vi "Auto_New.vi"() -> ()   [LabVIEW 2017]
uses:
  Control/Saurabh/prosucer_consumer_enum1.ctl
  <vilib>/Utility/error.llb/DialogType.ctl
  <vilib>/addons/database/Connection.llb/DB Tools Open Connec (String).vi
  Global/Global 1.vi
  Global/DATA LOG.vi
  <vilib>/addons/database/NI_Database_API.lvlib
panel:
  out "OP30 BARCODE STRING EMPRTY 2":bool
  out "SHIFT":string
  in  "BARCODE RECIPE":string(combo)
  out "PLC COM.":bool
  out "SHIFT_DATA":string[](array[string])
  out "OP30 BARCODE STRING EMPRTY":bool
  out "stop":bool
  out "error out 2":errorcluster
  out "Shift 4":i32
  out "Time Stamp Out":timestamp[](array[timestamp]) format="%<%X>T"
  out "Time Stamp Out 4":timestamp[](array[timestamp]) format="%<%X>T"
  out "Shift_change":bool
  out "appended array":string[][](array[string])
  out "SHIFT_DATA 2":string[](array[string])
  in  "error in (no error)":errorcluster
  in  "Tab Control":enum32{"Screen 1", "Screen 2"}(tab)
  out "OP 50":bool
  out "OP 40":bool
  out "OP 30":bool
  out "OP - 50":T1
  out "OP - 40":T2
  out "OP - 30":T3
  in  "stop 2":bool
  out "OP - 10":T4
  in  "SIMULATE INPUT":bool[](array[boolean])=[FALSE, FALSE, FALSE, FALSE]
  out "OP - 20":T5
  out "OP 10 & 20":bool
  out "OP - 110":cluster{"BARCODE":string}
  out "OP - 80":T6
  out "OP - 70":T7
  out "OP - 90":T8
  out "OP - 100":T9
  out "OP - 60":T10
  out "OP 60":bool
  out "OP 70 & 80":bool
  out "OP 90 -100 - 110":bool
  # "SENSOR MIN VLTG"
  # "Op10 20\nOp30\nOp 40\nOp50\nOp60\nOp70-80\nOp 90-100-110"
  # "OP - 50"
  # "OP - 40"
  # "OP - 30"
  # "OP - 10"
  # "OP - 20"
  # "Op10 20\nOp30\nOp 40\nOp50\nOp60\nOp70-80\nOp 90-100-110"
  # "OP - 110"
  # "OP - 80"
  # "OP - 70"
  # "OP - 90"
  # "OP - 100"
  # "OP - 60"
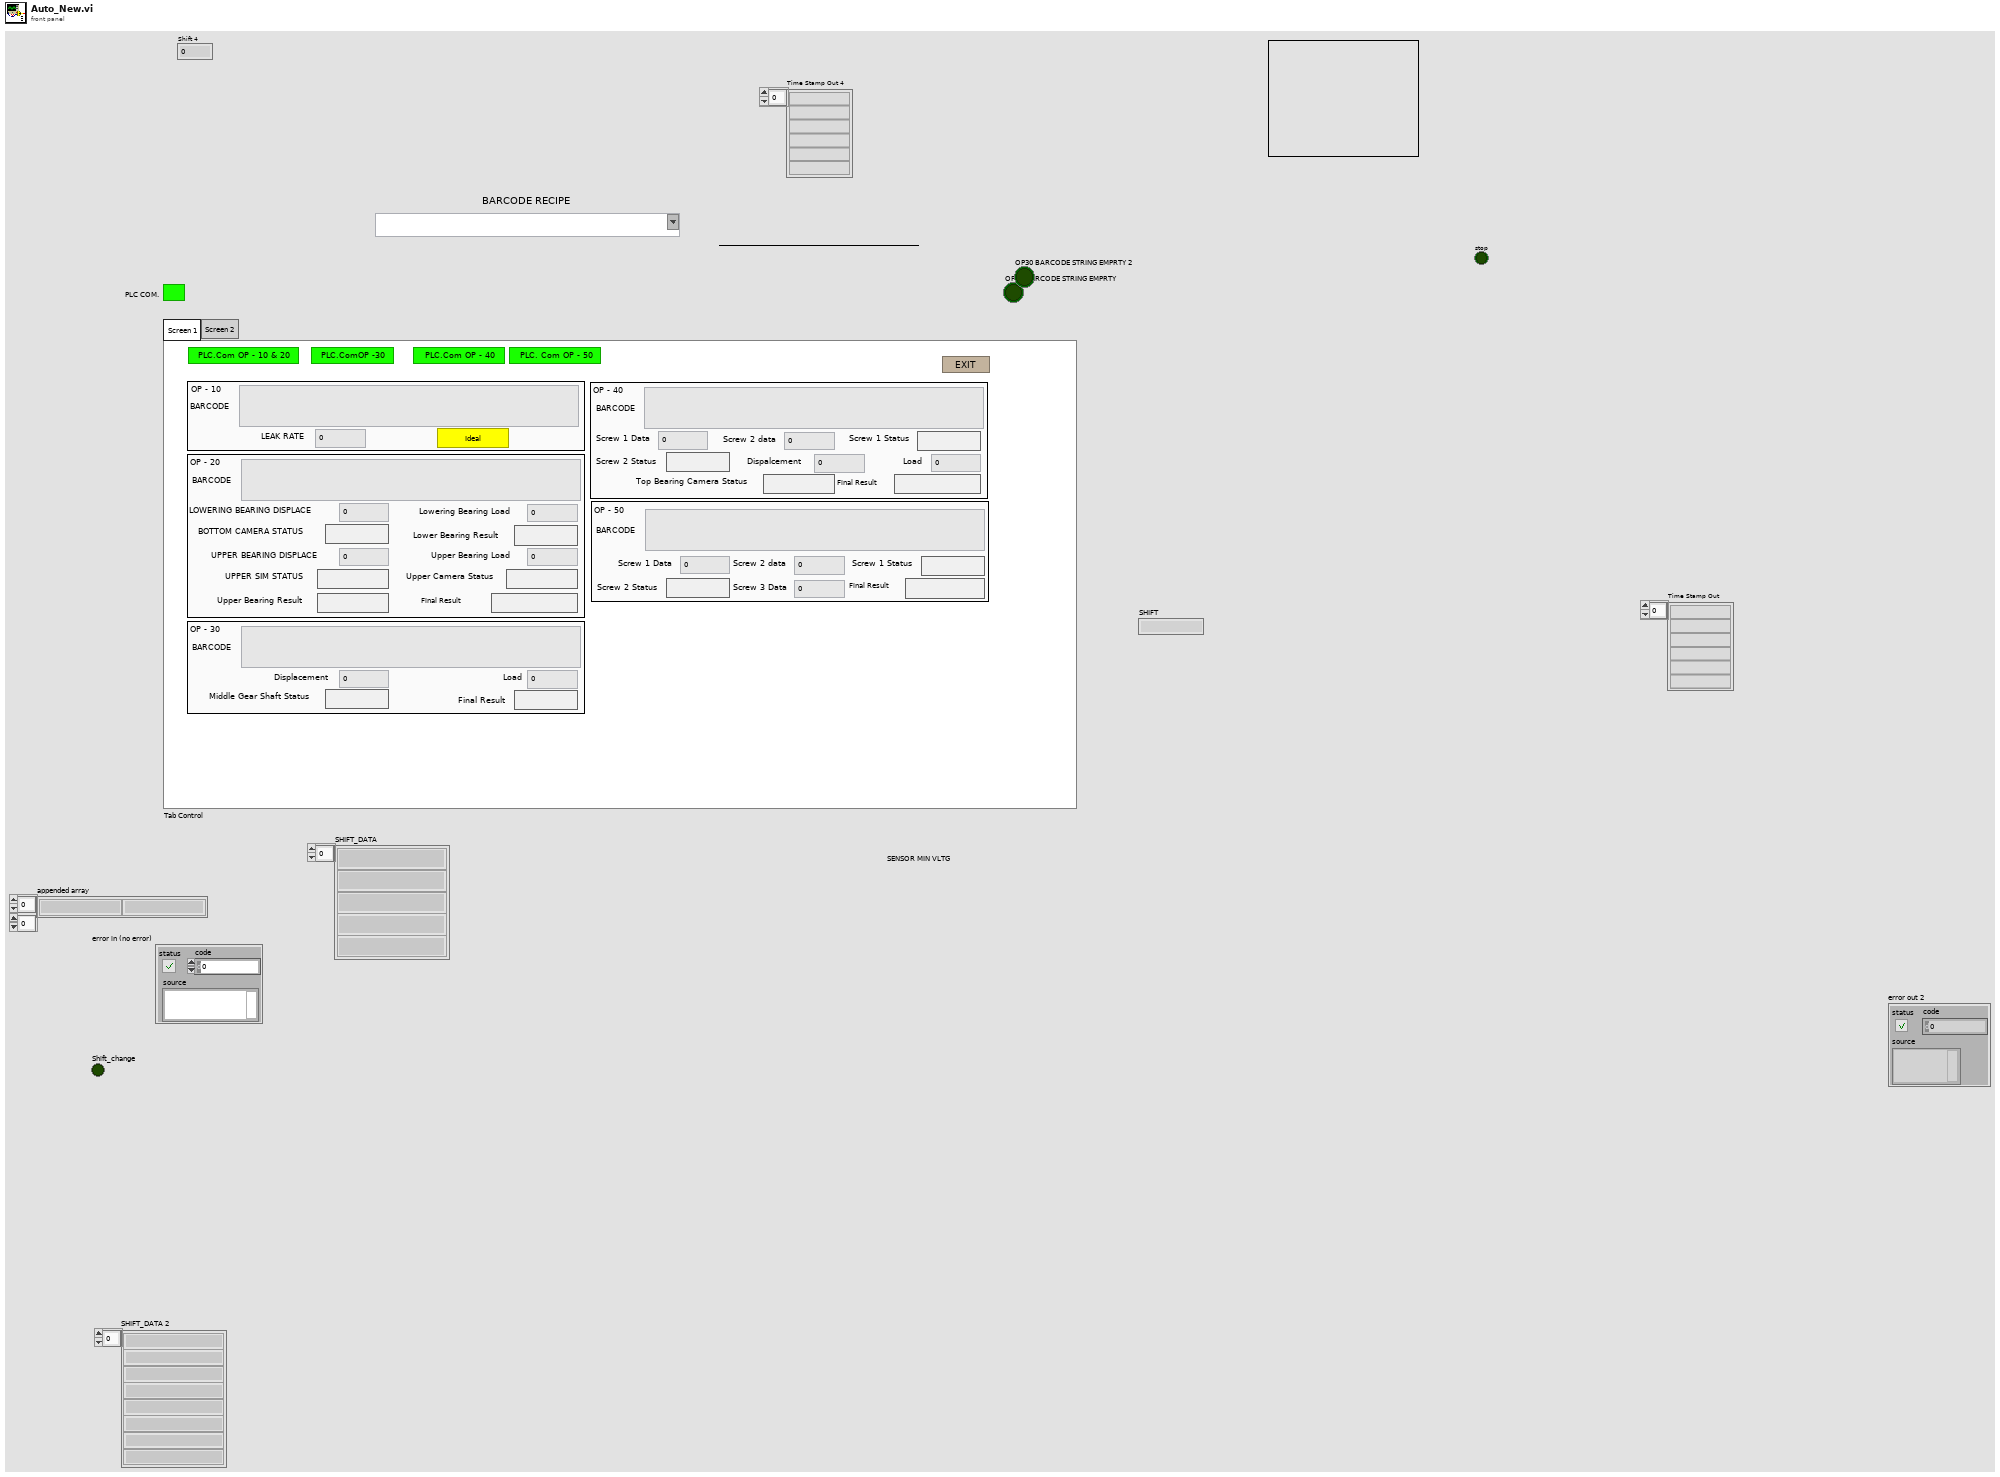
[diagram p1: front panel]
types:
  T1 = cluster{"BARCODE":string, "Screw 1 Data":dbl, "Screw 2 data":dbl, "Screw 1 Status":bool, "Screw 2 Status":bool, "Screw 3 Data":dbl, "Final Result":bool}
  T2 = cluster{"BARCODE":string, "Screw 1 Data":dbl, "Screw 2 data":dbl, "Screw 1 Status":bool, "Screw 2 Status":bool, "Dispalcement ":dbl, "Load ":dbl, "Top Bearing Camera Status":bool, "Final Result":bool}
  T3 = cluster{"BARCODE":string, "Displacement":dbl, "Load":dbl, "Middle Gear Shaft Status":bool, "Final Result":bool}
  T4 = cluster{"BARCODE":string, "LEAK RATE":dbl, "RESULT":bool}
  T5 = cluster{"BARCODE":string, "LOWERING BEARING DISPLACE":dbl, "Lowering Bearing Load":dbl, "BOTTOM CAMERA STATUS":bool, "Lower Bearing Result":bool, "UPPER BEARING DISPLACE":dbl, "Upper Bearing Load ":dbl, "UPPER SIM STATUS":bool, "Upper Camera Status":bool, "Upper Bearing Result":bool, "Final Result":bool}
  T6 = cluster{"BARCODE":string, "Load":dbl, "Final Result":bool, "Dispensing":bool}
  T7 = cluster{"BARCODE":string, "Sensor MIN Vltg":dbl, "Sensor MAX Vltg":dbl, "Final Result":bool}
  T8 = cluster{"BARCODE":string, "Seat LT Data":dbl, "Seat Status":bool, "Steam LT Data":dbl, "Final Result":bool}
  T9 = cluster{"BARCODE":string, "Sensor O/P Open V":dbl, "Start Of Close Sensor V":dbl, "Final Result":bool, "Sensor O/P Full Close V":dbl, "Response Time FWD (mSec)":dbl, "Response Time REV (mSec)":dbl, "Motor V Start Of Close A":dbl, "Motor V Full Close B R":dbl, "Motor V Start Back C":dbl, "Motor V Full Open D":dbl, "Motor RMS Current A":dbl}
  T10 = cluster{"BARCODE":string, "Screw 1 Data":dbl, "Screw 2 data":dbl, "Screw 1 Status":bool, "Screw 2 Status":bool, "Screw3 Data":dbl, "Final Result":bool, "Screw3 Status":bool, "Screw4 Data":dbl, "Screw5 Data":dbl, "Screw4 Status":bool, "Screw5 Status":bool, "Screw6 Data":dbl, "Screw6 Status":bool}
  T11 = cluster{"OP - 10":cluster{"BARCODE":string, "LEAK RATE":dbl, "RESULT":bool}, "OP - 20":cluster{"BARCODE":string, "LOWERING BEARING DISPLACE":dbl, "LOWERING BEARING LOAD":dbl, "BOTTOM CAMERA STATUS":bool, "LOWER BEARING RESULT":bool, "UPPER BEARING DISPLACE":dbl, "UPPER BEARING LOAD ":dbl, "UPPER SIM STATUS":bool, "UPPER CAMERA STATUS":bool, "UPPER BEARING RESULT":bool, "FINAL RESULT":bool}, "OP - 30":cluster{"BARCODE":string, "Displacement":dbl, "Load":dbl, "Middle Gear Shaft Status":bool, "Final Result":bool}, "OP - 40":cluster{"BARCODE":string, "Screw 1 Data":dbl, "Screw 2 data":dbl, "Screw 1 Status":bool, "Screw 2 Status":bool, "Dispalcement ":dbl, "Load ":dbl, "Top Bearing Camera Status":bool, "Final Result":bool}, "OP - 50":cluster{"BARCODE":string, "Screw 1 Data":dbl, "Screw 2 data":dbl, "Screw 1 Status":bool, "Screw 2 Status":bool, "Screw 3 Data":dbl, "Final Result":bool}, "OP - 60":cluster{"BARCODE":string, "Screw 1 Data":dbl, "Screw 2 data":dbl, "Screw 1 Status":bool, "Screw 2 Status":bool, "Screw3 Data":dbl, "Final Result":bool, "Screw3 Status":bool, "Screw4 Data":dbl, "Screw5 Data":dbl, "Screw4 Status":bool, "Screw5 Status":bool, "Screw6 Data":dbl, "Screw6 Status":bool}, "OP - 70":cluster{"BARCODE":string, "Sensor MIN Vltg":dbl, "Sensor MAX Vltg":dbl, "Final Result":bool}, "OP - 80":cluster{"BARCODE":string, "Load":dbl, "Final Result":bool, "Dispensing":bool}, "OP - 90":cluster{"BARCODE":string, "Seat LT Data":dbl, "Seat Status":bool, "Steam LT Data":dbl, "Final Result":bool}, "OP - 100":cluster{"BARCODE":string, "Sensor O/P Open V":dbl, "Start Of Close Sensor V":dbl, "Final Result":bool, "Sensor O/P Full Close V":dbl, "Response Time FWD (mSec)":dbl, "Response Time REV (mSec)":dbl, "Motor V Start Of Close A":dbl, "Motor V Full Close B R":dbl, "Motor V Start Back C":dbl, "Motor V Full Open D":dbl, "Motor RMS Current A":dbl}, "OP - 110":cluster{"BARCODE":string}}
  T12 = typedef "prosucer_consumer_enum1.ctl" = enum16{"SCAN1", "SCAN2", "SCAN3", "SCAN4", "SCAN5", "SCAN6", "SCAN7", "SCAN8", "SCAN9", "SCAN10", "SCAN11", "STOP", "DATALOG1", "DATALOG2", "DATALOG3", "DATALOG4", "DATALOG5", "DATALOG6", "DATALOG7", "DATALOG8", "DATALOG9", "DATALOG10", "DATALOG11", "-1", "CYCLE_START1", "CYCLE_START2", "CYCLE_START3", "CYCLE_START4", "BARCODE RECIPE", "EMERGENCY STOP"}
  T13 = typedef "NI_Database_API.lvlib/Conn ObjectReference.ctl" = refnum<k1>
  T14 = typedef "DialogType.ctl" = u16
  T15 = cluster{"trimmed string":string, "SHIFT":string, "date/time string":string, string, "Input 2":string}
  T16 = cluster{"SHIFT":string, "date/time string":string, "Input 2":string, string}
  T17 = cluster{"Input 2":string, "Input 2":string, "Input 2":string, "Input 2":string, "Input 2":string, "Input 2":string, "Input 2":string, "Input 2":string, "Input 2":string, "Input 2":string}
  T18 = cluster{"date/time string":string, "SHIFT":string, "Input 2":string, "Input 2":string, "Input 2":string, "Input 2":string, "Input 2":string, "Input 2":string, "Input 2":string, "Input 2":string, "Input 2":string, "Input 2":string}
  T19 = cluster{"Input 2":string, "Input 2":string, "Input 2":string, "Input 2":string}
  T20 = cluster{"date/time string":string, "SHIFT":string, "Input 2":string, "Input 2":string, "Input 2":string, "Input 2":string}
  T21 = cluster{"Input 2":string, "Input 2":string, "Input 2":string, "Input 2":string, "Input 2":string, "Input 2":string, "Input 2":string, "Input 2":string}
  T22 = cluster{"date/time string":string, "SHIFT":string, "Input 2":string, "Input 2":string, "Input 2":string, "Input 2":string, "Input 2":string, "Input 2":string, "Input 2":string, "Input 2":string}
  T23 = cluster{"Input 2":string, "Input 2":string, "Input 2":string, "Input 2":string, "Input 2":string, "Input 2":string}
  T24 = cluster{"date/time string":string, "SHIFT":string, "Input 2":string, "Input 2":string, "Input 2":string, "Input 2":string, "Input 2":string, "Input 2":string}
  T25 = cluster{"Input 2":string, "Input 2":string, "Input 2":string, "Input 2":string, "Input 2":string, "Input 2":string, "Input 2":string, "Input 2":string, "Input 2":string, "Input 2":string, "Input 2":string, "Input 2":string}
  T26 = cluster{"date/time string":string, "SHIFT":string, "Input 2":string, "Input 2":string, "Input 2":string, "Input 2":string, "Input 2":string, "Input 2":string, "Input 2":string, "Input 2":string, "Input 2":string, "Input 2":string, "Input 2":string, "Input 2":string}
  T27 = cluster{"Input 2":string, "Input 2":string, "Input 2":string}
  T28 = cluster{"date/time string":string, "SHIFT":string, "Input 2":string, "Input 2":string, "Input 2":string}
  T29 = cluster{"Input 2":string, "Input 2":string, "Input 2":string, "time string":string, "time string":string, "Input 2":string, "Input 2":string, "Input 2":string, "Input 2":string, "Input 2":string, "Input 2":string, "Input 2":string}
  T30 = cluster{"date/time string":string, "SHIFT":string, "Input 2":string, "Input 2":string, "Input 2":string, "time string":string, "time string":string, "Input 2":string, "Input 2":string, "Input 2":string, "Input 2":string, "Input 2":string, "Input 2":string, "Input 2":string}
  T31 = cluster{"BARCODE":string, "LOWERING BEARING DISPLACE":dbl, "LOWERING BEARING LOAD":dbl, "BOTTOM CAMERA STATUS":bool, "LOWER BEARING RESULT":bool, "UPPER BEARING DISPLACE":dbl, "UPPER BEARING LOAD ":dbl, "UPPER SIM STATUS":bool, "UPPER CAMERA STATUS":bool, "UPPER BEARING RESULT":bool, "FINAL RESULT":bool}
  T32 = enum32{"invalid app kind", "Development System", "Run Time System", "Student Edition", "Embedded LabVIEW", "Evaluation", "Custom"}
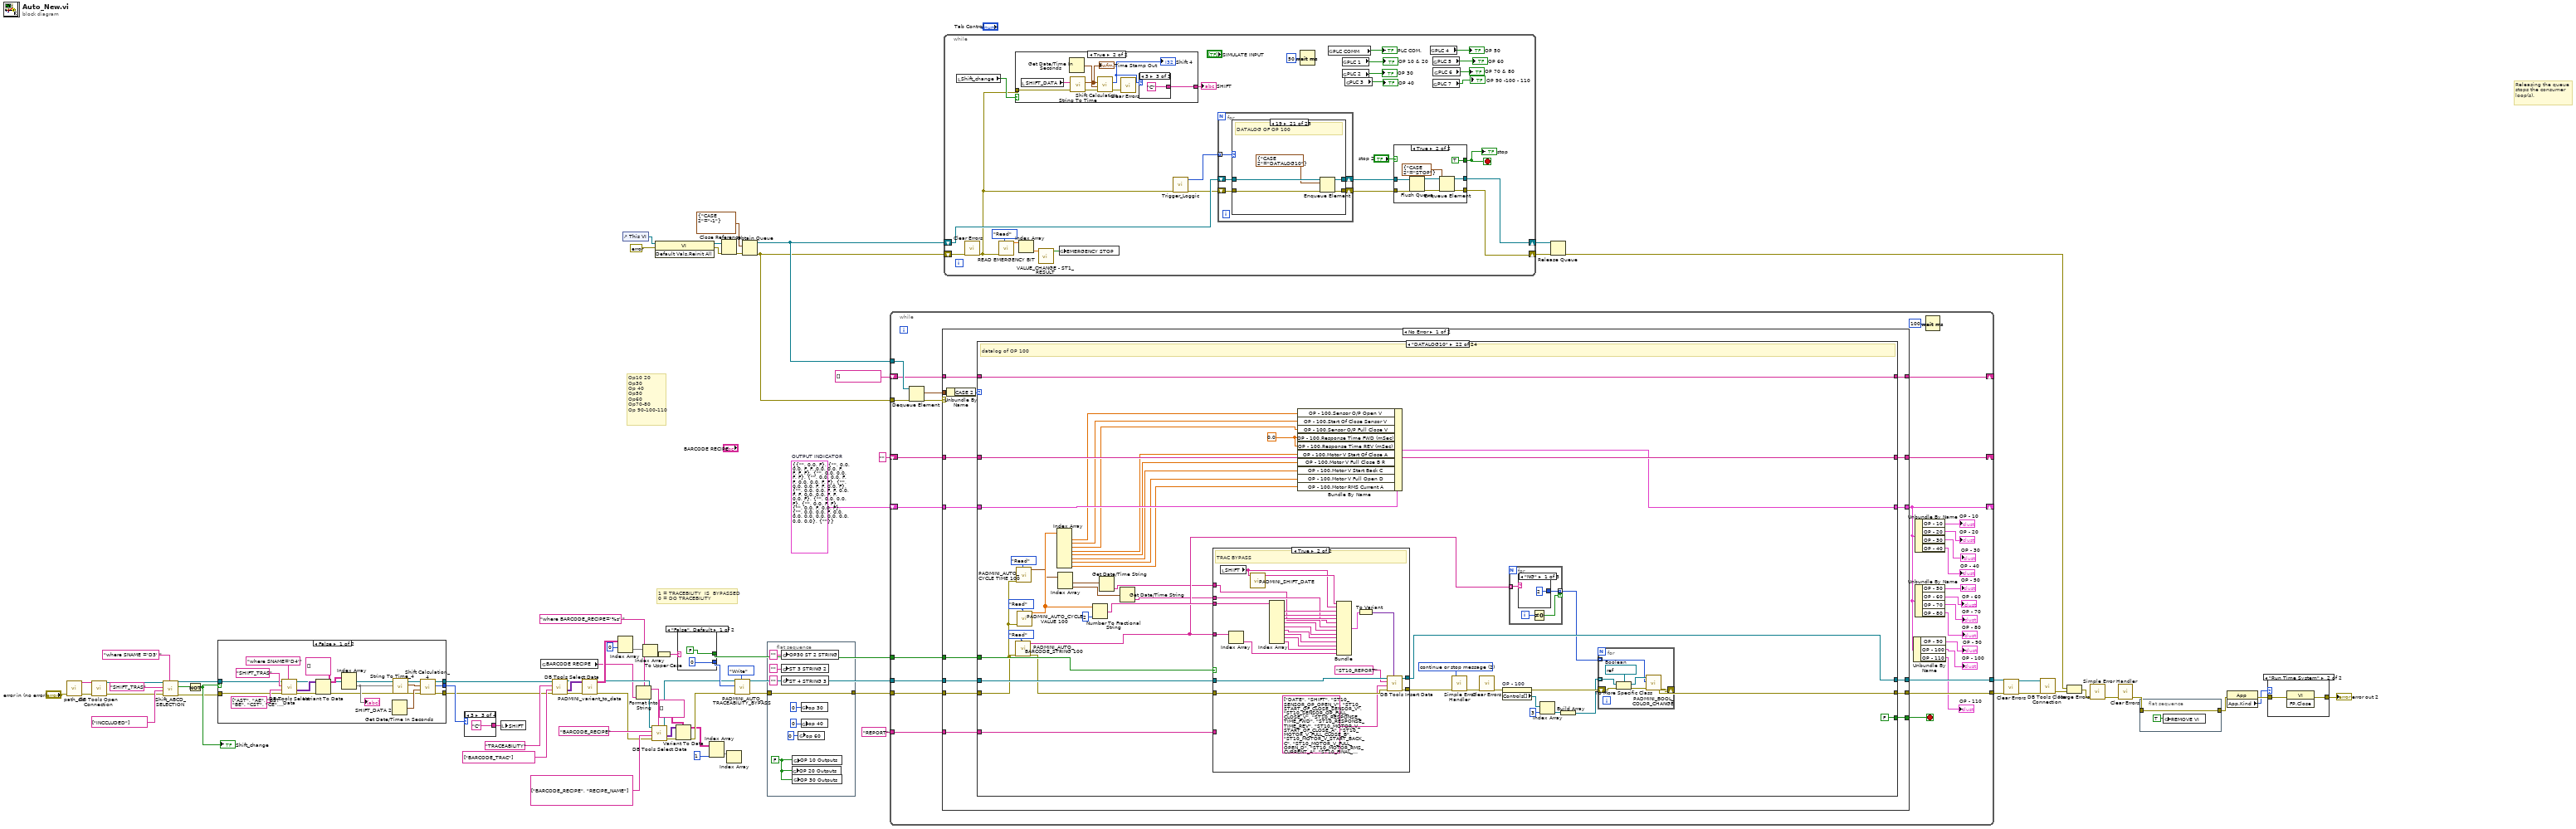
[diagram p0: block diagram]
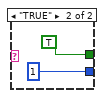
[diagram p2: hidden frame]
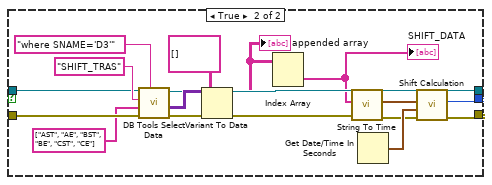
[diagram p3: hidden frame]
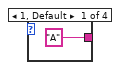
[diagram p4: hidden frame]
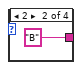
[diagram p5: hidden frame]
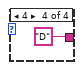
[diagram p6: hidden frame]
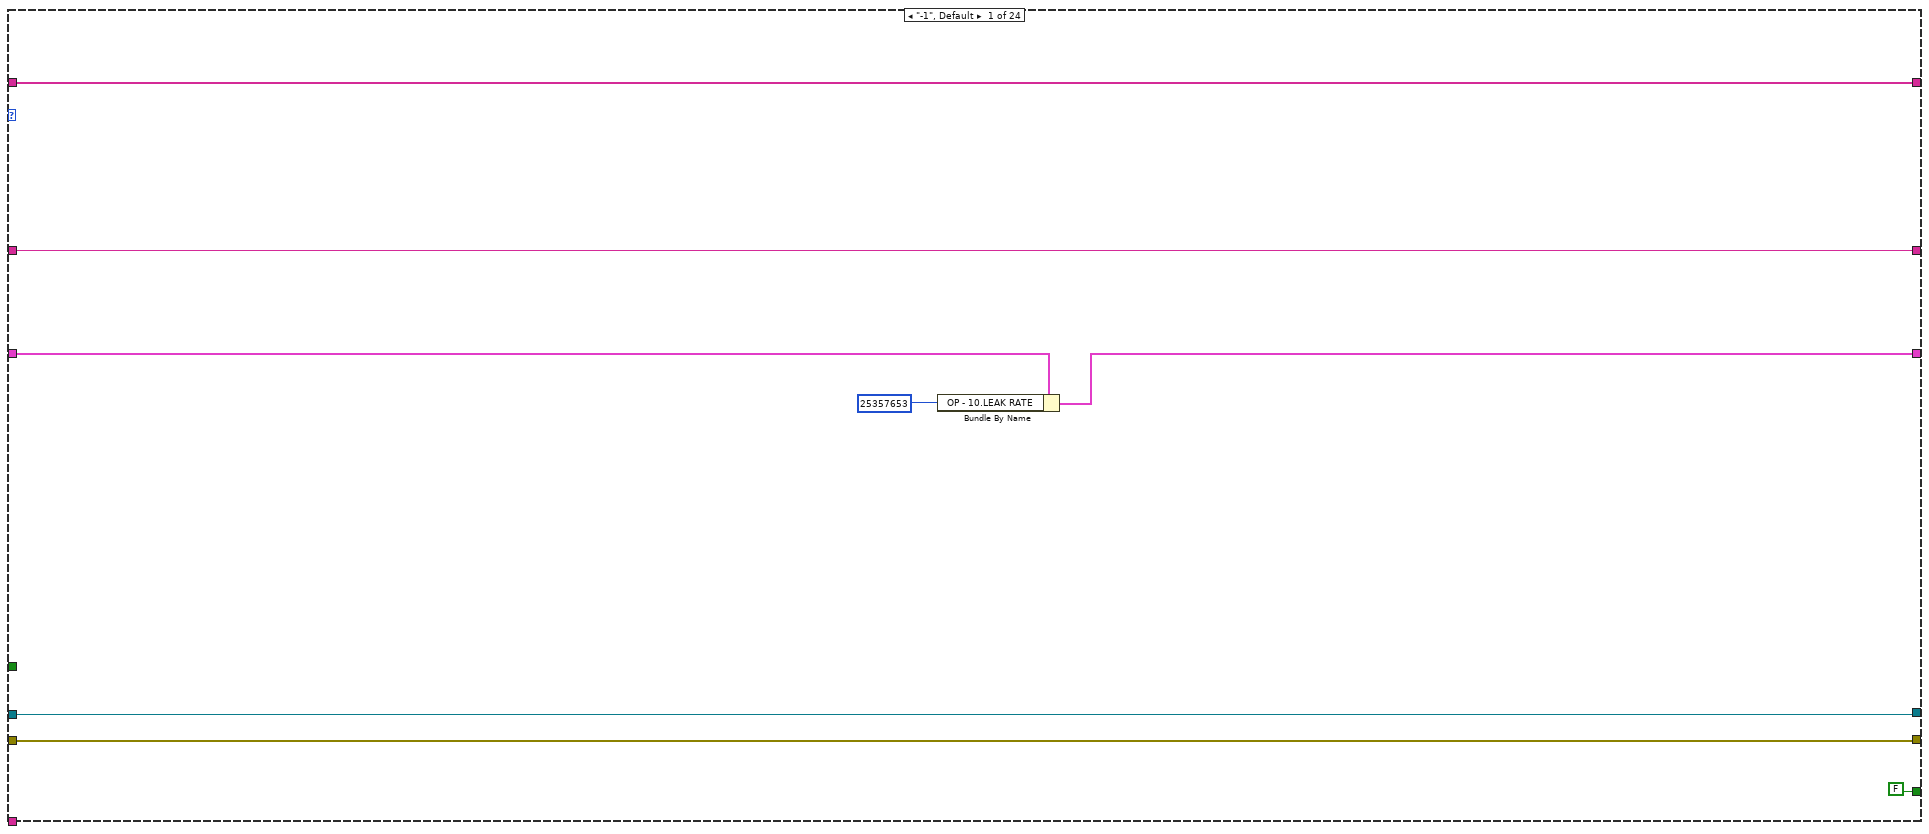
[diagram p7: hidden frame]
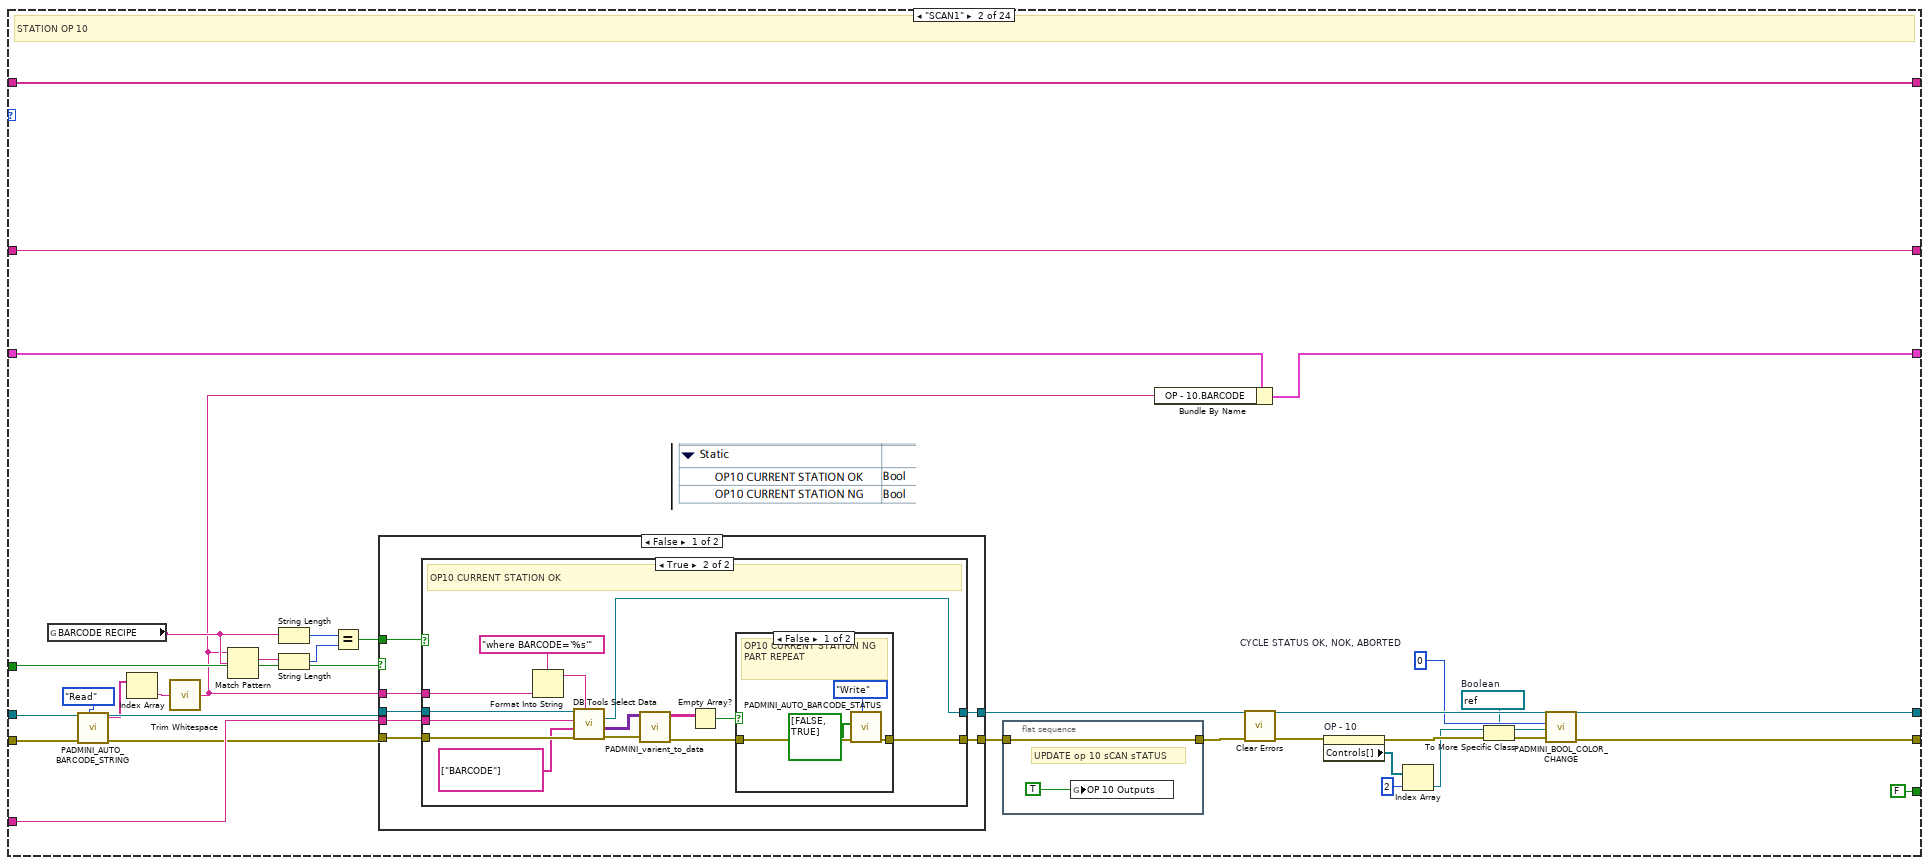
[diagram p8: hidden frame]
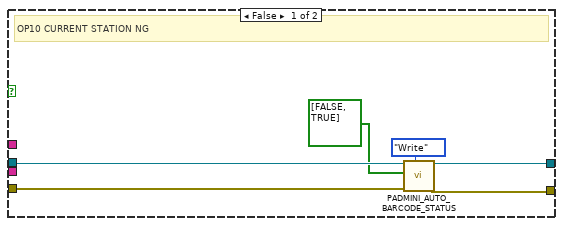
[diagram p9: hidden frame]
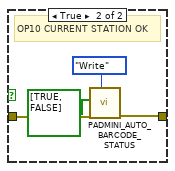
[diagram p10: hidden frame]
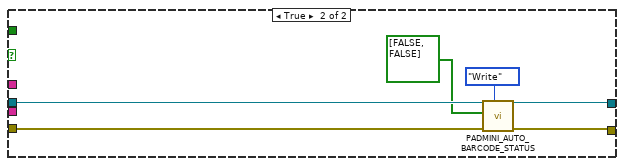
[diagram p11: hidden frame]
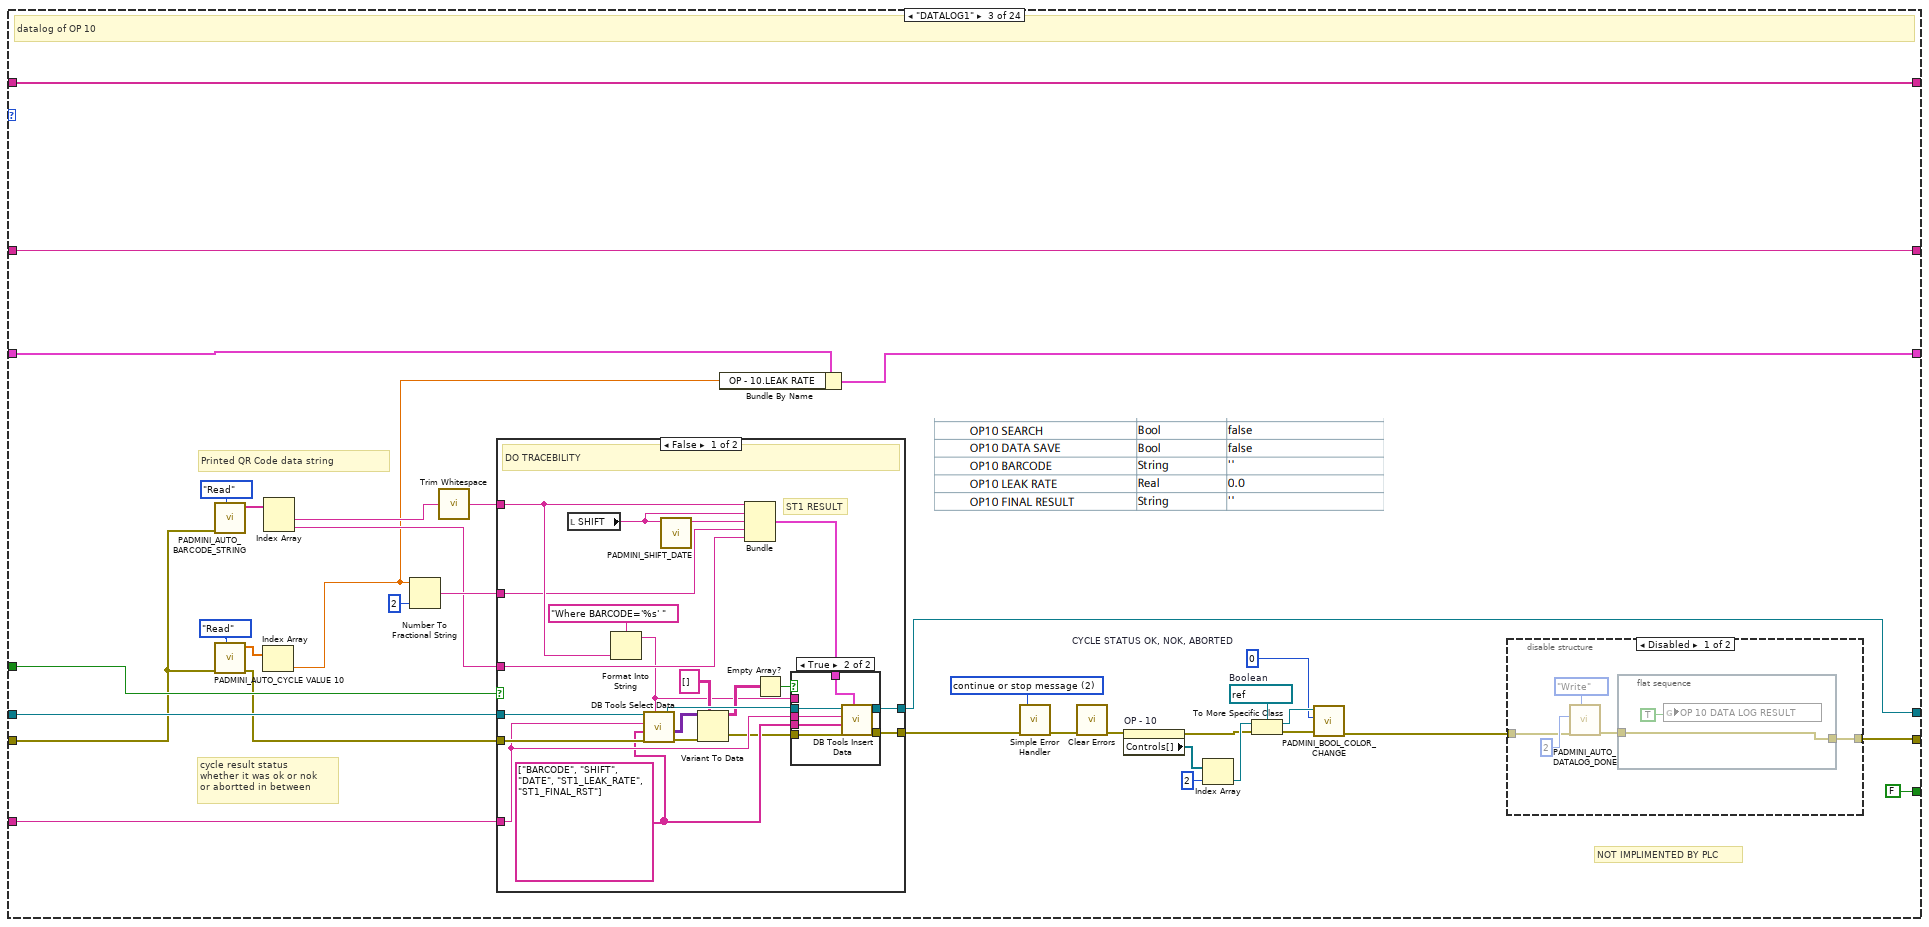
[diagram p12: hidden frame]
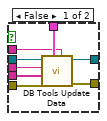
[diagram p14: hidden frame]
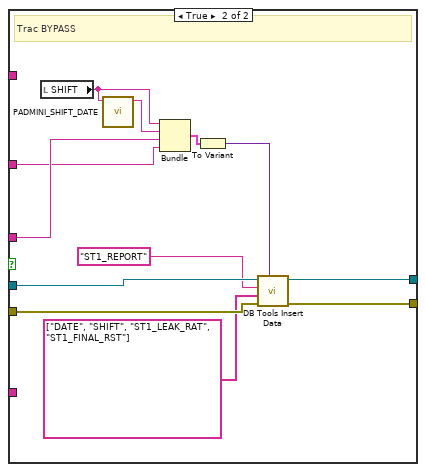
[diagram p15: hidden frame]
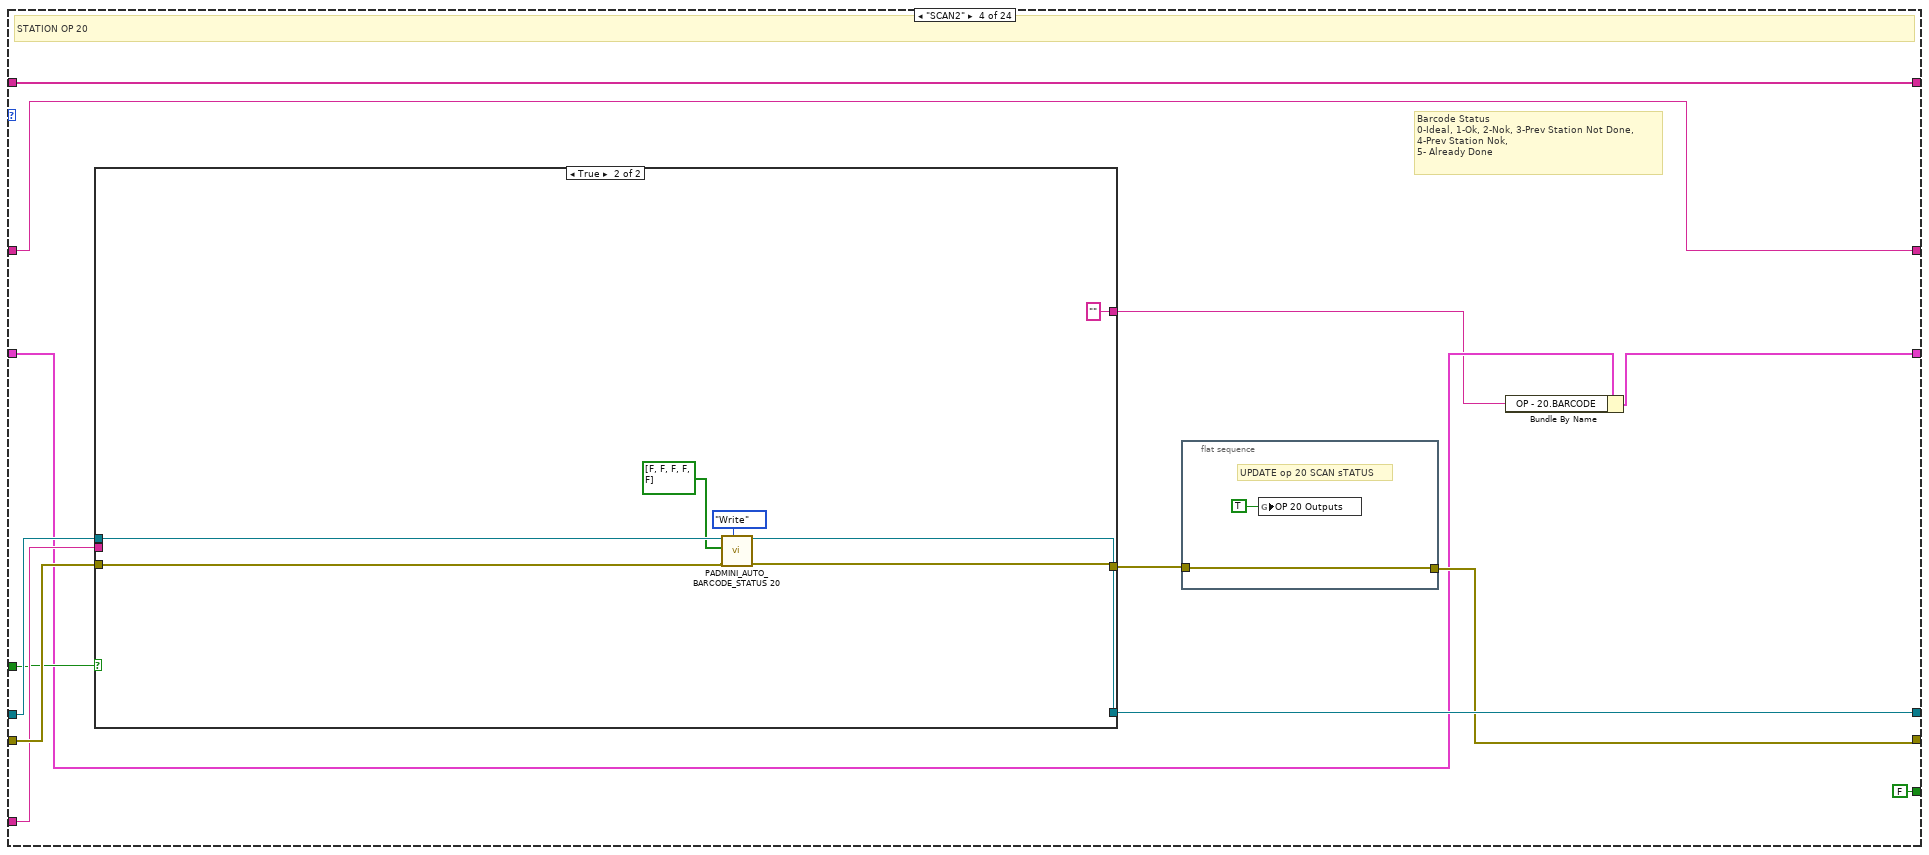
[diagram p16: hidden frame]
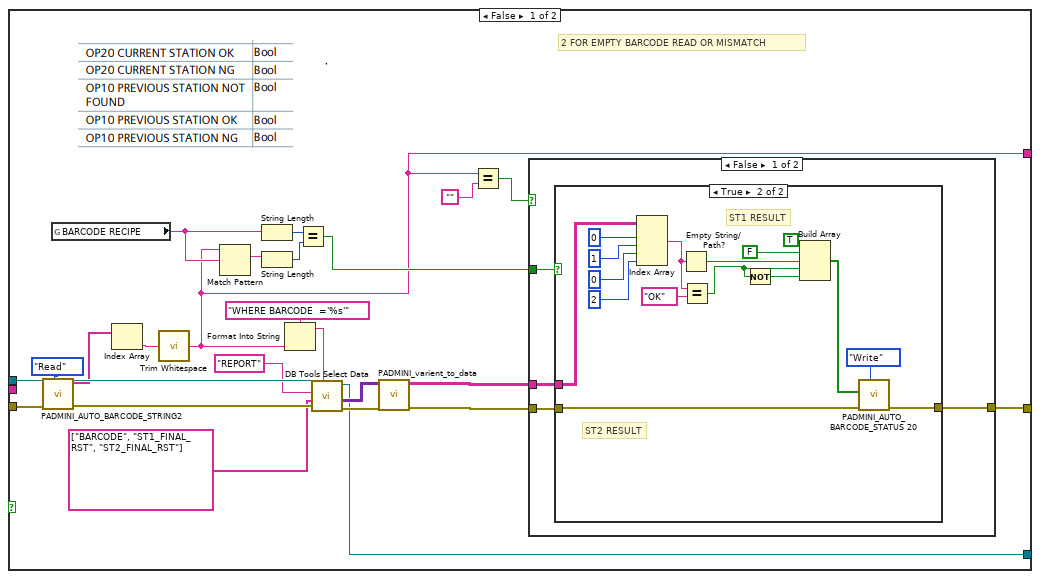
[diagram p17: hidden frame]
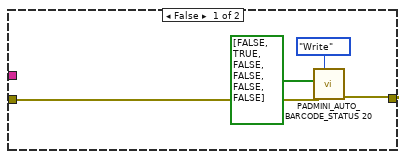
[diagram p18: hidden frame]
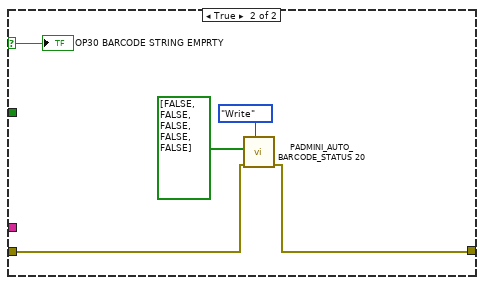
[diagram p19: hidden frame]
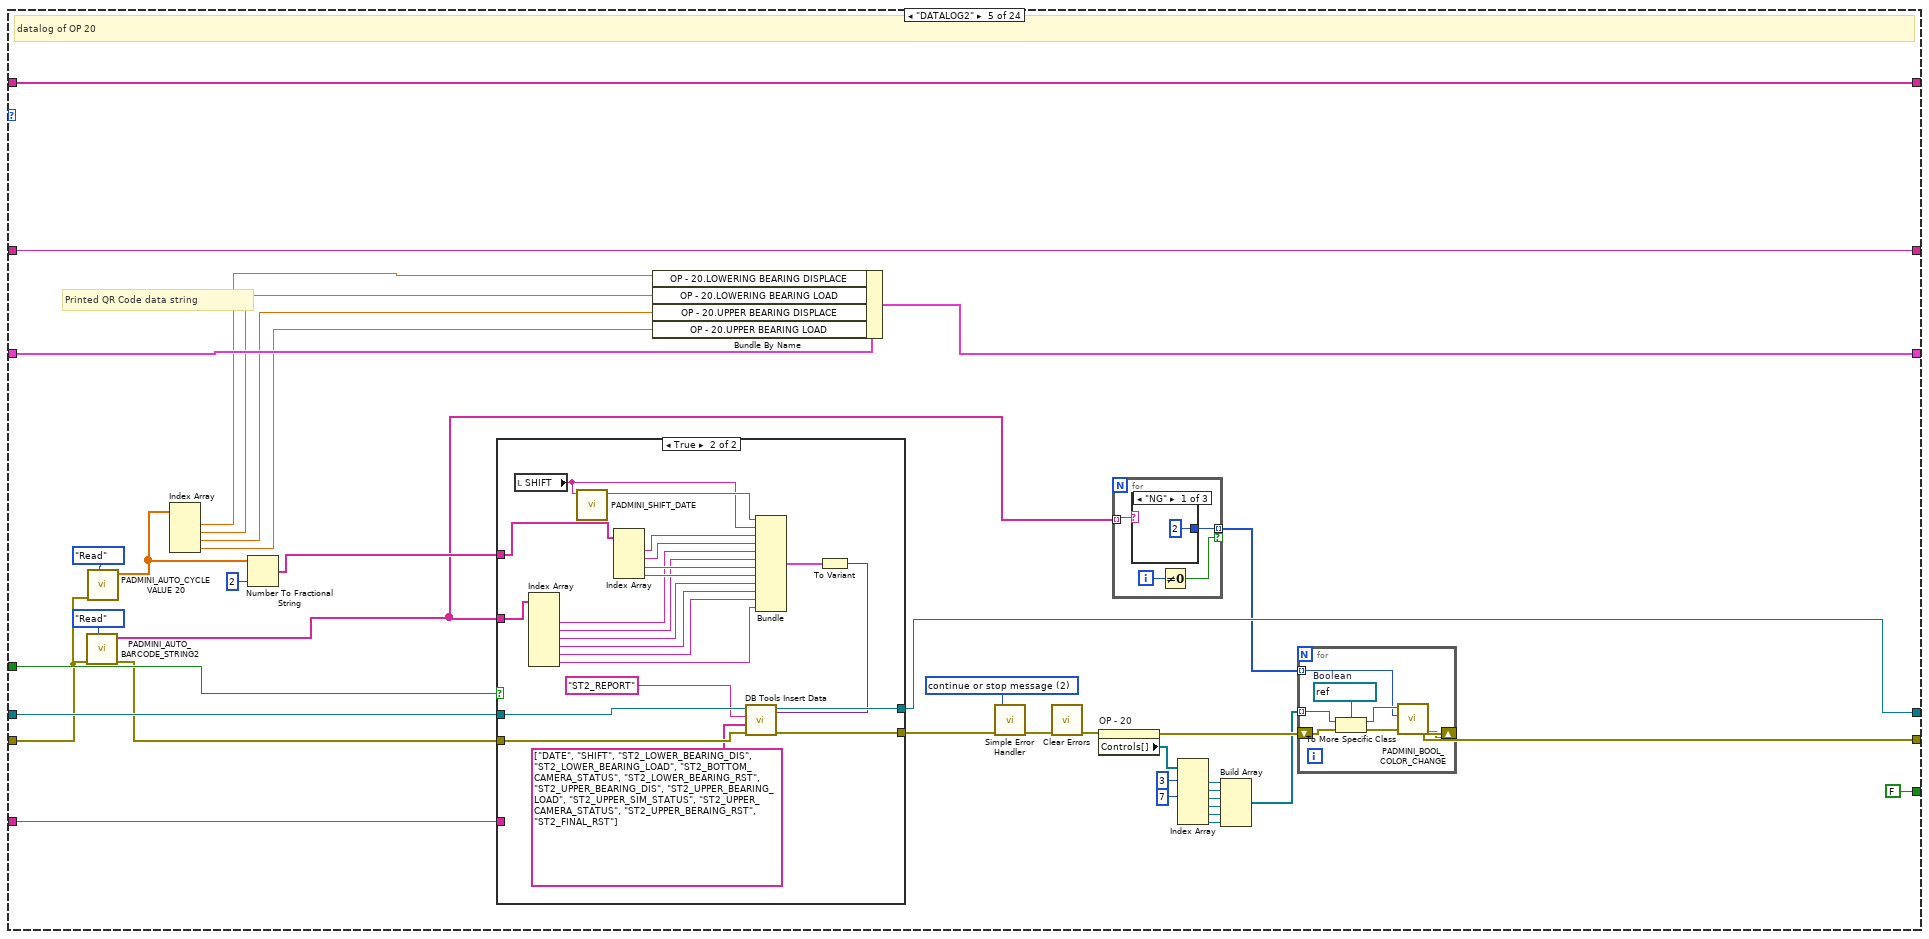
[diagram p20: hidden frame]
diagram:
  w2 = T11 {"OP - 10"={"BARCODE"="", "LEAK RATE"=0.0, "RESULT"=FALSE}, "OP - 20"={"BARCODE"="", "LOWERING BEARING DISPLACE"=0.0, "LOWERING BEARING LOAD"=0.0, "BOTTOM CAMERA STATUS"=FALSE, "LOWER BEARING RESULT"=FALSE, "UPPER BEARING DISPLACE"=0.0, "UPPER BEARING LOAD "=0.0, "UPPER SIM STATUS"=FALSE, "UPPER CAMERA STATUS"=FALSE, "UPPER BEARING RESULT"=FALSE, "FINAL RESULT"=FALSE}, "OP - 30"={"BARCODE"="", "Displacement"=0.0, "Load"=0.0, "Middle Gear Shaft Status"=FALSE, "Final Result"=FALSE}, "OP - 40"={"BARCODE"="", "Screw 1 Data"=0.0, "Screw 2 data"=0.0, "Screw 1 Status"=FALSE, "Screw 2 Status"=FALSE, "Dispalcement "=0.0, "Load "=0.0, "Top Bearing Camera Status"=FALSE, "Final Result"=FALSE}, "OP - 50"={"BARCODE"="", "Screw 1 Data"=0.0, "Screw 2 data"=0.0, "Screw 1 Status"=FALSE, "Screw 2 Status"=FALSE, "Screw 3 Data"=0.0, "Final Result"=FALSE}, "OP - 60"={"BARCODE"="", "Screw 1 Data"=0.0, "Screw 2 data"=0.0, "Screw 1 Status"=FALSE, "Screw 2 Status"=FALSE, "Screw3 Data"=0.0, "Final Result"=FALSE, "Screw3 Status"=FALSE, "Screw4 Data"=0.0, "Screw5 Data"=0.0, "Screw4 Status"=FALSE, "Screw5 Status"=FALSE, "Screw6 Data"=0.0, "Screw6 Status"=FALSE}, "OP - 70"={"BARCODE"="", "Sensor MIN Vltg"=0.0, "Sensor MAX Vltg"=0.0, "Final Result"=FALSE}, "OP - 80"={"BARCODE"="", "Load"=0.0, "Final Result"=FALSE, "Dispensing"=FALSE}, "OP - 90"={"BARCODE"="", "Seat LT Data"=0.0, "Seat Status"=FALSE, "Steam LT Data"=0.0, "Final Result"=FALSE}, "OP - 100"={"BARCODE"="", "Sensor O/P Open V"=0.0, "Start Of Close Sensor V"=0.0, "Final Result"=FALSE, "Sensor O/P Full Close V"=0.0, "Response Time FWD (mSec)"=0.0, "Response Time REV (mSec)"=0.0, "Motor V Start Of Close A"=0.0, "Motor V Full Close B R"=0.0, "Motor V Start Back C"=0.0, "Motor V Full Open D"=0.0, "Motor RMS Current A"=0.0}, "OP - 110"={"BARCODE"=""}}  # OUTPUT INDICATOR
  # "Op10 20\nOp30\nOp 40\nOp50\nOp60\nOp70-80\nOp 90-100-110"
  # "1 = TRACEBILITY  IS  BYPASSED\n0 = DO TRACEBILITY"
  # "Releasing the queue stops the consumer loop(s)."
  n1 = call "path_db.vi"("error in"="error in (no error)") -> ("error out"=w47:errorcluster, "resulting string"=w68:string)  [unwired: 9 in]
  n2 = call-poly <vilib>:"DB Tools Open Connection.vi"("error in (no error)"=w47, "connection information"=w68) -> ("error out"=w46:errorcluster, "connection reference"=w39:T13)  [unwired: 6 in]
  n3 = call "Shift_ABCD_SELECTION.vi"("Where"="where SNAME ='D3' ", "error in (no error)"=w46, "Array"=string[] ["INCCLUDED"], "table"="SHIFT_TRAS", "Refnum in"=w39) -> ("error out"=w1:errorcluster, "Boolean"=w59:bool, "Refnum out"=w60:T13)  [unwired: 4 in]
  n4 = Not(x=w59) -> (.not. x?=w58:bool)
  "Shift_change" <- w58
  n5 = case shown="False" w58 {
    tunnel: [w73 w97] -> w64
    tunnel: w60 -> [w76 w95]
    tunnel: w1 -> [w75 w94]
    tunnel: [w74 w93] -> w28
    tunnel: [w72 w87] -> w27
    frame False {
      n6 = call <vilib>:"DB Tools Select Data.vi"("condition"="where SNAME='D4'", "error in (no error)"=w75, "columns"=string[] ["AST", "AE", "BST", "BE", "CST", "CE", "DST", "DE"], "table"="SHIFT_TRAS", "connection reference"=w76) -> ("error out"=w82:errorcluster, "data"=w86:variant[][], "connection reference out"=w74:T13)  [unwired: 1 in]
      n7 = Variant To Data(error in=w82, type=string[][] [], Variant=w86) -> (data=w79:string[][], error out=w72:errorcluster)
      n8 = Index Array(array=w79) -> (element=w78:string[])  [unwired: 2 in]
      "SHIFT_DATA 2" <- w78
      n9 = Get Date/Time In Seconds() -> (seconds since 1Jan1904=w81:timestamp)
      n10 = call "String To Time_4.vi"("String Array In"=w78) -> ("Time Stamp Out"=w77:timestamp[])  [unwired: 9 in, 1 out]
      n11 = call "Shift Calculation_4.vi"("Current Time"=w81, "Time Stamp Out"=w77) -> ("Shift"=w73:i32)  [unwired: 8 in, 1 out]
    }
    frame True {
      n12 = call <vilib>:"DB Tools Select Data.vi"("condition"="where SNAME='D3'", "error in (no error)"=w94, "columns"=string[] ["AST", "AE", "BST", "BE", "CST", "CE"], "table"="SHIFT_TRAS", "connection reference"=w95) -> ("error out"=w99:errorcluster, "data"=w103:variant[][], "connection reference out"=w93:T13)  [unwired: 1 in]
      n13 = Variant To Data(error in=w99, type=string[][] [], Variant=w103) -> (data=w91:string[][], error out=w89:errorcluster)
      "appended array" <- w91
      n14 = Index Array(array=w91) -> (element=w90:string[])  [unwired: 2 in]
      "SHIFT_DATA" <- w90
      n15 = call "String To Time.vi"("error in (no error)"=w89, "String Array In"=w90) -> ("error out"=w88:errorcluster, "Time Stamp Out"=w96:timestamp[])  [unwired: 8 in]
      n16 = Get Date/Time In Seconds() -> (seconds since 1Jan1904=w98:timestamp)
      n17 = call "Shift Calculation.vi"("error in (no error)"=w88, "Current Time"=w98, "Time Stamp Out"=w96) -> ("error out"=w87:errorcluster, "Shift"=w97:i32)  [unwired: 7 in]
    }
  }
  n18 = case shown="3" w64 {
    tunnel: ["A" "B" "C" "D"] -> w57
    frame 1, Default {
    }
    frame 2 {
    }
    frame 3 {
    }
    frame 4 {
    }
  }
  n19 = local write "SHIFT"(w57) -> ()
  n20 = global read "Global 1.vi" "BARCODE RECIPE"() -> (w8:string)
  n21 = call <vilib>:"DB Tools Select Data.vi"("error in (no error)"=w27, "columns"=string[] ["BARCODE_TRAC"], "table"="TRACEABILITY", "connection reference"=w28) -> ("error out"=w37:errorcluster, "data"=w36:variant[][], "connection reference out"=w14:T13)  [unwired: 2 in]
  n22 = call "PADMINI_varient_to_data.vi"("error in (no error)"=w37, "data"=w36) -> ("error out"=w12:errorcluster, "Array"=w35:string[][])  [unwired: 8 in]
  n23 = Index Array(array=w35, index (row)=0 ("disabled index (col)")) -> (element=w34:string[])  [unwired: 1 in]
  n24 = control-ref of="This VI"() -> (w44:refnum<vi>)
  n25 = Format Into String(format string="where BARCODE_RECIPE='%s' ", w8) -> (resulting string=w6:string)  [unwired: 2 in, 1 out]
  n26 = Index Array(array=w34) -> (element=w30:string)  [unwired: 1 in]
  n27 = call <vilib>:"DB Tools Select Data.vi"("condition"=w6, "error in (no error)"=w12, "columns"=string[] ["BARCODE_RECIPE", "RECIPE_NAME"], "table"="BARCODE_RECIPE", "connection reference"=w14) -> ("error out"=w16:errorcluster, "data"=w15:variant[][], "connection reference out"=w13:T13)  [unwired: 1 in]
  n28 = invoke class="VI" method="Default Vals.Reinit All"(reference=w44, error in=errorcluster {"status"=FALSE, "code"=0, "source"=""} ("error in (no error)")) -> (reference out=w42:refnum<vi>, error out=w43:errorcluster)  [unwired: 1 in, 1 out]
  n29 = To Upper Case(1:w30) -> (0:w29:string)
  n30 = Variant To Data(error in=w16, type=string[][] [], Variant=w15) -> (data=w9:string[][], error out=w11:errorcluster)
  n31 = case shown="\"False\", Default" w29 {
    tunnel: [FALSE ("BARCODE TRACEABILITY") TRUE ("BARCODE TRACEABILITY")] -> w19
    tunnel: [0 1] -> w25
    frame "False", Default {
    }
    frame "TRUE" {
    }
  }
  n32 = Index Array(array=w9, index (col)=1 ("disabled index (col)")) -> (element=w4:string[])  [unwired: 1 in]
  n33 = Close Reference(reference=w42, error in (no error)=w43) -> (error out=w40:errorcluster)
  n34 = Index Array(array=w4) -> ()  [unwired: 1 in, 1 out]
  n35 = call "PADMINI_AUTO_TRACEABILITY_BYPASS.vi"("Enum"=enum16{"Read", "Write"}."Write", "error in (no error)"=w11, "I/P"=w25) -> ("error out"=w23:errorcluster)  [unwired: 7 in, 1 out]
  n36 = Obtain Queue(element data type=cluster{"CASE 2":T12} {"CASE 2"=enum."-1"}, error in (no error)=w40) -> (queue out=w69:refnum<queue>, error out=w20:errorcluster)  [unwired: 3 in, 1 out]
  n37 = flat-sequence {
    tunnel: w23 -> [w116]
    tunnel: [w116] -> w22
    frame #0 {
      w112 = FALSE
      n38 = global write "DATA LOG.vi" "OP30 ST 2 STRING"("" ("OP30 ST 2 STRING")) -> ()
      n39 = global write "DATA LOG.vi" "ST 3 STRING 2"("" ("ST 3 STRING 2")) -> ()
      n40 = global write "DATA LOG.vi" "ST 4 STRING 3"("" ("ST 4 STRING 3")) -> ()
      n41 = global write "DATA LOG.vi" "OP 20 Outputs"(w112) -> ()
      n42 = global write "DATA LOG.vi" "OP 10 Outputs"(w112) -> ()
      n43 = global write "DATA LOG.vi" "OP 30 Outputs"(w112) -> ()
      n44 = global write "DATA LOG.vi" "op 60"(0 ("op 30")) -> ()
      n45 = global write "DATA LOG.vi" "op 30"(0 ("op 30")) -> ()
      n46 = global write "DATA LOG.vi" "op 40"(0 ("op 30")) -> ()
    }
  }
  n47 = while {
    tunnel: w69 -> [w148]
    tunnel: w20 -> [w144]
    tunnel: w22 -> [w143]
    tunnel: w13 -> [w142]
    tunnel: [w141] -> w67
    tunnel: [w140] -> w66
    tunnel: w19 -> [w139]
    tunnel: "REPORT" -> [w138]
    shift-right: [w136] -> _
    shift-left: string[] [] -> [w137]
    shift-right: [w135] -> _
    shift-left: "" ("trimmed string") -> [w134]
    shift-right: [w123] -> _
    shift-left: w2 -> [w132]
    stop <- w145 stop-if-true
    n48 = Dequeue Element(queue=w148, error in (no error)=w144) -> (element=w146:cluster{"CASE 2":T12}, error out=w147:errorcluster)  [unwired: 1 in, 2 out]
    n49 = case shown="No Error" w147 {
      tunnel: w146 -> [w163 _]
      tunnel: [w159 TRUE] -> w145
      tunnel: w143 -> [w160 w1892]
      tunnel: w142 -> [w161 w1891]
      tunnel: [w157 w1892] -> w141
      tunnel: [w158 w1891] -> w140
      tunnel: w139 -> [w156 _]
      tunnel: w138 -> [w155 _]
      tunnel: w137 -> [w154 w1890]
      tunnel: [w153 w1890] -> w136
      tunnel: [w152 w1889] -> w135
      tunnel: w134 -> [w151 w1889]
      tunnel: w132 -> [w150 w1888]
      tunnel: [w149 w1888] -> w123
      frame No Error {
        n50 = Unbundle By Name(w163) -> ("CASE 2"=w162:T12)
        n51 = case shown="\"DATALOG10\"" w162 {
          tunnel: w161 -> [w170 w202 w278 w348 w446 w520 w613 w675 w772 w842 w936 w1002 w1107 w1185 w1274 w1333 w1423 w1482 w1573 w1634 w1705 w1806 w1875 w1883]
          tunnel: w160 -> [w169 w198 w245 w347 w427 w519 w594 w674 w753 w841 w917 w1001 w1088 w1184 w1255 w1332 w1404 w1481 w1554 w1633 w1704 w1771 w1874 w1885]
          tunnel: [FALSE FALSE FALSE FALSE FALSE FALSE FALSE FALSE FALSE FALSE FALSE FALSE FALSE FALSE FALSE FALSE FALSE FALSE FALSE FALSE FALSE FALSE FALSE TRUE] -> w159
          tunnel: [w170 w200 w275 w345 w443 w517 w610 w672 w769 w839 w933 w999 w1104 w1182 w1271 w1330 w1420 w1479 w1570 w1631 w1702 w1803 w1875 w1882] -> w158
          tunnel: [w169 w177 w274 w342 w433 w514 w600 w669 w759 w836 w923 w996 w1094 w1179 w1261 w1327 w1410 w1476 w1560 w1628 w1699 w1793 w1874 w1884] -> w157
          tunnel: w156 -> [_ w195 w277 w344 w445 w516 w612 w671 w771 w838 w935 w998 w1106 w1181 w1273 w1329 w1422 w1478 w1572 w1630 w1701 w1805 _ _]
          tunnel: w155 -> [_ w201 w276 w346 w444 w518 w611 w673 w770 w840 w934 w1000 w1105 w1183 w1272 w1331 w1421 w1480 w1571 w1632 w1703 w1804 _ _]
          tunnel: w154 -> [w168 w199 w271 w339 w442 w512 w609 w667 w768 w834 w932 w994 w1103 w1177 w1270 w1325 w1419 w1474 w1569 w1626 w1697 w1802 w1872 w1886]
          tunnel: [w168 w199 w271 w339 w442 w512 w609 w667 w768 w834 w932 w994 w1103 w1177 w1270 w1325 w1419 w1474 w1569 w1626 w1697 w1802 w1872 w1886] -> w153
          tunnel: [w167 w194 w267 w340 w438 w511 w605 w666 w764 w833 w928 w993 w1099 w1176 w1266 w1324 w1415 w1473 w1565 w1625 w1696 w1798 w1871 w1877] -> w152
          tunnel: w151 -> [w167 w194 w267 w340 w438 w511 w605 w666 w764 w833 w928 w993 w1099 w1176 w1266 w1324 w1415 w1473 w1565 w1625 w1696 w1798 w1871 w1877]
          tunnel: w150 -> [w166 w188 w256 w338 w432 w510 w599 w665 w758 w832 w922 w992 w1093 w1175 w1260 w1323 w1409 w1472 w1559 w1624 w1695 w1792 w1870 w1876]
          tunnel: [w165 w187 w255 w337 w431 w509 w598 w664 w757 w831 w921 w991 w1092 w1174 w1259 w1322 w1408 w1471 w1558 w1623 w1695 w1791 w1870 w1876] -> w149
          frame "-1", Default {
            n52 = Bundle By Name(cluster=w166, "OP - 10.LEAK RATE"=25357653) -> (w165:T11)
          }
          frame "SCAN1" {
            w180 = u16 0  # CYCLE STATUS OK, NOK, ABORTED
            w179 = refnum<vi> refnum  # Boolean
            # "STATION OP 10"
            n53 = global read "Global 1.vi" "BARCODE RECIPE"() -> (w189:string)
            n54 = call "PADMINI_AUTO_BARCODE_STRING.vi"("Enum"=enum16{"Read", "Write"}."Read", "error in (no error)"=w198) -> ("error out"=w197:errorcluster, "Input 2"=w174:string[])  [unwired: 8 in]
            n55 = Index Array(array=w174) -> (element=w173:string)  [unwired: 1 in]
            n56 = call <vilib>:"Trim Whitespace.vi"("string"=w173) -> ("trimmed string"=w172:string)  [unwired: 1 in]
            n57 = Match Pattern(string=w172, regular expression=w189) -> (match substring=w192:string)  [unwired: 1 in, 3 out]
            n58 = String Length(string=w189) -> (length=w191:i32)
            n59 = String Length(string=w192) -> (length=w190:i32)
            n60 = Equal?(x=w191, y=w190) -> (x = y?=w196:bool)
            n61 = case shown="False" w195 {
              tunnel: w202 -> [w212 w244]
              tunnel: w197 -> [w211 w242]
              tunnel: w201 -> [w210 _]
              tunnel: [w209 w241] -> w176
              tunnel: [w208 w244] -> w200
              tunnel: w196 -> [w207 _]
              tunnel: w172 -> [w206 _]
              frame False {
                n62 = case shown="True" w207 {
                  tunnel: w212 -> [w214 w231]
                  tunnel: w211 -> [w216 w230]
                  tunnel: w210 -> [_ w229]
                  tunnel: [w215 w220] -> w209
                  tunnel: [w214 w219] -> w208
                  tunnel: w206 -> [_ w218]
                  frame False {
                    # "OP10 CURRENT STATION NG"
                    n63 = call "PADMINI_AUTO_BARCODE_STATUS.vi"("Enum"=enum16{"Read", "Write"}."Write", "error in (no error)"=w216, "I/P"=bool[] [FALSE, TRUE]) -> ("error out"=w215:errorcluster)  [unwired: 7 in, 1 out]
                  }
                  frame True {
                    # "OP10 CURRENT STATION OK"
                    n64 = Format Into String(format string="where BARCODE='%s'", w218) -> (resulting string=w226:string)  [unwired: 2 in, 1 out]
                    n65 = call <vilib>:"DB Tools Select Data.vi"("condition"=w226, "error in (no error)"=w230, "columns"=string[] ["BARCODE"], "table"=w229, "connection reference"=w231) -> ("error out"=w225:errorcluster, "data"=w224:variant[][], "connection reference out"=w219:T13)  [unwired: 1 in]
                    n66 = call "PADMINI_varient_to_data.vi"("error in (no error)"=w225, "data"=w224) -> ("error out"=w221:errorcluster, "Array"=w223:string[][])  [unwired: 8 in]
                    n67 = Empty Array?(array=w223) -> (empty?=w222:bool)
                    n68 = case shown="False" w222 {
                      tunnel: w221 -> [w235 w239]
                      tunnel: [w234 w237] -> w220
                      frame False {
                        # "OP10 CURRENT STATION NG\nPART REPEAT"
                        n69 = call "PADMINI_AUTO_BARCODE_STATUS.vi"("Enum"=enum16{"Read", "Write"}."Write", "error in (no error)"=w235, "I/P"=bool[] [FALSE, TRUE]) -> ("error out"=w234:errorcluster)  [unwired: 7 in, 1 out]
                      }
                      frame True {
                        # "OP10 CURRENT STATION OK"
                        n70 = call "PADMINI_AUTO_BARCODE_STATUS.vi"("Enum"=enum16{"Read", "Write"}."Write", "error in (no error)"=w239, "I/P"=bool[] [TRUE, FALSE]) -> ("error out"=w237:errorcluster)  [unwired: 7 in, 1 out]
                      }
                    }
                  }
                }
              }
              frame True {
                n71 = call "PADMINI_AUTO_BARCODE_STATUS.vi"("Enum"=enum16{"Read", "Write"}."Write", "error in (no error)"=w242, "I/P"=bool[] [FALSE, FALSE]) -> ("error out"=w241:errorcluster)  [unwired: 7 in, 1 out]
              }
            }
            n72 = flat-sequence {
              tunnel: [w205] -> w175
              tunnel: w176 -> [w205]
              frame #0 {
                # "UPDATE op 10 sCAN sTATUS"
                n73 = global write "DATA LOG.vi" "OP 10 Outputs"(TRUE) -> ()
              }
            }
            n74 = Bundle By Name(cluster=w188, "OP - 10.BARCODE"=w172) -> (w187:T11)
            n75 = call <vilib>:"Clear Errors.vi"("error in (no error)"=w175) -> ("error out"=w181:errorcluster)  [unwired: 5 in, 1 out]
            n76 = property on="OP - 10" class="Clust"(error in=w181) -> (error out=w185:errorcluster, "Controls[]"=w183:refnum<vi>[])  [unwired: 1 in, 1 out]
            n77 = Index Array(array=w183, index=2) -> (element=w184:refnum<vi>)
            n78 = To More Specific Class(target class=w179, reference=w184, error in=w185) -> (specific class reference=w182:refnum<vi>, error out=w186:errorcluster)
            n79 = call "PADMINI_BOOL_COLOR_CHANGE.vi"("error in (no error)"=w186, "Numeric"=w180, "Boolean in"=w182) -> ("error out"=w177:errorcluster)  [unwired: 8 in]
          }
          frame "DATALOG1" {
            w257 = u16 0  # CYCLE STATUS OK, NOK, ABORTED
            w261 = refnum<vi> refnum  # Boolean
            w269 = T14 2 items=["no dialog", "OK message", "continue or stop message", "OK message + warnings", "continue/stop + warnings"] ("type of dialog (OK msg:1)")
            # "NOT IMPLIMENTED BY PLC"
            # "cycle result status\nwhether it was ok or nok\nor abortted in between"
            # "Printed QR Code data string"
            # "datalog of OP 10"
            n80 = call "PADMINI_AUTO_BARCODE_STRING.vi"("Enum"=enum16{"Read", "Write"}."Read", "error in (no error)"=w245) -> ("Input 2"=w252:string[])  [unwired: 8 in, 1 out]
            n81 = call "PADMINI_AUTO_CYCLE VALUE 10.vi"("Enum"=enum16{"Read", "Write"}."Read", "error in (no error)"=w245) -> ("error out"=w248:errorcluster, "Input 2"=w247:dbl[])  [unwired: 8 in]
            n82 = Index Array(array=w247) -> (element=w246:dbl)  [unwired: 1 in]
            n83 = Index Array(array=w252) -> (element #1=w251:string, element #2=w250:string)  [unwired: 2 in]
            n84 = Number To Fractional String(number=w246, precision (6)=i16 2) -> (F-format string=w253:string)  [unwired: 2 in]
            n85 = call <vilib>:"Trim Whitespace.vi"("string"=w251) -> ("trimmed string"=w272:string)  [unwired: 1 in]
            n86 = case shown="False" w277 {
              tunnel: w278 -> [w300 w335]
              tunnel: w248 -> [w302 w334]
              tunnel: [w308 w333] -> w275
              tunnel: [w307 w332] -> w270
              tunnel: w276 -> [w297 _]
              tunnel: w272 -> [w294 _]
              tunnel: w250 -> [w304 w325]
              tunnel: w253 -> [w288 w324]
              frame False {
                w296 = string[] ["BARCODE", "SHIFT", "DATE", "ST1_LEAK_RATE", "ST1_FINAL_RST"]
                # "ST1 RESULT"
                # "DO TRACEBILITY"
                n87 = local read "SHIFT"() -> (w306:string)
                n88 = Format Into String(format string="Where BARCODE='%s' ", w294) -> (resulting string=w289:string)  [unwired: 2 in, 1 out]
                n89 = call <vilib>:"DB Tools Select Data.vi"("condition"=w289, "error in (no error)"=w302, "columns"=w296, "table"=w297, "connection reference"=w300) -> ("error out"=w298:errorcluster, "data"=w301:variant[][], "connection reference out"=w299:T13)  [unwired: 1 in]
                n90 = call "PADMINI_SHIFT_DATE.vi"("SHIFT"=w306) -> ("date/time string"=w305:string)  [unwired: 10 in]
                n91 = Variant To Data(error in=w298, type=string[][] [], Variant=w301) -> (data=w292:string[][], error out=w290:errorcluster)
                n92 = Bundle("trimmed string"=w294, "SHIFT"=w306, "date/time string"=w305, w288, "Input 2"=w304) -> (w303:T15)  [unwired: 1 in]
                n93 = Empty Array?(array=w292) -> (empty?=w291:bool)
                n94 = case shown="True" w291 {
                  tunnel: w299 -> [w313 w323]
                  tunnel: w290 -> [w312 w322]
                  tunnel: [w316 w321] -> w308
                  tunnel: [w315 w320] -> w307
                  tunnel: w296 -> [w310 w319]
                  tunnel: w297 -> [w311 w318]
                  tunnel: w303 -> [w314 w317]
                  tunnel: w289 -> [w309 _]
                  frame False {
                    n95 = call <vilib>:"DB Tools Update Data.vi"("condition"=w309, "data"=w314, "error in (no error)"=w312, "columns"=w310, "table"=w311, "connection reference"=w313) -> ("error out"=w315:errorcluster, "connection reference out"=w316:T13)  [unwired: 4 in]
                  }
                  frame True {
                    n96 = call <vilib>:"DB Tools Insert Data.vi"("data"=w317, "error in (no error)"=w322, "columns"=w319, "table"=w318, "connection reference"=w323) -> ("error out"=w320:errorcluster, "connection reference out"=w321:T13)  [unwired: 5 in]
                  }
                }
              }
              frame True {
                # "Trac BYPASS"
                n97 = local read "SHIFT"() -> (w330:string)
                n98 = call "PADMINI_SHIFT_DATE.vi"("SHIFT"=w330) -> ("date/time string"=w329:string)  [unwired: 10 in]
                n99 = Bundle("SHIFT"=w330, "date/time string"=w329, "Input 2"=w325, w324) -> (w328:T16)  [unwired: 1 in]
                n100 = To Variant(anything=w328) -> (Variant=w327:variant)
                n101 = call <vilib>:"DB Tools Insert Data.vi"("data"=w327, "error in (no error)"=w334, "columns"=string[] ["DATE", "SHIFT", "ST1_LEAK_RAT", "ST1_FINAL_RST"], "table"="ST1_REPORT", "connection reference"=w335) -> ("error out"=w332:errorcluster, "connection reference out"=w333:T13)  [unwired: 5 in]
              }
            }
            n102 = Bundle By Name(cluster=w256, "OP - 10.LEAK RATE"=w246) -> (w255:T11)
            n103 = call <vilib>:"Simple Error Handler.vi"("type of dialog (OK msg:1)"=w269, "error in (no error)"=w270) -> ("error out"=w268:errorcluster)  [unwired: 3 in, 4 out]
            n104 = call <vilib>:"Clear Errors.vi"("error in (no error)"=w268) -> ("error out"=w266:errorcluster)  [unwired: 5 in, 1 out]
            n105 = property on="OP - 10" class="Clust"(error in=w266) -> (error out=w260:errorcluster, "Controls[]"=w264:refnum<vi>[])  [unwired: 1 in, 1 out]
            n106 = Index Array(array=w264, index=2) -> (element=w262:refnum<vi>)
            n107 = To More Specific Class(target class=w261, reference=w262, error in=w260) -> (specific class reference=w265:refnum<vi>, error out=w259:errorcluster)
            n108 = call "PADMINI_BOOL_COLOR_CHANGE.vi"("error in (no error)"=w259, "Numeric"=w257, "Boolean in"=w265) -> ("error out"=w258:errorcluster)  [unwired: 8 in]
            n109 = disable-structure shown="Disabled" {
              disable-tunnel: [w281 w287] -> w274
              disable-tunnel: w258 -> [w280 w287]
              frame Disabled {
                n110 = call "PADMINI_AUTO_DATALOG_DONE.vi"("Enum"=enum16{"Read", "Write"}."Write", "error in (no error)"=w280, "I/P"=u16 2) -> ("error out"=w282:errorcluster)  [unwired: 7 in, 1 out]
                n111 = flat-sequence {
                  tunnel: [w285] -> w281
                  tunnel: w282 -> [w285]
                  frame #0 {
                    n112 = global write "DATA LOG.vi" "OP 10 DATA LOG RESULT"(TRUE ("DATA LOG RESET")) -> ()
                  }
                }
              }
              frame Enabled {
              }
            }
          }
          frame "SCAN2" {
            # "Barcode Status\n0-Ideal, 1-Ok, 2-Nok, 3-Prev Station Not Done,\n4-Prev Station Nok,\n5- Already Done"
            # "STATION OP 20"
            n113 = case shown="True" w344 {
              tunnel: w348 -> [w372 w407]
              tunnel: w347 -> [w364 w405]
              tunnel: w346 -> [_ _]
              tunnel: [w367 w404] -> w343
              tunnel: [w365 w407] -> w345
              tunnel: [w349 "" ("trimmed string")] -> w336
              frame False {
                # "2 FOR EMPTY BARCODE READ OR MISMATCH"
                n114 = call "PADMINI_AUTO_BARCODE_STRING2.vi"("Enum"=enum16{"Read", "Write"}."Read", "error in (no error)"=w364) -> ("error out"=w363:errorcluster, "Input 2"=w351:string[])  [unwired: 8 in]
                n115 = global read "Global 1.vi" "BARCODE RECIPE"() -> (w352:string)
                n116 = Index Array(array=w351) -> (element=w350:string)  [unwired: 1 in]
                n117 = call <vilib>:"Trim Whitespace.vi"("string"=w350) -> ("trimmed string"=w349:string)  [unwired: 1 in]
                n118 = Match Pattern(string=w349, regular expression=w352) -> (match substring=w353:string)  [unwired: 1 in, 3 out]
                n119 = String Length(string=w352) -> (length=w355:i32)
                n120 = String Length(string=w353) -> (length=w354:i32)
                n121 = Format Into String(format string="WHERE BARCODE  ='%s'", w349) -> (resulting string=w359:string)  [unwired: 2 in, 1 out]
                n122 = Equal?(x=w355, y=w354) -> (x = y?=w356:bool)
                n123 = call <vilib>:"DB Tools Select Data.vi"("condition"=w359, "error in (no error)"=w363, "columns"=string[] ["BARCODE", "ST1_FINAL_RST", "ST2_FINAL_RST"], "table"="REPORT", "connection reference"=w372) -> ("error out"=w370:errorcluster, "data"=w369:variant[][], "connection reference out"=w365:T13)  [unwired: 1 in]
                n124 = call "PADMINI_varient_to_data.vi"("error in (no error)"=w370, "data"=w369) -> ("error out"=w368:errorcluster, "Array"=w366:string[][])  [unwired: 8 in]
                n125 = Equal?(x=w349, y="") -> (x = y?=w357:bool)
                n126 = case shown="False" w357 {
                  selector: w357 -> [_ w401]
                  tunnel: w368 -> [w376 w400]
                  tunnel: [w375 w399] -> w367
                  tunnel: w366 -> [w374 _]
                  tunnel: w356 -> [w373 _]
                  frame False {
                    n127 = case shown="True" w373 {
                      tunnel: w376 -> [w379 w389]
                      tunnel: [w378 w396] -> w375
                      tunnel: w374 -> [_ w395]
                      frame False {
                        n128 = call "PADMINI_AUTO_BARCODE_STATUS 20.vi"("Enum"=enum16{"Read", "Write"}."Write", "error in (no error)"=w379, "I/P"=bool[] [FALSE, TRUE, FALSE, FALSE, FALSE, FALSE]) -> ("error out"=w378:errorcluster)  [unwired: 7 in, 1 out]
                      }
                      frame True {
                        # "ST2 RESULT"
                        # "ST1 RESULT"
                        n129 = Index Array(array=w395, index (row) #1=0 ("index (row)"), index (col) #1=1 ("disabled index (col)"), index (row) #2=0 ("index (row)"), index (col) #2=2 ("disabled index (col)")) -> (element #1=w388:string)  [unwired: 1 out]
                        n130 = Empty String/Path?(string/path=w388) -> (empty?=w386:bool)
                        n131 = Equal?(x=w388, y="OK") -> (x = y?=w382:bool)
                        n132 = Not(x=w382) -> (.not. x?=w381:bool)
                        n133 = Build Array(TRUE ("element"), FALSE ("element"), w386, w382, w381) -> (w385:bool[])
                        n134 = call "PADMINI_AUTO_BARCODE_STATUS 20.vi"("Enum"=enum16{"Read", "Write"}."Write", "error in (no error)"=w389, "I/P"=w385) -> ("error out"=w396:errorcluster)  [unwired: 7 in, 1 out]
                      }
                    }
                  }
                  frame True {
                    n135 = call "PADMINI_AUTO_BARCODE_STATUS 20.vi"("Enum"=enum16{"Read", "Write"}."Write", "error in (no error)"=w400, "I/P"=bool[] [FALSE, FALSE, FALSE, FALSE, FALSE]) -> ("error out"=w399:errorcluster)  [unwired: 7 in, 1 out]
                    "OP30 BARCODE STRING EMPRTY" <- w401
                  }
                }
              }
              frame True {
                n136 = call "PADMINI_AUTO_BARCODE_STATUS 20.vi"("Enum"=enum16{"Read", "Write"}."Write", "error in (no error)"=w405, "I/P"=bool[] [FALSE, FALSE, FALSE, FALSE, FALSE]) -> ("error out"=w404:errorcluster)  [unwired: 7 in, 1 out]
              }
            }
            n137 = flat-sequence {
              tunnel: [w409] -> w342
              tunnel: w343 -> [w409]
              frame #0 {
                # "UPDATE op 20 SCAN sTATUS"
                n138 = global write "DATA LOG.vi" "OP 20 Outputs"(TRUE) -> ()
              }
            }
            n139 = Bundle By Name(cluster=w338, "OP - 20.BARCODE"=w336) -> (w337:T11)
          }
          frame "DATALOG2" {
            w440 = T14 2 items=["no dialog", "OK message", "continue or stop message", "OK message + warnings", "continue/stop + warnings"] ("type of dialog (OK msg:1)")
            # "Printed QR Code data string"
            # "datalog of OP 20"
            n140 = call "PADMINI_AUTO_BARCODE_STRING2.vi"("Enum"=enum16{"Read", "Write"}."Read", "error in (no error)"=w427) -> ("error out"=w429:errorcluster, "Input 2"=w411:string[])  [unwired: 8 in]
            n141 = call "PADMINI_AUTO_CYCLE VALUE 20.vi"("Enum"=enum16{"Read", "Write"}."Read", "error in (no error)"=w427) -> ("Input 2"=w421:dbl[])  [unwired: 8 in, 1 out]
            n142 = Index Array(array=w421) -> (element #1=w426:dbl, element #2=w425:dbl, element #3=w424:dbl, element #4=w423:dbl)  [unwired: 4 in]
            n143 = Number To Fractional String(number=w421, precision (6)=i16 2) -> (F-format string=w420:string[])  [unwired: 2 in]
            n144 = case shown="True" w445 {
              tunnel: w446 -> [w481 w507]
              tunnel: w429 -> [w482 w506]
              tunnel: [w485 w505] -> w443
              tunnel: [w484 w504] -> w441
              tunnel: w444 -> [w480 _]
              tunnel: w420 -> [w476 w489]
              tunnel: w411 -> [w468 w490]
              frame False {
                # "ST2 RESULT"
                # "DO TRACEBILITY"
                n145 = Index Array(array=w468) -> (element #1=w469:string, element #2=w467:string, element #3=w466:string, element #4=w465:string, element #5=w464:string, element #6=w463:string, element #7=w462:string)  [unwired: 7 in]
                n146 = local read "SHIFT"() -> (w483:string)
                n147 = Index Array(array=w476) -> (element #1=w475:string, element #2=w474:string, element #3=w473:string, element #4=w472:string)  [unwired: 4 in]
                n148 = call <vilib>:"Trim Whitespace.vi"("string"=w469) -> ("trimmed string"=w470:string)  [unwired: 1 in]
                n149 = call "PADMINI_SHIFT_DATE.vi"("SHIFT"=w483) -> ()  [unwired: 10 in, 1 out]
                n150 = Format Into String(format string="Where BARCODE='%s' ", w470) -> (resulting string=w478:string)  [unwired: 2 in, 1 out]
                n151 = Bundle("Input 2"=w475, "Input 2"=w474, "Input 2"=w467, "Input 2"=w466, "Input 2"=w473, "Input 2"=w472, "Input 2"=w465, "Input 2"=w464, "Input 2"=w463, "Input 2"=w462) -> (w471:T17)  [unwired: 1 in]
                n152 = call <vilib>:"DB Tools Update Data.vi"("condition"=w478, "data"=w471, "error in (no error)"=w482, "columns"=string[] ["ST2_LOWER_BEARING_DIS", "ST2_LOWER_BEARING_LOAD", "ST2_BOTTOM_CAMERA_STATUS", "ST2_LOWER_BEARING_RST", "ST2_UPPER_BEARING_DIS", "ST2_UPPER_BEARING_LOAD", "ST2_UPPER_SIM_STATUS", "ST2_UPPER_CAMERA_STATUS", "ST2_UPPER_BERAING_RST", "ST2_FINAL_RST"], "table"=w480, "connection reference"=w481) -> ("error out"=w484:errorcluster, "connection reference out"=w485:T13)  [unwired: 4 in]
              }
              frame True {
                n153 = local read "SHIFT"() -> (w487:string)
                n154 = Index Array(array=w490) -> (element #2=w496:string, element #3=w495:string, element #4=w494:string, element #5=w493:string, element #6=w492:string, element #7=w486:string)  [unwired: 7 in, 1 out]
                n155 = call "PADMINI_SHIFT_DATE.vi"("SHIFT"=w487) -> ("date/time string"=w488:string)  [unwired: 10 in]
                n156 = Index Array(array=w489) -> (element #1=w500:string, element #2=w499:string, element #3=w498:string, element #4=w497:string)  [unwired: 4 in]
                n157 = Bundle("date/time string"=w488, "SHIFT"=w487, "Input 2"=w500, "Input 2"=w499, "Input 2"=w496, "Input 2"=w495, "Input 2"=w498, "Input 2"=w497, "Input 2"=w494, "Input 2"=w493, "Input 2"=w492, "Input 2"=w486) -> (w491:T18)  [unwired: 1 in]
                n158 = To Variant(anything=w491) -> (Variant=w502:variant)
                n159 = call <vilib>:"DB Tools Insert Data.vi"("data"=w502, "error in (no error)"=w506, "columns"=string[] ["DATE", "SHIFT", "ST2_LOWER_BEARING_DIS", "ST2_LOWER_BEARING_LOAD", "ST2_BOTTOM_CAMERA_STATUS", "ST2_LOWER_BEARING_RST", "ST2_UPPER_BEARING_DIS", "ST2_UPPER_BEARING_LOAD", "ST2_UPPER_SIM_STATUS", "ST2_UPPER_CAMERA_STATUS", "ST2_UPPER_BERAING_RST", "ST2_FINAL_RST"], "table"="ST2_REPORT", "connection reference"=w507) -> ("error out"=w504:errorcluster, "connection reference out"=w505:T13)  [unwired: 5 in]
              }
            }
            n160 = Bundle By Name(cluster=w432, "OP - 20.LOWERING BEARING DISPLACE"=w426, "OP - 20.LOWERING BEARING LOAD"=w425, "OP - 20.UPPER BEARING DISPLACE"=w424, "OP - 20.UPPER BEARING LOAD"=w423) -> (w431:T11)
            n161 = call <vilib>:"Simple Error Handler.vi"("type of dialog (OK msg:1)"=w440, "error in (no error)"=w441) -> ("error out"=w439:errorcluster)  [unwired: 3 in, 4 out]
            n162 = call <vilib>:"Clear Errors.vi"("error in (no error)"=w439) -> ("error out"=w437:errorcluster)  [unwired: 5 in, 1 out]
            n163 = property on="OP - 20" class="Clust"(error in=w437) -> (error out=w434:errorcluster, "Controls[]"=w436:refnum<vi>[])  [unwired: 1 in, 1 out]
            n164 = for {
              tunnel: w411 -> [w451] mode=indexing
              tunnel: [w450] -> w410 mode=indexing if=w448
              i -> [w449]
              n165 = case shown="\"NG\"" w451 {
                tunnel: [2 ("CYCLE STATUS OK, NOK, ABORTED") 1 ("CYCLE STATUS OK, NOK, ABORTED") 0 ("CYCLE STATUS OK, NOK, ABORTED")] -> w450
                frame "NG" {
                }
                frame "OK" {
                }
                frame "-1", Default {
                }
              }
              n166 = Not Equal To 0?(x=w449) -> (x != 0?=w448:bool)
            }
            n167 = Index Array(array=w436, index #1=3 ("index"), index #3=7 ("index")) -> (element #1=w418:refnum<vi>, element #2=w417:refnum<vi>, element #3=w416:refnum<vi>, element #4=w415:refnum<vi>, element #5=w414:refnum<vi>, element #6=w413:refnum<vi>)  [unwired: 4 in]
            n168 = Build Array(w418, w417, w416, w415, w414, w413) -> (w412:refnum<vi>[])
            n169 = for {
              tunnel: w412 -> [w460] mode=indexing
              shift-right: [w456] -> w433
              shift-left: w434 -> [w458]
              tunnel: w410 -> [w455] mode=indexing
              w459 = refnum<vi> refnum  # Boolean
              n170 = To More Specific Class(target class=w459, reference=w460, error in=w458) -> (specific class reference=w461:refnum<vi>, error out=w457:errorcluster)
              n171 = call "PADMINI_BOOL_COLOR_CHANGE.vi"("error in (no error)"=w457, "Numeric"=w455, "Boolean in"=w461) -> ("error out"=w456:errorcluster)  [unwired: 8 in]
            }
          }
          frame "SCAN3" {
            # "STATION OP 30"
            n172 = case shown="False" w516 {
              tunnel: w520 -> [w544 w579]
              tunnel: w519 -> [w536 w577]
              tunnel: w518 -> [_ _]
              tunnel: [w539 w576] -> w515
              tunnel: [w537 w579] -> w517
              tunnel: [w521 "" ("trimmed string")] -> w508
              frame False {
                n173 = call "PADMINI_AUTO_BARCODE_STRING 30.vi"("Enum"=enum16{"Read", "Write"}."Read", "error in (no error)"=w536) -> ("error out"=w535:errorcluster, "Input 2"=w523:string[])  [unwired: 8 in]
                n174 = global read "Global 1.vi" "BARCODE RECIPE"() -> (w524:string)
                n175 = Index Array(array=w523) -> (element=w522:string)  [unwired: 1 in]
                n176 = call <vilib>:"Trim Whitespace.vi"("string"=w522) -> ("trimmed string"=w521:string)  [unwired: 1 in]
                n177 = Match Pattern(string=w521, regular expression=w524) -> (match substring=w525:string)  [unwired: 1 in, 3 out]
                n178 = String Length(string=w524) -> (length=w527:i32)
                n179 = String Length(string=w525) -> (length=w526:i32)
                n180 = Format Into String(format string="WHERE BARCODE  ='%s'", w521) -> (resulting string=w531:string)  [unwired: 2 in, 1 out]
                n181 = Equal?(x=w527, y=w526) -> (x = y?=w528:bool)
                n182 = call <vilib>:"DB Tools Select Data.vi"("condition"=w531, "error in (no error)"=w535, "columns"=string[] ["BARCODE", "ST2_FINAL_RST", "ST3_FINAL_RST"], "table"="REPORT", "connection reference"=w544) -> ("error out"=w542:errorcluster, "data"=w541:variant[][], "connection reference out"=w537:T13)  [unwired: 1 in]
                n183 = call "PADMINI_varient_to_data.vi"("error in (no error)"=w542, "data"=w541) -> ("error out"=w540:errorcluster, "Array"=w538:string[][])  [unwired: 8 in]
                n184 = Equal?(x=w521, y="") -> (x = y?=w529:bool)
                n185 = case shown="False" w529 {
                  selector: w529 -> [_ w573]
                  tunnel: w540 -> [w548 w572]
                  tunnel: [w547 w571] -> w539
                  tunnel: w538 -> [w546 _]
                  tunnel: w528 -> [w545 _]
                  frame False {
                    n186 = case shown="True" w545 {
                      tunnel: w548 -> [w551 w561]
                      tunnel: [w550 w568] -> w547
                      tunnel: w546 -> [_ w567]
                      frame False {
                        n187 = call "PADMINI_AUTO_BARCODE_STATUS 30.vi"("Enum"=enum16{"Read", "Write"}."Write", "error in (no error)"=w551, "I/P"=bool[] [FALSE, TRUE, FALSE, FALSE, FALSE, FALSE]) -> ("error out"=w550:errorcluster)  [unwired: 7 in, 1 out]
                      }
                      frame True {
                        n188 = Index Array(array=w567, index (row) #1=0 ("index (row)"), index (col) #1=1 ("disabled index (col)"), index (row) #2=0 ("index (row)"), index (col) #2=2 ("disabled index (col)")) -> (element #1=w560:string)  [unwired: 1 out]
                        n189 = Empty String/Path?(string/path=w560) -> (empty?=w558:bool)
                        n190 = Equal?(x=w560, y="OK") -> (x = y?=w554:bool)
                        n191 = Not(x=w554) -> (.not. x?=w553:bool)
                        n192 = Build Array(TRUE ("element"), FALSE ("element"), w558, w554, w553) -> (w557:bool[])
                        n193 = call "PADMINI_AUTO_BARCODE_STATUS 30.vi"("Enum"=enum16{"Read", "Write"}."Write", "error in (no error)"=w561, "I/P"=w557) -> ("error out"=w568:errorcluster)  [unwired: 7 in, 1 out]
                      }
                    }
                  }
                  frame True {
                    n194 = call "PADMINI_AUTO_BARCODE_STATUS 30.vi"("Enum"=enum16{"Read", "Write"}."Write", "error in (no error)"=w572, "I/P"=bool[] [FALSE, FALSE, FALSE, FALSE, FALSE]) -> ("error out"=w571:errorcluster)  [unwired: 7 in, 1 out]
                    "OP30 BARCODE STRING EMPRTY 2" <- w573
                  }
                }
              }
              frame True {
                n195 = call "PADMINI_AUTO_BARCODE_STATUS 30.vi"("Enum"=enum16{"Read", "Write"}."Write", "error in (no error)"=w577, "I/P"=bool[] [FALSE, FALSE, FALSE, FALSE, FALSE]) -> ("error out"=w576:errorcluster)  [unwired: 7 in, 1 out]
              }
            }
            n196 = flat-sequence {
              tunnel: [w582] -> w514
              tunnel: w515 -> [w582]
              frame #0 {
                # "UPDATE op 30 SCAN sTATUS"
                n197 = local write "OP30 BARCODE STRING EMPRTY 2"(FALSE ("Boolean 5")) -> ()
                n198 = global write "DATA LOG.vi" "OP 30 Outputs"(TRUE) -> ()
              }
            }
            n199 = Bundle By Name(cluster=w510, "OP - 30.BARCODE"=w508) -> (w509:T11)
          }
          frame "DATALOG3" {
            w607 = T14 2 items=["no dialog", "OK message", "continue or stop message", "OK message + warnings", "continue/stop + warnings"] ("type of dialog (OK msg:1)")
            # "Printed QR Code data string"
            # "datalog of OP 30"
            n200 = call "PADMINI_AUTO_BARCODE_STRING 30.vi"("Enum"=enum16{"Read", "Write"}."Read", "error in (no error)"=w594) -> ("error out"=w596:errorcluster, "Input 2"=w585:string[])  [unwired: 8 in]
            n201 = call "PADMINI_AUTO_CYCLE VALUE 30.vi"("Enum"=enum16{"Read", "Write"}."Read", "error in (no error)"=w594) -> ("Input 2"=w590:dbl[])  [unwired: 8 in, 1 out]
            n202 = Index Array(array=w590) -> (element #1=w593:dbl, element #2=w592:dbl)  [unwired: 2 in]
            n203 = Number To Fractional String(number=w590, precision (6)=i16 2) -> (F-format string=w589:string[])  [unwired: 2 in]
            n204 = case shown="True" w612 {
              tunnel: w613 -> [w642 w662]
              tunnel: w596 -> [w643 w661]
              tunnel: [w646 w660] -> w610
              tunnel: [w645 w659] -> w608
              tunnel: w611 -> [w641 _]
              tunnel: w589 -> [w637 w647]
              tunnel: w585 -> [w631 w648]
              frame False {
                # "DO TRACEBILITY"
                n205 = Index Array(array=w631) -> (element #1=w632:string, element #2=w630:string, element #3=w629:string)  [unwired: 3 in]
                n206 = local read "SHIFT"() -> (w644:string)
                n207 = Index Array(array=w637) -> (element #1=w636:string, element #2=w635:string)  [unwired: 2 in]
                n208 = call <vilib>:"Trim Whitespace.vi"("string"=w632) -> ("trimmed string"=w633:string)  [unwired: 1 in]
                n209 = call "PADMINI_SHIFT_DATE.vi"("SHIFT"=w644) -> ()  [unwired: 10 in, 1 out]
                n210 = Format Into String(format string="Where BARCODE='%s' ", w633) -> (resulting string=w639:string)  [unwired: 2 in, 1 out]
                n211 = Bundle("Input 2"=w636, "Input 2"=w635, "Input 2"=w630, "Input 2"=w629) -> (w634:T19)  [unwired: 1 in]
                n212 = call <vilib>:"DB Tools Update Data.vi"("condition"=w639, "data"=w634, "error in (no error)"=w643, "columns"=string[] ["ST3_DISPLACEMENT", "ST3_LOAD", "ST3_MIDDLE_GEAR_SHAFT_STATUS", "ST3_FINAL_RST"], "table"=w641, "connection reference"=w642) -> ("error out"=w645:errorcluster, "connection reference out"=w646:T13)  [unwired: 4 in]
              }
              frame True {
                # "TRAC BYPASS"
                n213 = local read "SHIFT"() -> (w649:string)
                n214 = call "PADMINI_SHIFT_DATE.vi"("SHIFT"=w649) -> ("date/time string"=w650:string)  [unwired: 10 in]
                n215 = Index Array(array=w648) -> (element #2=w654:string, element #3=w653:string)  [unwired: 3 in, 1 out]
                n216 = Index Array(array=w647) -> (element #1=w656:string, element #2=w655:string)  [unwired: 2 in]
                n217 = Bundle("date/time string"=w650, "SHIFT"=w649, "Input 2"=w656, "Input 2"=w655, "Input 2"=w654, "Input 2"=w653) -> (w651:T20)  [unwired: 1 in]
                n218 = To Variant(anything=w651) -> (Variant=w652:variant)
                n219 = call <vilib>:"DB Tools Insert Data.vi"("data"=w652, "error in (no error)"=w661, "columns"=string[] ["DATE", "SHIFT", "ST3_DISPLACEMENT", "ST3_LOAD", "ST3_MIDDLE_GEAR_SHAFT_STATUS", "ST3_FINAL_RST"], "table"="ST3_REPORT", "connection reference"=w662) -> ("error out"=w659:errorcluster, "connection reference out"=w660:T13)  [unwired: 5 in]
              }
            }
            n220 = Bundle By Name(cluster=w599, "OP - 30.Displacement"=w593, "OP - 30.Load"=w592) -> (w598:T11)
            n221 = call <vilib>:"Simple Error Handler.vi"("type of dialog (OK msg:1)"=w607, "error in (no error)"=w608) -> ("error out"=w606:errorcluster)  [unwired: 3 in, 4 out]
            n222 = call <vilib>:"Clear Errors.vi"("error in (no error)"=w606) -> ("error out"=w604:errorcluster)  [unwired: 5 in, 1 out]
            n223 = property on="OP - 30" class="Clust"(error in=w604) -> (error out=w601:errorcluster, "Controls[]"=w603:refnum<vi>[])  [unwired: 1 in, 1 out]
            n224 = for {
              tunnel: w585 -> [w618] mode=indexing
              tunnel: [w617] -> w584 mode=indexing if=w615
              i -> [w616]
              n225 = case shown="\"NG\"" w618 {
                tunnel: [2 ("CYCLE STATUS OK, NOK, ABORTED") 1 ("CYCLE STATUS OK, NOK, ABORTED") 0 ("CYCLE STATUS OK, NOK, ABORTED")] -> w617
                frame "NG" {
                }
                frame "OK" {
                }
                frame "-1", Default {
                }
              }
              n226 = Not Equal To 0?(x=w616) -> (x != 0?=w615:bool)
            }
            n227 = Index Array(array=w603, index #1=3 ("index"), index #2=4 ("index")) -> (element #1=w588:refnum<vi>, element #2=w587:refnum<vi>)
            n228 = Build Array(w588, w587) -> (w586:refnum<vi>[])
            n229 = for {
              tunnel: w586 -> [w627] mode=indexing
              shift-right: [w623] -> w600
              shift-left: w601 -> [w625]
              tunnel: w584 -> [w622] mode=indexing
              w626 = refnum<vi> refnum  # Boolean
              n230 = To More Specific Class(target class=w626, reference=w627, error in=w625) -> (specific class reference=w628:refnum<vi>, error out=w624:errorcluster)
              n231 = call "PADMINI_BOOL_COLOR_CHANGE.vi"("error in (no error)"=w624, "Numeric"=w622, "Boolean in"=w628) -> ("error out"=w623:errorcluster)  [unwired: 8 in]
            }
          }
          frame "SCAN4" {
            # "STATION OP 40"
            n232 = case shown="True" w671 {
              tunnel: w675 -> [w699 w733]
              tunnel: w674 -> [w691 w732]
              tunnel: w673 -> [_ _]
              tunnel: [w694 w731] -> w670
              tunnel: [w692 w733] -> w672
              tunnel: [w676 "" ("trimmed string")] -> w663
              frame False {
                n233 = call "PADMINI_AUTO_BARCODE_STRING 40.vi"("Enum"=enum16{"Read", "Write"}."Read", "error in (no error)"=w691) -> ("error out"=w690:errorcluster, "Input 2"=w678:string[])  [unwired: 8 in]
                n234 = global read "Global 1.vi" "BARCODE RECIPE"() -> (w679:string)
                n235 = Index Array(array=w678) -> (element=w677:string)  [unwired: 1 in]
                n236 = call <vilib>:"Trim Whitespace.vi"("string"=w677) -> ("trimmed string"=w676:string)  [unwired: 1 in]
                n237 = Match Pattern(string=w676, regular expression=w679) -> (match substring=w680:string)  [unwired: 1 in, 3 out]
                n238 = String Length(string=w679) -> (length=w682:i32)
                n239 = String Length(string=w680) -> (length=w681:i32)
                n240 = Format Into String(format string="WHERE BARCODE  ='%s'", w676) -> (resulting string=w686:string)  [unwired: 2 in, 1 out]
                n241 = Equal?(x=w682, y=w681) -> (x = y?=w683:bool)
                n242 = call <vilib>:"DB Tools Select Data.vi"("condition"=w686, "error in (no error)"=w690, "columns"=string[] ["BARCODE", "ST3_FINAL_RST", "ST4_FINAL_RST"], "table"="REPORT", "connection reference"=w699) -> ("error out"=w697:errorcluster, "data"=w696:variant[][], "connection reference out"=w692:T13)  [unwired: 1 in]
                n243 = call "PADMINI_varient_to_data.vi"("error in (no error)"=w697, "data"=w696) -> ("error out"=w695:errorcluster, "Array"=w693:string[][])  [unwired: 8 in]
                n244 = Equal?(x=w676, y="") -> (x = y?=w684:bool)
                n245 = case shown="True" w684 {
                  tunnel: w695 -> [w703 w727]
                  tunnel: [w702 w726] -> w694
                  tunnel: w693 -> [w701 _]
                  tunnel: w683 -> [w700 _]
                  frame False {
                    n246 = case shown="False" w700 {
                      tunnel: w703 -> [w707 w710]
                      tunnel: [w706 w709] -> w702
                      tunnel: w701 -> [_ w723]
                      frame False {
                        n247 = call "PADMINI_AUTO_BARCODE_STATUS 40.vi"("Enum"=enum16{"Read", "Write"}."Write", "error in (no error)"=w707, "I/P"=bool[] [FALSE, TRUE, FALSE, FALSE, FALSE]) -> ("error out"=w706:errorcluster)  [unwired: 7 in, 1 out]
                      }
                      frame True {
                        n248 = Index Array(array=w723, index (row) #1=0 ("index (row)"), index (col) #1=1 ("disabled index (col)"), index (row) #2=0 ("index (row)"), index (col) #2=2 ("disabled index (col)")) -> (element #1=w717:string)  [unwired: 1 out]
                        n249 = Empty String/Path?(string/path=w717) -> (empty?=w715:bool)
                        n250 = Equal?(x=w717, y="OK") -> (x = y?=w713:bool)
                        n251 = Not(x=w713) -> (.not. x?=w712:bool)
                        n252 = Build Array(TRUE ("element"), FALSE ("element"), w715, w713, w712) -> (w711:bool[])
                        n253 = call "PADMINI_AUTO_BARCODE_STATUS 40.vi"("Enum"=enum16{"Read", "Write"}."Write", "error in (no error)"=w710, "I/P"=w711) -> ("error out"=w709:errorcluster)  [unwired: 7 in, 1 out]
                      }
                    }
                  }
                  frame True {
                    n254 = call "PADMINI_AUTO_BARCODE_STATUS 40.vi"("Enum"=enum16{"Read", "Write"}."Write", "error in (no error)"=w727, "I/P"=bool[] [FALSE, FALSE, FALSE, FALSE, FALSE]) -> ("error out"=w726:errorcluster)  [unwired: 7 in, 1 out]
                  }
                }
              }
              frame True {
                n255 = call "PADMINI_AUTO_BARCODE_STATUS 40.vi"("Enum"=enum16{"Read", "Write"}."Write", "error in (no error)"=w732, "I/P"=bool[] [FALSE, FALSE, FALSE, FALSE, FALSE]) -> ("error out"=w731:errorcluster)  [unwired: 7 in, 1 out]
              }
            }
            n256 = flat-sequence {
              tunnel: [w735] -> w669
              tunnel: w670 -> [w735]
              frame #0 {
                # "UPDATE op 40 SCAN sTATUS"
                n257 = global write "DATA LOG.vi" "OP 40 Outputs"(TRUE) -> ()
              }
            }
            n258 = Bundle By Name(cluster=w665, "OP - 40.BARCODE"=w663) -> (w664:T11)
          }
          frame "DATALOG4" {
            w766 = T14 2 items=["no dialog", "OK message", "continue or stop message", "OK message + warnings", "continue/stop + warnings"] ("type of dialog (OK msg:1)")
            # "datalog of OP 40"
            n259 = call "PADMINI_AUTO_BARCODE_STRING 40.vi"("Enum"=enum16{"Read", "Write"}."Read", "error in (no error)"=w753) -> ("error out"=w755:errorcluster, "Input 2"=w744:string[])  [unwired: 8 in]
            n260 = call "PADMINI_AUTO_CYCLE VALUE 40.vi"("Enum"=enum16{"Read", "Write"}."Read", "error in (no error)"=w753) -> ("Input 2"=w749:dbl[])  [unwired: 8 in, 1 out]
            n261 = Index Array(array=w749) -> (element #1=w752:dbl, element #2=w751:dbl, element #3=w741:dbl, element #4=w740:dbl)  [unwired: 4 in]
            n262 = Number To Fractional String(number=w749, precision (6)=i16 2) -> (F-format string=w748:string[])  [unwired: 2 in]
            n263 = case shown="True" w771 {
              tunnel: w772 -> [w805 w829]
              tunnel: w755 -> [w806 w828]
              tunnel: [w809 w827] -> w769
              tunnel: [w808 w826] -> w767
              tunnel: w770 -> [w804 _]
              tunnel: w748 -> [w800 w811]
              tunnel: w744 -> [w795 w810]
              frame False {
                # "DO TRACEBILITY"
                n264 = Index Array(array=w795) -> (element #1=w796:string, element #2=w791:string, element #3=w790:string, element #4=w789:string, element #5=w788:string)  [unwired: 5 in]
                n265 = local read "SHIFT"() -> (w807:string)
                n266 = Index Array(array=w800) -> (element #1=w799:string, element #2=w794:string, element #3=w793:string, element #4=w792:string)  [unwired: 4 in]
                n267 = call <vilib>:"Trim Whitespace.vi"("string"=w796) -> ("trimmed string"=w797:string)  [unwired: 1 in]
                n268 = call "PADMINI_SHIFT_DATE.vi"("SHIFT"=w807) -> ()  [unwired: 10 in, 1 out]
                n269 = Format Into String(format string="Where BARCODE='%s' ", w797) -> (resulting string=w802:string)  [unwired: 2 in, 1 out]
                n270 = Bundle("Input 2"=w799, "Input 2"=w791, "Input 2"=w794, "Input 2"=w790, "Input 2"=w793, "Input 2"=w792, "Input 2"=w788, "Input 2"=w789) -> (w798:T21)  [unwired: 1 in]
                n271 = call <vilib>:"DB Tools Update Data.vi"("condition"=w802, "data"=w798, "error in (no error)"=w806, "columns"=string[] ["ST4_SCREW1_DATA", "ST4_SCREW1_STATUS", "ST4_SCREW2_DATA", "ST4_SCREW2_STATUS", "ST4_DISPLACEMENT", "ST4_LOAD", "ST4_TOP_BEARING_CAMERA_STAUS", "ST4_FINAL_RST"], "table"=w804, "connection reference"=w805) -> ("error out"=w808:errorcluster, "connection reference out"=w809:T13)  [unwired: 4 in]
              }
              frame True {
                # "TRAC BYPASS"
                n272 = local read "SHIFT"() -> (w812:string)
                n273 = Index Array(array=w810) -> (element #2=w820:string, element #3=w819:string, element #4=w818:string, element #5=w817:string)  [unwired: 5 in, 1 out]
                n274 = call "PADMINI_SHIFT_DATE.vi"("SHIFT"=w812) -> ("date/time string"=w813:string)  [unwired: 10 in]
                n275 = Index Array(array=w811) -> (element #1=w814:string, element #2=w823:string, element #3=w822:string, element #4=w821:string)  [unwired: 4 in]
                n276 = Bundle("date/time string"=w813, "SHIFT"=w812, "Input 2"=w814, "Input 2"=w820, "Input 2"=w823, "Input 2"=w819, "Input 2"=w822, "Input 2"=w821, "Input 2"=w817, "Input 2"=w818) -> (w816:T22)  [unwired: 1 in]
                n277 = To Variant(anything=w816) -> (Variant=w815:variant)
                n278 = call <vilib>:"DB Tools Insert Data.vi"("data"=w815, "error in (no error)"=w828, "columns"=string[] ["DATE", "SHIFT", "ST4_SCREW1_DATA", "ST4_SCREW1_STATUS", "ST4_SCREW2_DATA", "ST4_SCREW2_STATUS", "ST4_DISPLACEMENT", "ST4_LOAD", "ST4_TOP_BEARING_CAMERA_STAUS", "ST4_FINAL_RST"], "table"="ST4_REPORT", "connection reference"=w829) -> ("error out"=w826:errorcluster, "connection reference out"=w827:T13)  [unwired: 5 in]
              }
            }
            n279 = Bundle By Name(cluster=w758, "OP - 40.Screw 1 Data"=w752, "OP - 40.Screw 2 data"=w751, "OP - 40.Dispalcement"=w741, "OP - 40.Load"=w740) -> (w757:T11)
            n280 = call <vilib>:"Simple Error Handler.vi"("type of dialog (OK msg:1)"=w766, "error in (no error)"=w767) -> ("error out"=w765:errorcluster)  [unwired: 3 in, 4 out]
            n281 = call <vilib>:"Clear Errors.vi"("error in (no error)"=w765) -> ("error out"=w763:errorcluster)  [unwired: 5 in, 1 out]
            n282 = property on="OP - 40" class="Clust"(error in=w763) -> (error out=w760:errorcluster, "Controls[]"=w762:refnum<vi>[])  [unwired: 1 in, 1 out]
            n283 = for {
              tunnel: w744 -> [w777] mode=indexing
              tunnel: [w776] -> w743 mode=indexing if=w774
              i -> [w775]
              n284 = case shown="\"NG\"" w777 {
                tunnel: [2 ("CYCLE STATUS OK, NOK, ABORTED") 1 ("CYCLE STATUS OK, NOK, ABORTED") 0 ("CYCLE STATUS OK, NOK, ABORTED")] -> w776
                frame "NG" {
                }
                frame "OK" {
                }
                frame "-1", Default {
                }
              }
              n285 = Not Equal To 0?(x=w775) -> (x != 0?=w774:bool)
            }
            n286 = Index Array(array=w762, index #1=3 ("index"), index #2=4 ("index"), index #3=8 ("index"), index #4=7 ("index")) -> (element #1=w747:refnum<vi>, element #2=w746:refnum<vi>, element #3=w737:refnum<vi>, element #4=w736:refnum<vi>)
            n287 = Build Array(w747, w746, w737, w736) -> (w745:refnum<vi>[])
            n288 = for {
              tunnel: w745 -> [w786] mode=indexing
              shift-right: [w782] -> w759
              shift-left: w760 -> [w784]
              tunnel: w743 -> [w781] mode=indexing
              w785 = refnum<vi> refnum  # Boolean
              n289 = To More Specific Class(target class=w785, reference=w786, error in=w784) -> (specific class reference=w787:refnum<vi>, error out=w783:errorcluster)
              n290 = call "PADMINI_BOOL_COLOR_CHANGE.vi"("error in (no error)"=w783, "Numeric"=w781, "Boolean in"=w787) -> ("error out"=w782:errorcluster)  [unwired: 8 in]
            }
          }
          frame "SCAN5" {
            # "STATION OP 50"
            n291 = case shown="False" w838 {
              tunnel: w842 -> [w866 w900]
              tunnel: w841 -> [w858 w899]
              tunnel: w840 -> [_ _]
              tunnel: [w861 w898] -> w837
              tunnel: [w859 w900] -> w839
              tunnel: [w843 "" ("trimmed string")] -> w830
              frame False {
                n292 = call "PADMINI_AUTO_BARCODE_STRING 50.vi"("Enum"=enum16{"Read", "Write"}."Read", "error in (no error)"=w858) -> ("error out"=w857:errorcluster, "Input 2"=w845:string[])  [unwired: 8 in]
                n293 = global read "Global 1.vi" "BARCODE RECIPE"() -> (w846:string)
                n294 = Index Array(array=w845) -> (element=w844:string)  [unwired: 1 in]
                n295 = call <vilib>:"Trim Whitespace.vi"("string"=w844) -> ("trimmed string"=w843:string)  [unwired: 1 in]
                n296 = Match Pattern(string=w843, regular expression=w846) -> (match substring=w847:string)  [unwired: 1 in, 3 out]
                n297 = String Length(string=w846) -> (length=w849:i32)
                n298 = String Length(string=w847) -> (length=w848:i32)
                n299 = Format Into String(format string="WHERE BARCODE  ='%s'", w843) -> (resulting string=w853:string)  [unwired: 2 in, 1 out]
                n300 = Equal?(x=w849, y=w848) -> (x = y?=w850:bool)
                n301 = call <vilib>:"DB Tools Select Data.vi"("condition"=w853, "error in (no error)"=w857, "columns"=string[] ["BARCODE", "ST4_FINAL_RST", "ST5_FINAL_RST"], "table"="REPORT", "connection reference"=w866) -> ("error out"=w864:errorcluster, "data"=w863:variant[][], "connection reference out"=w859:T13)  [unwired: 1 in]
                n302 = call "PADMINI_varient_to_data.vi"("error in (no error)"=w864, "data"=w863) -> ("error out"=w862:errorcluster, "Array"=w860:string[][])  [unwired: 8 in]
                n303 = Equal?(x=w843, y="") -> (x = y?=w851:bool)
                n304 = case shown="True" w851 {
                  tunnel: w862 -> [w870 w894]
                  tunnel: [w869 w893] -> w861
                  tunnel: w860 -> [w868 _]
                  tunnel: w850 -> [w867 _]
                  frame False {
                    n305 = case shown="True" w867 {
                      tunnel: w870 -> [w874 w878]
                      tunnel: [w873 w877] -> w869
                      tunnel: w868 -> [_ w890]
                      frame False {
                        n306 = call "PADMINI_AUTO_BARCODE_STATUS 50.vi"("Enum"=enum16{"Read", "Write"}."Write", "error in (no error)"=w874, "I/P"=bool[] [FALSE, TRUE, FALSE, FALSE, FALSE]) -> ("error out"=w873:errorcluster)  [unwired: 7 in, 1 out]
                      }
                      frame True {
                        n307 = Index Array(array=w890, index (row) #1=0 ("index (row)"), index (col) #1=1 ("disabled index (col)"), index (row) #2=0 ("index (row)"), index (col) #2=2 ("disabled index (col)")) -> (element #1=w884:string)  [unwired: 1 out]
                        n308 = Empty String/Path?(string/path=w884) -> (empty?=w882:bool)
                        n309 = Equal?(x=w884, y="OK") -> (x = y?=w880:bool)
                        n310 = Not(x=w880) -> (.not. x?=w879:bool)
                        n311 = Build Array(TRUE ("element"), FALSE ("element"), w882, w880, w879) -> (w876:bool[])
                        n312 = call "PADMINI_AUTO_BARCODE_STATUS 50.vi"("Enum"=enum16{"Read", "Write"}."Write", "error in (no error)"=w878, "I/P"=w876) -> ("error out"=w877:errorcluster)  [unwired: 7 in, 1 out]
                      }
                    }
                  }
                  frame True {
                    n313 = call "PADMINI_AUTO_BARCODE_STATUS 50.vi"("Enum"=enum16{"Read", "Write"}."Write", "error in (no error)"=w894, "I/P"=bool[] [FALSE, FALSE, FALSE, FALSE, FALSE]) -> ("error out"=w893:errorcluster)  [unwired: 7 in, 1 out]
                  }
                }
              }
              frame True {
                n314 = call "PADMINI_AUTO_BARCODE_STATUS 50.vi"("Enum"=enum16{"Read", "Write"}."Write", "error in (no error)"=w899, "I/P"=bool[] [FALSE, FALSE, FALSE, FALSE, FALSE]) -> ("error out"=w898:errorcluster)  [unwired: 7 in, 1 out]
              }
            }
            n315 = flat-sequence {
              tunnel: [w902] -> w836
              tunnel: w837 -> [w902]
              frame #0 {
                # "UPDATE op 50 SCAN sTATUS"
                n316 = global write "DATA LOG.vi" "OP 50 Outputs"(TRUE) -> ()
              }
            }
            n317 = Bundle By Name(cluster=w832, "OP - 50.BARCODE"=w830) -> (w831:T11)
          }
          frame "DATALOG5" {
            w930 = T14 2 items=["no dialog", "OK message", "continue or stop message", "OK message + warnings", "continue/stop + warnings"] ("type of dialog (OK msg:1)")
            # "datalog of OP 50"
            n318 = call "PADMINI_AUTO_BARCODE_STRING 50.vi"("Enum"=enum16{"Read", "Write"}."Read", "error in (no error)"=w917) -> ("error out"=w919:errorcluster, "Input 2"=w908:string[])  [unwired: 8 in]
            n319 = call "PADMINI_AUTO_CYCLE VALUE 50.vi"("Enum"=enum16{"Read", "Write"}."Read", "error in (no error)"=w917) -> ("Input 2"=w913:dbl[])  [unwired: 8 in, 1 out]
            n320 = Index Array(array=w913) -> (element #1=w916:dbl, element #2=w915:dbl, element #3=w905:dbl)  [unwired: 3 in]
            n321 = Number To Fractional String(number=w913, precision (6)=i16 2) -> (F-format string=w912:string[])  [unwired: 2 in]
            n322 = case shown="True" w935 {
              tunnel: w936 -> [w967 w989]
              tunnel: w919 -> [w968 w988]
              tunnel: [w971 w987] -> w933
              tunnel: [w970 w986] -> w931
              tunnel: w934 -> [w966 _]
              tunnel: w912 -> [w962 w973]
              tunnel: w908 -> [w957 w972]
              frame False {
                # "DO TRACEBILITY"
                n323 = Index Array(array=w957) -> (element #1=w958:string, element #2=w954:string, element #3=w953:string, element #4=w952:string)  [unwired: 4 in]
                n324 = local read "SHIFT"() -> (w969:string)
                n325 = Index Array(array=w962) -> (element #1=w961:string, element #2=w956:string, element #3=w955:string)  [unwired: 3 in]
                n326 = call <vilib>:"Trim Whitespace.vi"("string"=w958) -> ("trimmed string"=w959:string)  [unwired: 1 in]
                n327 = call "PADMINI_SHIFT_DATE.vi"("SHIFT"=w969) -> ()  [unwired: 10 in, 1 out]
                n328 = Format Into String(format string="Where BARCODE='%s' ", w959) -> (resulting string=w964:string)  [unwired: 2 in, 1 out]
                n329 = Bundle("Input 2"=w961, "Input 2"=w954, "Input 2"=w956, "Input 2"=w953, "Input 2"=w955, "Input 2"=w952) -> (w960:T23)  [unwired: 1 in]
                n330 = call <vilib>:"DB Tools Update Data.vi"("condition"=w964, "data"=w960, "error in (no error)"=w968, "columns"=string[] ["ST5_SCREW1_DATA", "ST5_SCREW1_STATUS", "ST5_SCREW2_DATA", "ST5_SCREW2_STATUS", "ST5_SCREW3_DATA", "ST5_FINAL_RST"], "table"=w966, "connection reference"=w967) -> ("error out"=w970:errorcluster, "connection reference out"=w971:T13)  [unwired: 4 in]
              }
              frame True {
                # "TRAC BYPASS"
                n331 = local read "SHIFT"() -> (w974:string)
                n332 = Index Array(array=w972) -> (element #2=w978:string, element #3=w977:string, element #4=w982:string)  [unwired: 4 in, 1 out]
                n333 = Index Array(array=w973) -> (element #1=w981:string, element #2=w980:string, element #3=w979:string)  [unwired: 3 in]
                n334 = call "PADMINI_SHIFT_DATE.vi"("SHIFT"=w974) -> ("date/time string"=w975:string)  [unwired: 10 in]
                n335 = Bundle("date/time string"=w975, "SHIFT"=w974, "Input 2"=w981, "Input 2"=w978, "Input 2"=w980, "Input 2"=w977, "Input 2"=w979, "Input 2"=w982) -> (w976:T24)  [unwired: 1 in]
                n336 = To Variant(anything=w976) -> (Variant=w985:variant)
                n337 = call <vilib>:"DB Tools Insert Data.vi"("data"=w985, "error in (no error)"=w988, "columns"=string[] ["DATE", "SHIFT", "ST5_SCREW1_DATA", "ST5_SCREW1_STATUS", "ST5_SCREW2_DATA", "ST5_SCREW2_STATUS", "ST5_SCREW3_DATA", "ST5_FINAL_RST"], "table"="ST5_REPORT", "connection reference"=w989) -> ("error out"=w986:errorcluster, "connection reference out"=w987:T13)  [unwired: 5 in]
              }
            }
            n338 = Bundle By Name(cluster=w922, "OP - 50.Screw 1 Data"=w916, "OP - 50.Screw 2 data"=w915, "OP - 50.Screw 3 Data"=w905) -> (w921:T11)
            n339 = call <vilib>:"Simple Error Handler.vi"("type of dialog (OK msg:1)"=w930, "error in (no error)"=w931) -> ("error out"=w929:errorcluster)  [unwired: 3 in, 4 out]
            n340 = call <vilib>:"Clear Errors.vi"("error in (no error)"=w929) -> ("error out"=w927:errorcluster)  [unwired: 5 in, 1 out]
            n341 = property on="OP - 50" class="Clust"(error in=w927) -> (error out=w924:errorcluster, "Controls[]"=w926:refnum<vi>[])  [unwired: 1 in, 1 out]
            n342 = for {
              tunnel: w908 -> [w941] mode=indexing
              tunnel: [w940] -> w907 mode=indexing if=w938
              i -> [w939]
              n343 = case shown="\"NG\"" w941 {
                tunnel: [2 ("CYCLE STATUS OK, NOK, ABORTED") 1 ("CYCLE STATUS OK, NOK, ABORTED") 0 ("CYCLE STATUS OK, NOK, ABORTED")] -> w940
                frame "NG" {
                }
                frame "OK" {
                }
                frame "-1", Default {
                }
              }
              n344 = Not Equal To 0?(x=w939) -> (x != 0?=w938:bool)
            }
            n345 = Index Array(array=w926, index #1=3 ("index"), index #2=4 ("index"), index #3=6 ("index")) -> (element #1=w911:refnum<vi>, element #2=w910:refnum<vi>, element #3=w903:refnum<vi>)
            n346 = Build Array(w911, w910, w903) -> (w909:refnum<vi>[])
            n347 = for {
              tunnel: w909 -> [w950] mode=indexing
              shift-right: [w946] -> w923
              shift-left: w924 -> [w948]
              tunnel: w907 -> [w945] mode=indexing
              w949 = refnum<vi> refnum  # Boolean
              n348 = To More Specific Class(target class=w949, reference=w950, error in=w948) -> (specific class reference=w951:refnum<vi>, error out=w947:errorcluster)
              n349 = call "PADMINI_BOOL_COLOR_CHANGE.vi"("error in (no error)"=w947, "Numeric"=w945, "Boolean in"=w951) -> ("error out"=w946:errorcluster)  [unwired: 8 in]
            }
          }
          frame "SCAN6" {
            # "STATION OP 60"
            n350 = case shown="True" w998 {
              tunnel: w1002 -> [w1026 w1060]
              tunnel: w1001 -> [w1018 w1059]
              tunnel: w1000 -> [_ _]
              tunnel: [w1021 w1058] -> w997
              tunnel: [w1019 w1060] -> w999
              tunnel: [w1003 "" ("trimmed string")] -> w990
              frame False {
                n351 = call "PADMINI_AUTO_BARCODE_STRING 60.vi"("Enum"=enum16{"Read", "Write"}."Read", "error in (no error)"=w1018) -> ("error out"=w1017:errorcluster, "Input 2"=w1005:string[])  [unwired: 8 in]
                n352 = global read "Global 1.vi" "BARCODE RECIPE"() -> (w1006:string)
                n353 = Index Array(array=w1005) -> (element=w1004:string)  [unwired: 1 in]
                n354 = call <vilib>:"Trim Whitespace.vi"("string"=w1004) -> ("trimmed string"=w1003:string)  [unwired: 1 in]
                n355 = Match Pattern(string=w1003, regular expression=w1006) -> (match substring=w1007:string)  [unwired: 1 in, 3 out]
                n356 = String Length(string=w1006) -> (length=w1009:i32)
                n357 = String Length(string=w1007) -> (length=w1008:i32)
                n358 = Format Into String(format string="WHERE BARCODE  ='%s'", w1003) -> (resulting string=w1013:string)  [unwired: 2 in, 1 out]
                n359 = Equal?(x=w1009, y=w1008) -> (x = y?=w1010:bool)
                n360 = call <vilib>:"DB Tools Select Data.vi"("condition"=w1013, "error in (no error)"=w1017, "columns"=string[] ["BARCODE", "ST5_FINAL_RST", "ST6_FINAL_RST"], "table"="REPORT", "connection reference"=w1026) -> ("error out"=w1024:errorcluster, "data"=w1023:variant[][], "connection reference out"=w1019:T13)  [unwired: 1 in]
                n361 = call "PADMINI_varient_to_data.vi"("error in (no error)"=w1024, "data"=w1023) -> ("error out"=w1022:errorcluster, "Array"=w1020:string[][])  [unwired: 8 in]
                n362 = Equal?(x=w1003, y="") -> (x = y?=w1011:bool)
                n363 = case shown="False" w1011 {
                  tunnel: w1022 -> [w1030 w1054]
                  tunnel: [w1029 w1053] -> w1021
                  tunnel: w1020 -> [w1028 _]
                  tunnel: w1010 -> [w1027 _]
                  frame False {
                    n364 = case shown="True" w1027 {
                      tunnel: w1030 -> [w1034 w1038]
                      tunnel: [w1033 w1037] -> w1029
                      tunnel: w1028 -> [_ w1050]
                      frame False {
                        n365 = call "PADMINI_AUTO_BARCODE_STATUS 60.vi"("Enum"=enum16{"Read", "Write"}."Write", "error in (no error)"=w1034, "I/P"=bool[] [FALSE, TRUE, FALSE, FALSE, FALSE]) -> ("error out"=w1033:errorcluster)  [unwired: 7 in, 1 out]
                      }
                      frame True {
                        n366 = Index Array(array=w1050, index (row) #1=0 ("index (row)"), index (col) #1=1 ("disabled index (col)"), index (row) #2=0 ("index (row)"), index (col) #2=2 ("disabled index (col)")) -> (element #1=w1044:string)  [unwired: 1 out]
                        n367 = Empty String/Path?(string/path=w1044) -> (empty?=w1042:bool)
                        n368 = Equal?(x=w1044, y="OK") -> (x = y?=w1040:bool)
                        n369 = Not(x=w1040) -> (.not. x?=w1039:bool)
                        n370 = Build Array(TRUE ("element"), FALSE ("element"), w1042, w1040, w1039) -> (w1036:bool[])
                        n371 = call "PADMINI_AUTO_BARCODE_STATUS 60.vi"("Enum"=enum16{"Read", "Write"}."Write", "error in (no error)"=w1038, "I/P"=w1036) -> ("error out"=w1037:errorcluster)  [unwired: 7 in, 1 out]
                      }
                    }
                  }
                  frame True {
                    n372 = call "PADMINI_AUTO_BARCODE_STATUS 60.vi"("Enum"=enum16{"Read", "Write"}."Write", "error in (no error)"=w1054, "I/P"=bool[] [FALSE, FALSE, FALSE, FALSE, FALSE]) -> ("error out"=w1053:errorcluster)  [unwired: 7 in, 1 out]
                  }
                }
              }
              frame True {
                n373 = call "PADMINI_AUTO_BARCODE_STATUS 60.vi"("Enum"=enum16{"Read", "Write"}."Write", "error in (no error)"=w1059, "I/P"=bool[] [FALSE, FALSE, FALSE, FALSE, FALSE]) -> ("error out"=w1058:errorcluster)  [unwired: 7 in, 1 out]
              }
            }
            n374 = flat-sequence {
              tunnel: [w1062] -> w996
              tunnel: w997 -> [w1062]
              frame #0 {
                # "UPDATE op 60 SCAN sTATUS"
                n375 = global write "DATA LOG.vi" "OP 60 Outputs"(TRUE) -> ()
              }
            }
            n376 = Bundle By Name(cluster=w992, "OP - 60.BARCODE"=w990) -> (w991:T11)
          }
          frame "DATALOG6" {
            w1101 = T14 2 items=["no dialog", "OK message", "continue or stop message", "OK message + warnings", "continue/stop + warnings"] ("type of dialog (OK msg:1)")
            # "datalog of OP 60"
            n377 = call "PADMINI_AUTO_BARCODE_STRING 60.vi"("Enum"=enum16{"Read", "Write"}."Read", "error in (no error)"=w1088) -> ("error out"=w1090:errorcluster, "Input 2"=w1079:string[])  [unwired: 8 in]
            n378 = call "PADMINI_AUTO_CYCLE VALUE 60.vi"("Enum"=enum16{"Read", "Write"}."Read", "error in (no error)"=w1088) -> ("Input 2"=w1084:dbl[])  [unwired: 8 in, 1 out]
            n379 = Index Array(array=w1084) -> (element #1=w1087:dbl, element #2=w1086:dbl, element #3=w1076:dbl, element #4=w1073:dbl, element #5=w1072:dbl, element #6=w1071:dbl)  [unwired: 6 in]
            n380 = Number To Fractional String(number=w1084, precision (6)=i16 2) -> (F-format string=w1083:string[])  [unwired: 2 in]
            n381 = case shown="True" w1106 {
              tunnel: w1107 -> [w1144 w1172]
              tunnel: w1090 -> [w1145 w1171]
              tunnel: [w1148 w1170] -> w1104
              tunnel: [w1147 w1169] -> w1102
              tunnel: w1105 -> [w1143 _]
              tunnel: w1083 -> [w1139 w1152]
              tunnel: w1079 -> [w1134 w1151]
              frame False {
                # "DO TRACEBILITY"
                n382 = Index Array(array=w1134) -> (element #1=w1135:string, element #2=w1131:string, element #3=w1130:string, element #4=w1129:string, element #5=w1127:string, element #6=w1124:string, element #7=w1123:string)  [unwired: 7 in]
                n383 = local read "SHIFT"() -> (w1146:string)
                n384 = Index Array(array=w1139) -> (element #1=w1138:string, element #2=w1133:string, element #3=w1132:string, element #4=w1128:string, element #5=w1126:string, element #6=w1125:string)  [unwired: 6 in]
                n385 = call <vilib>:"Trim Whitespace.vi"("string"=w1135) -> ("trimmed string"=w1136:string)  [unwired: 1 in]
                n386 = call "PADMINI_SHIFT_DATE.vi"("SHIFT"=w1146) -> ()  [unwired: 10 in, 1 out]
                n387 = Format Into String(format string="Where BARCODE='%s' ", w1136) -> (resulting string=w1141:string)  [unwired: 2 in, 1 out]
                n388 = Bundle("Input 2"=w1138, "Input 2"=w1131, "Input 2"=w1133, "Input 2"=w1130, "Input 2"=w1132, "Input 2"=w1129, "Input 2"=w1128, "Input 2"=w1127, "Input 2"=w1126, "Input 2"=w1125, "Input 2"=w1124, "Input 2"=w1123) -> (w1137:T25)  [unwired: 1 in]
                n389 = call <vilib>:"DB Tools Update Data.vi"("condition"=w1141, "data"=w1137, "error in (no error)"=w1145, "columns"=string[] ["ST6_SCREW1_DATA", "ST6_SCREW1_STATUS", "ST6_SCREW2_DATA", "ST6_SCREW2_STATUS", "ST6_SCREW3_DATA", "ST6_SCREW3_STATUS", "ST6_SCREW4_DATA", "ST6_SCREW4_STATUS", "ST6_SCREW5_DATA", "ST6_SCREW5_STATUS", "ST6_SCREW6_DATA", "ST6_SCREW6_STATUS", "ST6_FINAL_RST"], "table"=w1143, "connection reference"=w1144) -> ("error out"=w1147:errorcluster, "connection reference out"=w1148:T13)  [unwired: 4 in]
              }
              frame True {
                # "TRAC BYPASS"
                n390 = local read "SHIFT"() -> (w1149:string)
                n391 = call "PADMINI_SHIFT_DATE.vi"("SHIFT"=w1149) -> ("date/time string"=w1150:string)  [unwired: 10 in]
                n392 = Index Array(array=w1151) -> (element #2=w1160:string, element #3=w1159:string, element #4=w1158:string, element #5=w1156:string, element #6=w1164:string, element #7=w1165:string)  [unwired: 7 in, 1 out]
                n393 = Index Array(array=w1152) -> (element #1=w1163:string, element #2=w1162:string, element #3=w1161:string, element #4=w1157:string, element #5=w1155:string, element #6=w1154:string)  [unwired: 6 in]
                n394 = Bundle("date/time string"=w1150, "SHIFT"=w1149, "Input 2"=w1163, "Input 2"=w1160, "Input 2"=w1162, "Input 2"=w1159, "Input 2"=w1161, "Input 2"=w1158, "Input 2"=w1157, "Input 2"=w1156, "Input 2"=w1155, "Input 2"=w1154, "Input 2"=w1164, "Input 2"=w1165) -> (w1153:T26)  [unwired: 1 in]
                n395 = To Variant(anything=w1153) -> (Variant=w1168:variant)
                n396 = call <vilib>:"DB Tools Insert Data.vi"("data"=w1168, "error in (no error)"=w1171, "columns"=string[] ["DATE", "SHIFT", "ST6_SCREW1_DATA", "ST6_SCREW1_STATUS", "ST6_SCREW2_DATA", "ST6_SCREW2_STATUS", "ST6_SCREW3_DATA", "ST6_SCREW3_STATUS", "ST6_SCREW4_DATA", "ST6_SCREW4_STATUS", "ST6_SCREW5_DATA", "ST6_SCREW5_STATUS", "ST6_SCREW6_DATA", "ST6_SCREW6_STATUS", "ST6_FINAL_RST"], "table"="ST6_REPORT", "connection reference"=w1172) -> ("error out"=w1169:errorcluster, "connection reference out"=w1170:T13)  [unwired: 5 in]
              }
            }
            n397 = Bundle By Name(cluster=w1093, "OP - 60.Screw 1 Data"=w1087, "OP - 60.Screw 2 data"=w1086, "OP - 60.Screw3 Data"=w1076, "OP - 60.Screw4 Data"=w1073, "OP - 60.Screw5 Data"=w1072, "OP - 60.Screw6 Data"=w1071) -> (w1092:T11)
            n398 = call <vilib>:"Simple Error Handler.vi"("type of dialog (OK msg:1)"=w1101, "error in (no error)"=w1102) -> ("error out"=w1100:errorcluster)  [unwired: 3 in, 4 out]
            n399 = call <vilib>:"Clear Errors.vi"("error in (no error)"=w1100) -> ("error out"=w1098:errorcluster)  [unwired: 5 in, 1 out]
            n400 = property on="OP - 60" class="Clust"(error in=w1098) -> (error out=w1095:errorcluster, "Controls[]"=w1097:refnum<vi>[])  [unwired: 1 in, 1 out]
            n401 = for {
              tunnel: w1079 -> [w1112] mode=indexing
              tunnel: [w1111] -> w1078 mode=indexing if=w1109
              i -> [w1110]
              n402 = case shown="\"NG\"" w1112 {
                tunnel: [2 ("CYCLE STATUS OK, NOK, ABORTED") 1 ("CYCLE STATUS OK, NOK, ABORTED") 0 ("CYCLE STATUS OK, NOK, ABORTED")] -> w1111
                frame "NG" {
                }
                frame "OK" {
                }
                frame "-1", Default {
                }
              }
              n403 = Not Equal To 0?(x=w1110) -> (x != 0?=w1109:bool)
            }
            n404 = Index Array(array=w1097, index #1=3 ("index"), index #2=4 ("index"), index #3=7 ("index"), index #4=10 ("index"), index #5=11 ("index"), index #6=13 ("index"), index #7=6 ("index")) -> (element #1=w1082:refnum<vi>, element #2=w1081:refnum<vi>, element #3=w1074:refnum<vi>, element #4=w1067:refnum<vi>, element #5=w1066:refnum<vi>, element #6=w1065:refnum<vi>, element #7=w1063:refnum<vi>)
            n405 = Build Array(w1082, w1081, w1074, w1067, w1066, w1065, w1063) -> (w1080:refnum<vi>[])
            n406 = for {
              tunnel: w1080 -> [w1121] mode=indexing
              shift-right: [w1117] -> w1094
              shift-left: w1095 -> [w1119]
              tunnel: w1078 -> [w1116] mode=indexing
              w1120 = refnum<vi> refnum  # Boolean
              n407 = To More Specific Class(target class=w1120, reference=w1121, error in=w1119) -> (specific class reference=w1122:refnum<vi>, error out=w1118:errorcluster)
              n408 = call "PADMINI_BOOL_COLOR_CHANGE.vi"("error in (no error)"=w1118, "Numeric"=w1116, "Boolean in"=w1122) -> ("error out"=w1117:errorcluster)  [unwired: 8 in]
            }
          }
          frame "SCAN7" {
            # "STATION OP 70"
            n409 = case shown="True" w1181 {
              tunnel: w1185 -> [w1209 w1243]
              tunnel: w1184 -> [w1201 w1242]
              tunnel: w1183 -> [_ _]
              tunnel: [w1204 w1241] -> w1180
              tunnel: [w1202 w1243] -> w1182
              tunnel: [w1186 "" ("trimmed string")] -> w1173
              frame False {
                n410 = call "PADMINI_AUTO_BARCODE_STRING 70.vi"("Enum"=enum16{"Read", "Write"}."Read", "error in (no error)"=w1201) -> ("error out"=w1200:errorcluster, "Input 2"=w1188:string[])  [unwired: 8 in]
                n411 = global read "Global 1.vi" "BARCODE RECIPE"() -> (w1189:string)
                n412 = Index Array(array=w1188) -> (element=w1187:string)  [unwired: 1 in]
                n413 = call <vilib>:"Trim Whitespace.vi"("string"=w1187) -> ("trimmed string"=w1186:string)  [unwired: 1 in]
                n414 = Match Pattern(string=w1186, regular expression=w1189) -> (match substring=w1190:string)  [unwired: 1 in, 3 out]
                n415 = String Length(string=w1189) -> (length=w1192:i32)
                n416 = String Length(string=w1190) -> (length=w1191:i32)
                n417 = Format Into String(format string="WHERE BARCODE  ='%s'", w1186) -> (resulting string=w1196:string)  [unwired: 2 in, 1 out]
                n418 = Equal?(x=w1192, y=w1191) -> (x = y?=w1193:bool)
                n419 = call <vilib>:"DB Tools Select Data.vi"("condition"=w1196, "error in (no error)"=w1200, "columns"=string[] ["BARCODE", "ST6_FINAL_RST", "ST7_FINAL_RST"], "table"="REPORT", "connection reference"=w1209) -> ("error out"=w1207:errorcluster, "data"=w1206:variant[][], "connection reference out"=w1202:T13)  [unwired: 1 in]
                n420 = call "PADMINI_varient_to_data.vi"("error in (no error)"=w1207, "data"=w1206) -> ("error out"=w1205:errorcluster, "Array"=w1203:string[][])  [unwired: 8 in]
                n421 = Equal?(x=w1186, y="") -> (x = y?=w1194:bool)
                n422 = case shown="False" w1194 {
                  tunnel: w1205 -> [w1213 w1237]
                  tunnel: [w1212 w1236] -> w1204
                  tunnel: w1203 -> [w1211 _]
                  tunnel: w1193 -> [w1210 _]
                  frame False {
                    n423 = case shown="False" w1210 {
                      tunnel: w1213 -> [w1217 w1221]
                      tunnel: [w1216 w1220] -> w1212
                      tunnel: w1211 -> [_ w1233]
                      frame False {
                        n424 = call "PADMINI_AUTO_BARCODE_STATUS 70.vi"("Enum"=enum16{"Read", "Write"}."Write", "error in (no error)"=w1217, "I/P"=bool[] [FALSE, TRUE, FALSE, FALSE, FALSE]) -> ("error out"=w1216:errorcluster)  [unwired: 7 in, 1 out]
                      }
                      frame True {
                        n425 = Index Array(array=w1233, index (row) #1=0 ("index (row)"), index (col) #1=1 ("disabled index (col)"), index (row) #2=0 ("index (row)"), index (col) #2=2 ("disabled index (col)")) -> (element #1=w1227:string)  [unwired: 1 out]
                        n426 = Empty String/Path?(string/path=w1227) -> (empty?=w1225:bool)
                        n427 = Equal?(x=w1227, y="OK") -> (x = y?=w1223:bool)
                        n428 = Not(x=w1223) -> (.not. x?=w1222:bool)
                        n429 = Build Array(TRUE ("element"), FALSE ("element"), w1225, w1223, w1222) -> (w1219:bool[])
                        n430 = call "PADMINI_AUTO_BARCODE_STATUS 70.vi"("Enum"=enum16{"Read", "Write"}."Write", "error in (no error)"=w1221, "I/P"=w1219) -> ("error out"=w1220:errorcluster)  [unwired: 7 in, 1 out]
                      }
                    }
                  }
                  frame True {
                    n431 = call "PADMINI_AUTO_BARCODE_STATUS 70.vi"("Enum"=enum16{"Read", "Write"}."Write", "error in (no error)"=w1237, "I/P"=bool[] [FALSE, FALSE, FALSE, FALSE, FALSE]) -> ("error out"=w1236:errorcluster)  [unwired: 7 in, 1 out]
                  }
                }
              }
              frame True {
                n432 = call "PADMINI_AUTO_BARCODE_STATUS 70.vi"("Enum"=enum16{"Read", "Write"}."Write", "error in (no error)"=w1242, "I/P"=bool[] [FALSE, FALSE, FALSE, FALSE, FALSE]) -> ("error out"=w1241:errorcluster)  [unwired: 7 in, 1 out]
              }
            }
            n433 = flat-sequence {
              tunnel: [w1245] -> w1179
              tunnel: w1180 -> [w1245]
              frame #0 {
                # "UPDATE op 70 SCAN sTATUS"
                n434 = global write "DATA LOG.vi" "OP 70 Outputs"(TRUE) -> ()
              }
            }
            n435 = Bundle By Name(cluster=w1175, "OP - 70.BARCODE"=w1173) -> (w1174:T11)
          }
          frame "DATALOG7" {
            w1268 = T14 2 items=["no dialog", "OK message", "continue or stop message", "OK message + warnings", "continue/stop + warnings"] ("type of dialog (OK msg:1)")
            # "datalog of OP 70"
            n436 = call "PADMINI_AUTO_BARCODE_STRING 70.vi"("Enum"=enum16{"Read", "Write"}."Read", "error in (no error)"=w1255) -> ("error out"=w1257:errorcluster, "Input 2"=w1247:string[])  [unwired: 8 in]
            n437 = call "PADMINI_AUTO_CYCLE VALUE 70.vi"("Enum"=enum16{"Read", "Write"}."Read", "error in (no error)"=w1255) -> ("Input 2"=w1251:dbl[])  [unwired: 8 in, 1 out]
            n438 = Index Array(array=w1251) -> (element #1=w1254:dbl, element #2=w1253:dbl)  [unwired: 2 in]
            n439 = Number To Fractional String(number=w1251, precision (6)=i16 2) -> (F-format string=w1250:string[])  [unwired: 2 in]
            n440 = case shown="True" w1273 {
              tunnel: w1274 -> [w1302 w1320]
              tunnel: w1257 -> [w1303 w1319]
              tunnel: [w1305 w1318] -> w1271
              tunnel: [w1304 w1317] -> w1269
              tunnel: w1272 -> [w1301 _]
              tunnel: w1250 -> [w1297 w1307]
              tunnel: w1247 -> [w1292 w1306]
              frame False {
                # "DO TRACEBILITY"
                n441 = Index Array(array=w1292) -> (element #1=w1293:string, element #2=w1291:string)  [unwired: 2 in]
                n442 = call <vilib>:"Trim Whitespace.vi"("string"=w1293) -> ("trimmed string"=w1294:string)  [unwired: 1 in]
                n443 = Index Array(array=w1297) -> (element #1=w1296:string, element #2=w1290:string)  [unwired: 2 in]
                n444 = Bundle("Input 2"=w1296, "Input 2"=w1290, "Input 2"=w1291) -> (w1295:T27)  [unwired: 1 in]
                n445 = Format Into String(format string="Where BARCODE='%s' ", w1294) -> (resulting string=w1299:string)  [unwired: 2 in, 1 out]
                n446 = call <vilib>:"DB Tools Update Data.vi"("condition"=w1299, "data"=w1295, "error in (no error)"=w1303, "columns"=string[] ["ST7_SENSOR_MIN_VLTG", "ST7_SENSOR_MAX_VLTG", "ST7_FINAL_RST"], "table"=w1301, "connection reference"=w1302) -> ("error out"=w1304:errorcluster, "connection reference out"=w1305:T13)  [unwired: 4 in]
              }
              frame True {
                # "TRAC BYPASS"
                n447 = local read "SHIFT"() -> (w1308:string)
                n448 = call "PADMINI_SHIFT_DATE.vi"("SHIFT"=w1308) -> ("date/time string"=w1309:string)  [unwired: 10 in]
                n449 = Index Array(array=w1306) -> (element #2=w1312:string)  [unwired: 2 in, 1 out]
                n450 = Index Array(array=w1307) -> (element #1=w1313:string, element #2=w1311:string)  [unwired: 2 in]
                n451 = Bundle("date/time string"=w1309, "SHIFT"=w1308, "Input 2"=w1313, "Input 2"=w1311, "Input 2"=w1312) -> (w1310:T28)  [unwired: 1 in]
                n452 = To Variant(anything=w1310) -> (Variant=w1316:variant)
                n453 = call <vilib>:"DB Tools Insert Data.vi"("data"=w1316, "error in (no error)"=w1319, "columns"=string[] ["DATE", "SHIFT", "ST7_SENSOR_MIN_VLTG", "ST7_SENSOR_MAX_VLTG", "ST7_FINAL_RST"], "table"="ST7_REPORT", "connection reference"=w1320) -> ("error out"=w1317:errorcluster, "connection reference out"=w1318:T13)  [unwired: 5 in]
              }
            }
            n454 = Bundle By Name(cluster=w1260, "OP - 70.Sensor MIN Vltg"=w1254, "OP - 70.Sensor MAX Vltg"=w1253) -> (w1259:T11)
            n455 = call <vilib>:"Simple Error Handler.vi"("type of dialog (OK msg:1)"=w1268, "error in (no error)"=w1269) -> ("error out"=w1267:errorcluster)  [unwired: 3 in, 4 out]
            n456 = call <vilib>:"Clear Errors.vi"("error in (no error)"=w1267) -> ("error out"=w1265:errorcluster)  [unwired: 5 in, 1 out]
            n457 = property on="OP - 70" class="Clust"(error in=w1265) -> (error out=w1262:errorcluster, "Controls[]"=w1264:refnum<vi>[])  [unwired: 1 in, 1 out]
            n458 = for {
              tunnel: w1247 -> [w1279] mode=indexing
              tunnel: [w1278] -> w1246 mode=indexing if=w1276
              i -> [w1277]
              n459 = case shown="\"NG\"" w1279 {
                tunnel: [2 ("CYCLE STATUS OK, NOK, ABORTED") 1 ("CYCLE STATUS OK, NOK, ABORTED") 0 ("CYCLE STATUS OK, NOK, ABORTED")] -> w1278
                frame "NG" {
                }
                frame "OK" {
                }
                frame "-1", Default {
                }
              }
              n460 = Not Equal To 0?(x=w1277) -> (x != 0?=w1276:bool)
            }
            n461 = Index Array(array=w1264, index=3) -> (element=w1249:refnum<vi>)
            n462 = Build Array(w1249) -> (w1248:refnum<vi>[])
            n463 = for {
              tunnel: w1248 -> [w1288] mode=indexing
              shift-right: [w1284] -> w1261
              shift-left: w1262 -> [w1286]
              tunnel: w1246 -> [w1283] mode=indexing
              w1287 = refnum<vi> refnum  # Boolean
              n464 = To More Specific Class(target class=w1287, reference=w1288, error in=w1286) -> (specific class reference=w1289:refnum<vi>, error out=w1285:errorcluster)
              n465 = call "PADMINI_BOOL_COLOR_CHANGE.vi"("error in (no error)"=w1285, "Numeric"=w1283, "Boolean in"=w1289) -> ("error out"=w1284:errorcluster)  [unwired: 8 in]
            }
          }
          frame "SCAN8" {
            # "STATION OP 80"
            n466 = case shown="True" w1329 {
              tunnel: w1333 -> [w1357 w1391]
              tunnel: w1332 -> [w1349 w1390]
              tunnel: w1331 -> [_ _]
              tunnel: [w1352 w1389] -> w1328
              tunnel: [w1350 w1391] -> w1330
              tunnel: [w1334 "" ("trimmed string")] -> w1321
              frame False {
                n467 = call "PADMINI_AUTO_BARCODE_STRING 80.vi"("Enum"=enum16{"Read", "Write"}."Read", "error in (no error)"=w1349) -> ("error out"=w1348:errorcluster, "Input 2"=w1336:string[])  [unwired: 8 in]
                n468 = global read "Global 1.vi" "BARCODE RECIPE"() -> (w1337:string)
                n469 = Index Array(array=w1336) -> (element=w1335:string)  [unwired: 1 in]
                n470 = call <vilib>:"Trim Whitespace.vi"("string"=w1335) -> ("trimmed string"=w1334:string)  [unwired: 1 in]
                n471 = Match Pattern(string=w1334, regular expression=w1337) -> (match substring=w1338:string)  [unwired: 1 in, 3 out]
                n472 = String Length(string=w1337) -> (length=w1340:i32)
                n473 = String Length(string=w1338) -> (length=w1339:i32)
                n474 = Format Into String(format string="WHERE BARCODE  ='%s'", w1334) -> (resulting string=w1344:string)  [unwired: 2 in, 1 out]
                n475 = Equal?(x=w1340, y=w1339) -> (x = y?=w1341:bool)
                n476 = call <vilib>:"DB Tools Select Data.vi"("condition"=w1344, "error in (no error)"=w1348, "columns"=string[] ["BARCODE", "ST7_FINAL_RST", "ST8_FINAL_RST"], "table"="REPORT", "connection reference"=w1357) -> ("error out"=w1355:errorcluster, "data"=w1354:variant[][], "connection reference out"=w1350:T13)  [unwired: 1 in]
                n477 = call "PADMINI_varient_to_data.vi"("error in (no error)"=w1355, "data"=w1354) -> ("error out"=w1353:errorcluster, "Array"=w1351:string[][])  [unwired: 8 in]
                n478 = Equal?(x=w1334, y="") -> (x = y?=w1342:bool)
                n479 = case shown="True" w1342 {
                  tunnel: w1353 -> [w1361 w1385]
                  tunnel: [w1360 w1384] -> w1352
                  tunnel: w1351 -> [w1359 _]
                  tunnel: w1341 -> [w1358 _]
                  frame False {
                    n480 = case shown="True" w1358 {
                      tunnel: w1361 -> [w1365 w1369]
                      tunnel: [w1364 w1368] -> w1360
                      tunnel: w1359 -> [_ w1381]
                      frame False {
                        n481 = call "PADMINI_AUTO_BARCODE_STATUS 80.vi"("Enum"=enum16{"Read", "Write"}."Write", "error in (no error)"=w1365, "I/P"=bool[] [FALSE, TRUE, FALSE, FALSE, FALSE]) -> ("error out"=w1364:errorcluster)  [unwired: 7 in, 1 out]
                      }
                      frame True {
                        n482 = Index Array(array=w1381, index (row) #1=0 ("index (row)"), index (col) #1=1 ("disabled index (col)"), index (row) #2=0 ("index (row)"), index (col) #2=2 ("disabled index (col)")) -> (element #1=w1375:string)  [unwired: 1 out]
                        n483 = Empty String/Path?(string/path=w1375) -> (empty?=w1373:bool)
                        n484 = Equal?(x=w1375, y="OK") -> (x = y?=w1371:bool)
                        n485 = Not(x=w1371) -> (.not. x?=w1370:bool)
                        n486 = Build Array(TRUE ("element"), FALSE ("element"), w1373, w1371, w1370) -> (w1367:bool[])
                        n487 = call "PADMINI_AUTO_BARCODE_STATUS 80.vi"("Enum"=enum16{"Read", "Write"}."Write", "error in (no error)"=w1369, "I/P"=w1367) -> ("error out"=w1368:errorcluster)  [unwired: 7 in, 1 out]
                      }
                    }
                  }
                  frame True {
                    n488 = call "PADMINI_AUTO_BARCODE_STATUS 80.vi"("Enum"=enum16{"Read", "Write"}."Write", "error in (no error)"=w1385, "I/P"=bool[] [FALSE, FALSE, FALSE, FALSE, FALSE]) -> ("error out"=w1384:errorcluster)  [unwired: 7 in, 1 out]
                  }
                }
              }
              frame True {
                n489 = call "PADMINI_AUTO_BARCODE_STATUS 80.vi"("Enum"=enum16{"Read", "Write"}."Write", "error in (no error)"=w1390, "I/P"=bool[] [FALSE, FALSE, FALSE, FALSE, FALSE]) -> ("error out"=w1389:errorcluster)  [unwired: 7 in, 1 out]
              }
            }
            n490 = flat-sequence {
              tunnel: [w1393] -> w1327
              tunnel: w1328 -> [w1393]
              frame #0 {
                # "UPDATE op 80 SCAN sTATUS"
                n491 = global write "DATA LOG.vi" "OP 80 Outputs"(TRUE) -> ()
              }
            }
            n492 = Bundle By Name(cluster=w1323, "OP - 80.BARCODE"=w1321) -> (w1322:T11)
          }
          frame "DATALOG8" {
            w1417 = T14 2 items=["no dialog", "OK message", "continue or stop message", "OK message + warnings", "continue/stop + warnings"] ("type of dialog (OK msg:1)")
            # "datalog of OP 80"
            n493 = call "PADMINI_AUTO_BARCODE_STRING 80.vi"("Enum"=enum16{"Read", "Write"}."Read", "error in (no error)"=w1404) -> ("error out"=w1406:errorcluster, "Input 2"=w1397:string[])  [unwired: 8 in]
            n494 = call "PADMINI_AUTO_CYCLE VALUE 80.vi"("Enum"=enum16{"Read", "Write"}."Read", "error in (no error)"=w1404) -> ("Input 2"=w1401:dbl[])  [unwired: 8 in, 1 out]
            n495 = Index Array(array=w1401) -> (element=w1403:dbl)  [unwired: 1 in]
            n496 = Number To Fractional String(number=w1401, precision (6)=i16 2) -> (F-format string=w1400:string[])  [unwired: 2 in]
            n497 = case shown="True" w1422 {
              tunnel: w1423 -> [w1451 w1469]
              tunnel: w1406 -> [w1452 w1468]
              tunnel: [w1454 w1467] -> w1420
              tunnel: [w1453 w1466] -> w1418
              tunnel: w1421 -> [w1450 _]
              tunnel: w1400 -> [w1446 w1457]
              tunnel: w1397 -> [w1442 w1458]
              frame False {
                # "DO TRACEBILITY"
                n498 = Index Array(array=w1442) -> (element #1=w1443:string, element #2=w1441:string, element #3=w1440:string)  [unwired: 3 in]
                n499 = call <vilib>:"Trim Whitespace.vi"("string"=w1443) -> ("trimmed string"=w1444:string)  [unwired: 1 in]
                n500 = Index Array(array=w1446) -> (element=w1439:string)  [unwired: 1 in]
                n501 = Bundle("Input 2"=w1439, "Input 2"=w1441, "Input 2"=w1440) -> (w1445:T27)  [unwired: 1 in]
                n502 = Format Into String(format string="Where BARCODE='%s' ", w1444) -> (resulting string=w1448:string)  [unwired: 2 in, 1 out]
                n503 = call <vilib>:"DB Tools Update Data.vi"("condition"=w1448, "data"=w1445, "error in (no error)"=w1452, "columns"=string[] ["ST8_DISPENSING", "ST8_LOAD", "ST8_FINAL_RST"], "table"=w1450, "connection reference"=w1451) -> ("error out"=w1453:errorcluster, "connection reference out"=w1454:T13)  [unwired: 4 in]
              }
              frame True {
                # "TRAC BYPASS"
                n504 = local read "SHIFT"() -> (w1455:string)
                n505 = call "PADMINI_SHIFT_DATE.vi"("SHIFT"=w1455) -> ("date/time string"=w1456:string)  [unwired: 10 in]
                n506 = Index Array(array=w1458) -> (element #2=w1462:string, element #3=w1461:string)  [unwired: 3 in, 1 out]
                n507 = Index Array(array=w1457) -> (element=w1460:string)  [unwired: 1 in]
                n508 = Bundle("date/time string"=w1456, "SHIFT"=w1455, "Input 2"=w1460, "Input 2"=w1462, "Input 2"=w1461) -> (w1459:T28)  [unwired: 1 in]
                n509 = To Variant(anything=w1459) -> (Variant=w1465:variant)
                n510 = call <vilib>:"DB Tools Insert Data.vi"("data"=w1465, "error in (no error)"=w1468, "columns"=string[] ["DATE", "SHIFT", "ST8_DISPENSING", "ST8_LOAD", "ST8_FINAL_RST"], "table"="ST8_REPORT", "connection reference"=w1469) -> ("error out"=w1466:errorcluster, "connection reference out"=w1467:T13)  [unwired: 5 in]
              }
            }
            n511 = Bundle By Name(cluster=w1409, "OP - 80.Load"=w1403) -> (w1408:T11)
            n512 = call <vilib>:"Simple Error Handler.vi"("type of dialog (OK msg:1)"=w1417, "error in (no error)"=w1418) -> ("error out"=w1416:errorcluster)  [unwired: 3 in, 4 out]
            n513 = call <vilib>:"Clear Errors.vi"("error in (no error)"=w1416) -> ("error out"=w1414:errorcluster)  [unwired: 5 in, 1 out]
            n514 = property on="OP - 80" class="Clust"(error in=w1414) -> (error out=w1411:errorcluster, "Controls[]"=w1413:refnum<vi>[])  [unwired: 1 in, 1 out]
            n515 = for {
              tunnel: w1397 -> [w1428] mode=indexing
              tunnel: [w1427] -> w1396 mode=indexing if=w1425
              i -> [w1426]
              n516 = case shown="\"NG\"" w1428 {
                tunnel: [2 ("CYCLE STATUS OK, NOK, ABORTED") 1 ("CYCLE STATUS OK, NOK, ABORTED") 0 ("CYCLE STATUS OK, NOK, ABORTED")] -> w1427
                frame "NG" {
                }
                frame "OK" {
                }
                frame "-1", Default {
                }
              }
              n517 = Not Equal To 0?(x=w1426) -> (x != 0?=w1425:bool)
            }
            n518 = Index Array(array=w1413, index #1=3 ("index"), index #2=2 ("index")) -> (element #1=w1399:refnum<vi>, element #2=w1394:refnum<vi>)
            n519 = Build Array(w1399, w1394) -> (w1398:refnum<vi>[])
            n520 = for {
              tunnel: w1398 -> [w1437] mode=indexing
              shift-right: [w1433] -> w1410
              shift-left: w1411 -> [w1435]
              tunnel: w1396 -> [w1432] mode=indexing
              w1436 = refnum<vi> refnum  # Boolean
              n521 = To More Specific Class(target class=w1436, reference=w1437, error in=w1435) -> (specific class reference=w1438:refnum<vi>, error out=w1434:errorcluster)
              n522 = call "PADMINI_BOOL_COLOR_CHANGE.vi"("error in (no error)"=w1434, "Numeric"=w1432, "Boolean in"=w1438) -> ("error out"=w1433:errorcluster)  [unwired: 8 in]
            }
          }
          frame "SCAN9" {
            # "STATION OP 90"
            n523 = case shown="True" w1478 {
              tunnel: w1482 -> [w1506 w1540]
              tunnel: w1481 -> [w1498 w1539]
              tunnel: w1480 -> [_ _]
              tunnel: [w1501 w1538] -> w1477
              tunnel: [w1499 w1540] -> w1479
              tunnel: [w1483 "" ("trimmed string")] -> w1470
              frame False {
                n524 = call "PADMINI_AUTO_BARCODE_STRING 90.vi"("Enum"=enum16{"Read", "Write"}."Read", "error in (no error)"=w1498) -> ("error out"=w1497:errorcluster, "Input 2"=w1485:string[])  [unwired: 8 in]
                n525 = global read "Global 1.vi" "BARCODE RECIPE"() -> (w1486:string)
                n526 = Index Array(array=w1485) -> (element=w1484:string)  [unwired: 1 in]
                n527 = call <vilib>:"Trim Whitespace.vi"("string"=w1484) -> ("trimmed string"=w1483:string)  [unwired: 1 in]
                n528 = Match Pattern(string=w1483, regular expression=w1486) -> (match substring=w1487:string)  [unwired: 1 in, 3 out]
                n529 = String Length(string=w1486) -> (length=w1489:i32)
                n530 = String Length(string=w1487) -> (length=w1488:i32)
                n531 = Format Into String(format string="WHERE BARCODE  ='%s'", w1483) -> (resulting string=w1493:string)  [unwired: 2 in, 1 out]
                n532 = Equal?(x=w1489, y=w1488) -> (x = y?=w1490:bool)
                n533 = call <vilib>:"DB Tools Select Data.vi"("condition"=w1493, "error in (no error)"=w1497, "columns"=string[] ["BARCODE", "ST8_FINAL_RST", "ST9_FINAL_RST"], "table"="REPORT", "connection reference"=w1506) -> ("error out"=w1504:errorcluster, "data"=w1503:variant[][], "connection reference out"=w1499:T13)  [unwired: 1 in]
                n534 = call "PADMINI_varient_to_data.vi"("error in (no error)"=w1504, "data"=w1503) -> ("error out"=w1502:errorcluster, "Array"=w1500:string[][])  [unwired: 8 in]
                n535 = Equal?(x=w1483, y="") -> (x = y?=w1491:bool)
                n536 = case shown="True" w1491 {
                  tunnel: w1502 -> [w1510 w1534]
                  tunnel: [w1509 w1533] -> w1501
                  tunnel: w1500 -> [w1508 _]
                  tunnel: w1490 -> [w1507 _]
                  frame False {
                    n537 = case shown="True" w1507 {
                      tunnel: w1510 -> [w1514 w1518]
                      tunnel: [w1513 w1517] -> w1509
                      tunnel: w1508 -> [_ w1530]
                      frame False {
                        n538 = call "PADMINI_AUTO_BARCODE_STATUS 90.vi"("Enum"=enum16{"Read", "Write"}."Write", "error in (no error)"=w1514, "I/P"=bool[] [FALSE, TRUE, FALSE, FALSE, FALSE]) -> ("error out"=w1513:errorcluster)  [unwired: 7 in, 1 out]
                      }
                      frame True {
                        n539 = Index Array(array=w1530, index (row) #1=0 ("index (row)"), index (col) #1=1 ("disabled index (col)"), index (row) #2=0 ("index (row)"), index (col) #2=2 ("disabled index (col)")) -> (element #1=w1524:string)  [unwired: 1 out]
                        n540 = Empty String/Path?(string/path=w1524) -> (empty?=w1522:bool)
                        n541 = Equal?(x=w1524, y="OK") -> (x = y?=w1520:bool)
                        n542 = Not(x=w1520) -> (.not. x?=w1519:bool)
                        n543 = Build Array(TRUE ("element"), FALSE ("element"), w1522, w1520, w1519) -> (w1516:bool[])
                        n544 = call "PADMINI_AUTO_BARCODE_STATUS 90.vi"("Enum"=enum16{"Read", "Write"}."Write", "error in (no error)"=w1518, "I/P"=w1516) -> ("error out"=w1517:errorcluster)  [unwired: 7 in, 1 out]
                      }
                    }
                  }
                  frame True {
                    n545 = call "PADMINI_AUTO_BARCODE_STATUS 90.vi"("Enum"=enum16{"Read", "Write"}."Write", "error in (no error)"=w1534, "I/P"=bool[] [FALSE, FALSE, FALSE, FALSE, FALSE]) -> ("error out"=w1533:errorcluster)  [unwired: 7 in, 1 out]
                  }
                }
              }
              frame True {
                n546 = call "PADMINI_AUTO_BARCODE_STATUS 90.vi"("Enum"=enum16{"Read", "Write"}."Write", "error in (no error)"=w1539, "I/P"=bool[] [FALSE, FALSE, FALSE, FALSE, FALSE]) -> ("error out"=w1538:errorcluster)  [unwired: 7 in, 1 out]
              }
            }
            n547 = flat-sequence {
              tunnel: [w1542] -> w1476
              tunnel: w1477 -> [w1542]
              frame #0 {
                # "UPDATE op 90 SCAN sTATUS"
                n548 = global write "DATA LOG.vi" "OP 90 Outputs"(TRUE) -> ()
              }
            }
            n549 = Bundle By Name(cluster=w1472, "OP - 90.BARCODE"=w1470) -> (w1471:T11)
          }
          frame "DATALOG9" {
            w1567 = T14 2 items=["no dialog", "OK message", "continue or stop message", "OK message + warnings", "continue/stop + warnings"] ("type of dialog (OK msg:1)")
            # "datalog of OP 90"
            n550 = call "PADMINI_AUTO_BARCODE_STRING 90.vi"("Enum"=enum16{"Read", "Write"}."Read", "error in (no error)"=w1554) -> ("error out"=w1556:errorcluster, "Input 2"=w1548:string[])  [unwired: 8 in]
            n551 = call "PADMINI_AUTO_CYCLE VALUE 90.vi"("Enum"=enum16{"Read", "Write"}."Read", "error in (no error)"=w1554) -> ("Input 2"=w1544:dbl[])  [unwired: 8 in, 1 out]
            n552 = Index Array(array=w1544) -> (element #1=w1553:dbl, element #2=w1543:dbl)  [unwired: 2 in]
            n553 = Number To Fractional String(number=w1544, precision (6)=i16 2) -> (F-format string=w1551:string[])  [unwired: 2 in]
            n554 = case shown="True" w1572 {
              tunnel: w1573 -> [w1602 w1621]
              tunnel: w1556 -> [w1603 w1620]
              tunnel: [w1605 w1619] -> w1570
              tunnel: [w1604 w1618] -> w1568
              tunnel: w1571 -> [w1601 _]
              tunnel: w1551 -> [w1597 w1610]
              tunnel: w1548 -> [w1593 w1609]
              frame False {
                # "DO TRACEBILITY"
                n555 = Index Array(array=w1593) -> (element #1=w1594:string, element #2=w1591:string, element #3=w1589:string)  [unwired: 3 in]
                n556 = call <vilib>:"Trim Whitespace.vi"("string"=w1594) -> ("trimmed string"=w1595:string)  [unwired: 1 in]
                n557 = Index Array(array=w1597) -> (element #1=w1592:string, element #2=w1590:string)  [unwired: 2 in]
                n558 = Bundle("Input 2"=w1592, "Input 2"=w1591, "Input 2"=w1590, "Input 2"=w1589) -> (w1596:T19)  [unwired: 1 in]
                n559 = Format Into String(format string="Where BARCODE='%s' ", w1595) -> (resulting string=w1599:string)  [unwired: 2 in, 1 out]
                n560 = call <vilib>:"DB Tools Update Data.vi"("condition"=w1599, "data"=w1596, "error in (no error)"=w1603, "columns"=string[] ["ST9_SEAT_LT_DATA", "ST9_SEAT_STATUS", "ST9_STEAM_LT_DATA", "ST9_FINAL_RST"], "table"=w1601, "connection reference"=w1602) -> ("error out"=w1604:errorcluster, "connection reference out"=w1605:T13)  [unwired: 4 in]
              }
              frame True {
                # "TRAC BYPASS"
                n561 = local read "SHIFT"() -> (w1606:string)
                n562 = call "PADMINI_SHIFT_DATE.vi"("SHIFT"=w1606) -> ("date/time string"=w1607:string)  [unwired: 10 in]
                n563 = Index Array(array=w1609) -> (element #2=w1614:string, element #3=w1612:string)  [unwired: 3 in, 1 out]
                n564 = Index Array(array=w1610) -> (element #1=w1615:string, element #2=w1613:string)  [unwired: 2 in]
                n565 = Bundle("date/time string"=w1607, "SHIFT"=w1606, "Input 2"=w1615, "Input 2"=w1614, "Input 2"=w1613, "Input 2"=w1612) -> (w1611:T20)  [unwired: 1 in]
                n566 = To Variant(anything=w1611) -> (Variant=w1617:variant)
                n567 = call <vilib>:"DB Tools Insert Data.vi"("data"=w1617, "error in (no error)"=w1620, "columns"=string[] ["DATE", "SHIFT", "ST9_SEAT_LT_DATA", "ST9_SEAT_STATUS", "ST9_STEAM_LT_DATA", "ST9_FINAL_RST"], "table"="ST9_REPORT", "connection reference"=w1621) -> ("error out"=w1618:errorcluster, "connection reference out"=w1619:T13)  [unwired: 5 in]
              }
            }
            n568 = Bundle By Name(cluster=w1559, "OP - 90.Seat LT Data"=w1553, "OP - 90.Steam LT Data"=w1543) -> (w1558:T11)
            n569 = call <vilib>:"Simple Error Handler.vi"("type of dialog (OK msg:1)"=w1567, "error in (no error)"=w1568) -> ("error out"=w1566:errorcluster)  [unwired: 3 in, 4 out]
            n570 = call <vilib>:"Clear Errors.vi"("error in (no error)"=w1566) -> ("error out"=w1564:errorcluster)  [unwired: 5 in, 1 out]
            n571 = property on="OP - 90" class="Clust"(error in=w1564) -> (error out=w1561:errorcluster, "Controls[]"=w1563:refnum<vi>[])  [unwired: 1 in, 1 out]
            n572 = for {
              tunnel: w1548 -> [w1578] mode=indexing
              tunnel: [w1577] -> w1547 mode=indexing if=w1575
              i -> [w1576]
              n573 = case shown="\"NG\"" w1578 {
                tunnel: [2 ("CYCLE STATUS OK, NOK, ABORTED") 1 ("CYCLE STATUS OK, NOK, ABORTED") 0 ("CYCLE STATUS OK, NOK, ABORTED")] -> w1577
                frame "NG" {
                }
                frame "OK" {
                }
                frame "-1", Default {
                }
              }
              n574 = Not Equal To 0?(x=w1576) -> (x != 0?=w1575:bool)
            }
            n575 = Index Array(array=w1563, index #1=2 ("index"), index #2=4 ("index")) -> (element #1=w1550:refnum<vi>, element #2=w1545:refnum<vi>)
            n576 = Build Array(w1550, w1545) -> (w1549:refnum<vi>[])
            n577 = for {
              tunnel: w1549 -> [w1587] mode=indexing
              shift-right: [w1583] -> w1560
              shift-left: w1561 -> [w1585]
              tunnel: w1547 -> [w1582] mode=indexing
              w1586 = refnum<vi> refnum  # Boolean
              n578 = To More Specific Class(target class=w1586, reference=w1587, error in=w1585) -> (specific class reference=w1588:refnum<vi>, error out=w1584:errorcluster)
              n579 = call "PADMINI_BOOL_COLOR_CHANGE.vi"("error in (no error)"=w1584, "Numeric"=w1582, "Boolean in"=w1588) -> ("error out"=w1583:errorcluster)  [unwired: 8 in]
            }
          }
          frame "SCAN10" {
            # "STATION OP 10"
            n580 = case shown="False" w1630 {
              tunnel: w1634 -> [w1658 w1692]
              tunnel: w1633 -> [w1650 w1691]
              tunnel: w1632 -> [_ _]
              tunnel: [w1653 w1690] -> w1629
              tunnel: [w1651 w1692] -> w1631
              tunnel: [w1635 "" ("trimmed string")] -> w1622
              frame False {
                n581 = call "PADMINI_AUTO_BARCODE_STRING 100.vi"("Enum"=enum16{"Read", "Write"}."Read", "error in (no error)"=w1650) -> ("error out"=w1649:errorcluster, "Input 2"=w1637:string[])  [unwired: 8 in]
                n582 = global read "Global 1.vi" "BARCODE RECIPE"() -> (w1638:string)
                n583 = Index Array(array=w1637) -> (element=w1636:string)  [unwired: 1 in]
                n584 = call <vilib>:"Trim Whitespace.vi"("string"=w1636) -> ("trimmed string"=w1635:string)  [unwired: 1 in]
                n585 = Match Pattern(string=w1635, regular expression=w1638) -> (match substring=w1639:string)  [unwired: 1 in, 3 out]
                n586 = String Length(string=w1638) -> (length=w1641:i32)
                n587 = String Length(string=w1639) -> (length=w1640:i32)
                n588 = Format Into String(format string="WHERE BARCODE  ='%s'", w1635) -> (resulting string=w1645:string)  [unwired: 2 in, 1 out]
                n589 = Equal?(x=w1641, y=w1640) -> (x = y?=w1642:bool)
                n590 = call <vilib>:"DB Tools Select Data.vi"("condition"=w1645, "error in (no error)"=w1649, "columns"=string[] ["BARCODE", "ST9_FINAL_RST", "ST10_FINAL_RST"], "table"="REPORT", "connection reference"=w1658) -> ("error out"=w1656:errorcluster, "data"=w1655:variant[][], "connection reference out"=w1651:T13)  [unwired: 1 in]
                n591 = call "PADMINI_varient_to_data.vi"("error in (no error)"=w1656, "data"=w1655) -> ("error out"=w1654:errorcluster, "Array"=w1652:string[][])  [unwired: 8 in]
                n592 = Equal?(x=w1635, y="") -> (x = y?=w1643:bool)
                n593 = case shown="False" w1643 {
                  tunnel: w1654 -> [w1662 w1686]
                  tunnel: [w1661 w1685] -> w1653
                  tunnel: w1652 -> [w1660 _]
                  tunnel: w1642 -> [w1659 _]
                  frame False {
                    n594 = case shown="False" w1659 {
                      tunnel: w1662 -> [w1666 w1670]
                      tunnel: [w1665 w1669] -> w1661
                      tunnel: w1660 -> [_ w1682]
                      frame False {
                        n595 = call "PADMINI_AUTO_BARCODE_STATUS 90.vi"("Enum"=enum16{"Read", "Write"}."Write", "error in (no error)"=w1666, "I/P"=bool[] [FALSE, TRUE, FALSE, FALSE, FALSE]) -> ("error out"=w1665:errorcluster)  [unwired: 7 in, 1 out]
                      }
                      frame True {
                        n596 = Index Array(array=w1682, index (row) #1=0 ("index (row)"), index (col) #1=1 ("disabled index (col)"), index (row) #2=0 ("index (row)"), index (col) #2=2 ("disabled index (col)")) -> (element #1=w1676:string)  [unwired: 1 out]
                        n597 = Empty String/Path?(string/path=w1676) -> (empty?=w1674:bool)
                        n598 = Equal?(x=w1676, y="OK") -> (x = y?=w1672:bool)
                        n599 = Not(x=w1672) -> (.not. x?=w1671:bool)
                        n600 = Build Array(TRUE ("element"), FALSE ("element"), w1674, w1672, w1671) -> (w1668:bool[])
                        n601 = call "PADMINI_AUTO_BARCODE_STATUS 100.vi"("Enum"=enum16{"Read", "Write"}."Write", "error in (no error)"=w1670, "I/P"=w1668) -> ("error out"=w1669:errorcluster)  [unwired: 7 in, 1 out]
                      }
                    }
                  }
                  frame True {
                    n602 = call "PADMINI_AUTO_BARCODE_STATUS 100.vi"("Enum"=enum16{"Read", "Write"}."Write", "error in (no error)"=w1686, "I/P"=bool[] [FALSE, FALSE, FALSE, FALSE, FALSE]) -> ("error out"=w1685:errorcluster)  [unwired: 7 in, 1 out]
                  }
                }
              }
              frame True {
                n603 = call "PADMINI_AUTO_BARCODE_STATUS 100.vi"("Enum"=enum16{"Read", "Write"}."Write", "error in (no error)"=w1691, "I/P"=bool[] [FALSE, FALSE, FALSE, FALSE, FALSE]) -> ("error out"=w1690:errorcluster)  [unwired: 7 in, 1 out]
              }
            }
            n604 = flat-sequence {
              tunnel: [w1694] -> w1628
              tunnel: w1629 -> [w1694]
              frame #0 {
                # "UPDATE op 100 SCAN sTATUS"
                n605 = global write "DATA LOG.vi" "OP 100 Outputs"(TRUE) -> ()
              }
            }
            n606 = Bundle By Name(cluster=w1624, "OP - 100.BARCODE"=w1622) -> (w1623:T11)
          }
          frame "SCAN11" {
            # "STATION OP 110"
            n607 = case shown="False" w1701 {
              tunnel: w1705 -> [w1729 w1762]
              tunnel: w1704 -> [w1721 w1761]
              tunnel: w1703 -> [_ _]
              tunnel: [w1724 w1760] -> w1700
              tunnel: [w1722 w1762] -> w1702
              frame False {
                n608 = call "PADMINI_AUTO_BARCODE_STRING 100.vi"("Enum"=enum16{"Read", "Write"}."Read", "error in (no error)"=w1721) -> ("error out"=w1720:errorcluster, "Input 2"=w1707:string[])  [unwired: 8 in]
                n609 = global read "Global 1.vi" "BARCODE RECIPE"() -> (w1708:string)
                n610 = Index Array(array=w1707) -> (element=w1706:string)  [unwired: 1 in]
                n611 = call <vilib>:"Trim Whitespace.vi"("string"=w1706) -> ("trimmed string"=w1712:string)  [unwired: 1 in]
                n612 = Match Pattern(string=w1712, regular expression=w1708) -> (match substring=w1709:string)  [unwired: 1 in, 3 out]
                n613 = String Length(string=w1708) -> (length=w1711:i32)
                n614 = String Length(string=w1709) -> (length=w1710:i32)
                n615 = Format Into String(format string="WHERE BARCODE  ='%s'", w1712) -> (resulting string=w1716:string)  [unwired: 2 in, 1 out]
                n616 = Equal?(x=w1711, y=w1710) -> (x = y?=w1713:bool)
                n617 = call <vilib>:"DB Tools Select Data.vi"("condition"=w1716, "error in (no error)"=w1720, "columns"=string[] ["BARCODE", "ST9_FINAL_RST", "ST10_FINAL_RST"], "table"="REPORT", "connection reference"=w1729) -> ("error out"=w1727:errorcluster, "data"=w1726:variant[][], "connection reference out"=w1722:T13)  [unwired: 1 in]
                n618 = call "PADMINI_varient_to_data.vi"("error in (no error)"=w1727, "data"=w1726) -> ("error out"=w1725:errorcluster, "Array"=w1723:string[][])  [unwired: 8 in]
                n619 = Equal?(x=w1712, y="") -> (x = y?=w1714:bool)
                n620 = case shown="True" w1714 {
                  tunnel: w1725 -> [w1733 w1757]
                  tunnel: [w1732 w1756] -> w1724
                  tunnel: w1723 -> [w1731 _]
                  tunnel: w1713 -> [w1730 _]
                  frame False {
                    n621 = case shown="True" w1730 {
                      tunnel: w1733 -> [w1737 w1741]
                      tunnel: [w1736 w1740] -> w1732
                      tunnel: w1731 -> [_ w1753]
                      frame False {
                        n622 = call "PADMINI_AUTO_BARCODE_STATUS 90.vi"("Enum"=enum16{"Read", "Write"}."Write", "error in (no error)"=w1737, "I/P"=bool[] [FALSE, TRUE, FALSE, FALSE, FALSE]) -> ("error out"=w1736:errorcluster)  [unwired: 7 in, 1 out]
                      }
                      frame True {
                        n623 = Index Array(array=w1753, index (row) #1=0 ("index (row)"), index (col) #1=1 ("disabled index (col)"), index (row) #2=0 ("index (row)"), index (col) #2=2 ("disabled index (col)")) -> (element #1=w1747:string)  [unwired: 1 out]
                        n624 = Empty String/Path?(string/path=w1747) -> (empty?=w1745:bool)
                        n625 = Equal?(x=w1747, y="OK") -> (x = y?=w1743:bool)
                        n626 = Not(x=w1743) -> (.not. x?=w1742:bool)
                        n627 = Build Array(TRUE ("element"), FALSE ("element"), w1745, w1743, w1742) -> (w1739:bool[])
                        n628 = call "PADMINI_AUTO_BARCODE_STATUS 100.vi"("Enum"=enum16{"Read", "Write"}."Write", "error in (no error)"=w1741, "I/P"=w1739) -> ("error out"=w1740:errorcluster)  [unwired: 7 in, 1 out]
                      }
                    }
                  }
                  frame True {
                    n629 = call "PADMINI_AUTO_BARCODE_STATUS 100.vi"("Enum"=enum16{"Read", "Write"}."Write", "error in (no error)"=w1757, "I/P"=bool[] [FALSE, FALSE, FALSE, FALSE, FALSE]) -> ("error out"=w1756:errorcluster)  [unwired: 7 in, 1 out]
                  }
                }
              }
              frame True {
                n630 = call "PADMINI_AUTO_BARCODE_STATUS 100.vi"("Enum"=enum16{"Read", "Write"}."Write", "error in (no error)"=w1761, "I/P"=bool[] [FALSE, FALSE, FALSE, FALSE, FALSE]) -> ("error out"=w1760:errorcluster)  [unwired: 7 in, 1 out]
              }
            }
            n631 = flat-sequence {
              tunnel: [w1764] -> w1699
              tunnel: w1700 -> [w1764]
              frame #0 {
                # "UPDATE op 100 SCAN sTATUS"
                n632 = global write "DATA LOG.vi" "OP 100 Outputs"(TRUE) -> ()
              }
            }
          }
          frame "DATALOG10" {
            w1765 = 0.0 ("OP - 100.Response Time FWD (mSec)")
            w1800 = T14 2 items=["no dialog", "OK message", "continue or stop message", "OK message + warnings", "continue/stop + warnings"] ("type of dialog (OK msg:1)")
            # "datalog of OP 100"
            n633 = call "PADMINI_AUTO_BARCODE_STRING 100.vi"("Enum"=enum16{"Read", "Write"}."Read", "error in (no error)"=w1771) -> ("error out"=w1789:errorcluster, "Input 2"=w1782:string[])  [unwired: 8 in]
            n634 = call "PADMINI_AUTO_CYCLE TIME 100.vi"("Enum"=enum16{"Read", "Write"}."Read", "error in (no error)"=w1771) -> ("Time of Day result array"=w1770:timestamp[])  [unwired: 8 in, 1 out]
            n635 = call "PADMINI_AUTO_CYCLE VALUE 100.vi"("Enum"=enum16{"Read", "Write"}."Read", "error in (no error)"=w1771) -> ("Input 2"=w1780:dbl[])  [unwired: 8 in, 1 out]
            n636 = Index Array(array=w1780) -> (element #1=w1787:dbl, element #2=w1779:dbl, element #3=w1778:dbl, element #4=w1777:dbl, element #5=w1776:dbl, element #6=w1775:dbl, element #7=w1774:dbl, element #8=w1773:dbl)  [unwired: 8 in]
            n637 = Index Array(array=w1770) -> (element #1=w1769:timestamp, element #2=w1768:timestamp)  [unwired: 2 in]
            n638 = Number To Fractional String(number=w1780, precision (6)=i16 2) -> (F-format string=w1785:string[])  [unwired: 2 in]
            n639 = Get Date/Time String(seconds (now)=w1769) -> (time string=w1767:string)  [unwired: 2 in, 1 out]
            n640 = Get Date/Time String(seconds (now)=w1768) -> (time string=w1766:string)  [unwired: 2 in, 1 out]
            n641 = case shown="True" w1805 {
              tunnel: w1806 -> [w1842 w1869]
              tunnel: w1789 -> [w1843 w1868]
              tunnel: [w1845 w1867] -> w1803
              tunnel: [w1844 w1866] -> w1801
              tunnel: w1804 -> [w1841 _]
              tunnel: w1785 -> [w1837 w1850]
              tunnel: w1782 -> [w1834 w1851]
              tunnel: w1767 -> [w1823 w1848]
              tunnel: w1766 -> [w1822 w1849]
              frame False {
                # "DO TRACEBILITY"
                n642 = Index Array(array=w1834) -> (element=w1826:string)  [unwired: 1 in]
                n643 = call <vilib>:"Trim Whitespace.vi"("string"=w1826) -> ("trimmed string"=w1835:string)  [unwired: 1 in]
                n644 = Index Array(array=w1837) -> (element #1=w1833:string, element #2=w1832:string, element #3=w1831:string, element #4=w1824:string, element #5=w1830:string, element #6=w1825:string, element #7=w1829:string, element #8=w1828:string, element #9=w1827:string)  [unwired: 9 in]
                n645 = Bundle("Input 2"=w1833, "Input 2"=w1832, "Input 2"=w1831, "time string"=w1823, "time string"=w1822, "Input 2"=w1824, "Input 2"=w1830, "Input 2"=w1825, "Input 2"=w1829, "Input 2"=w1828, "Input 2"=w1827, "Input 2"=w1826) -> (w1836:T29)  [unwired: 1 in]
                n646 = Format Into String(format string="Where BARCODE='%s' ", w1835) -> (resulting string=w1839:string)  [unwired: 2 in, 1 out]
                n647 = call <vilib>:"DB Tools Update Data.vi"("condition"=w1839, "data"=w1836, "error in (no error)"=w1843, "columns"=string[] ["ST10_SENSOR_OP_OPEN_V", "ST10_START_OF_CLOSE_SENSOR_V", "ST10_SENSOR_OP_FULL_CLOSE_V", "ST10_RESPONSE_TIME_FWD", "ST10_RESPONSE_TIME_REV", "ST10_MOTOR_V_START_OF_CLOSE_A", "ST10_MOTOR_V_FULL_CLOSE_B", "ST10_MOTOR_V_START_BACK_C", "ST10_MOTOR_V_FULL_OPEN_D", "ST10_MOTOR_RMS_CURRENT_A", "ST10_FINAL_RST"], "table"=w1841, "connection reference"=w1842) -> ("error out"=w1844:errorcluster, "connection reference out"=w1845:T13)  [unwired: 4 in]
              }
              frame True {
                # "TRAC BYPASS"
                n648 = local read "SHIFT"() -> (w1846:string)
                n649 = Index Array(array=w1851) -> (element=w1855:string)  [unwired: 1 in]
                n650 = call "PADMINI_SHIFT_DATE.vi"("SHIFT"=w1846) -> ("date/time string"=w1847:string)  [unwired: 10 in]
                n651 = Index Array(array=w1850) -> (element #1=w1862:string, element #2=w1861:string, element #3=w1860:string, element #4=w1853:string, element #5=w1859:string, element #6=w1854:string, element #7=w1858:string, element #8=w1857:string, element #9=w1856:string)  [unwired: 9 in]
                n652 = Bundle("date/time string"=w1847, "SHIFT"=w1846, "Input 2"=w1862, "Input 2"=w1861, "Input 2"=w1860, "time string"=w1848, "time string"=w1849, "Input 2"=w1853, "Input 2"=w1859, "Input 2"=w1854, "Input 2"=w1858, "Input 2"=w1857, "Input 2"=w1856, "Input 2"=w1855) -> (w1852:T30)  [unwired: 1 in]
                n653 = To Variant(anything=w1852) -> (Variant=w1865:variant)
                n654 = call <vilib>:"DB Tools Insert Data.vi"("data"=w1865, "error in (no error)"=w1868, "columns"=string[] ["DATE", "SHIFT", "ST10_SENSOR_OP_OPEN_V", "ST10_START_OF_CLOSE_SENSOR_V", "ST10_SENSOR_OP_FULL_CLOSE_V", "ST10_RESPONSE_TIME_FWD", "ST10_RESPONSE_TIME_REV", "ST10_MOTOR_V_START_OF_CLOSE_A", "ST10_MOTOR_V_FULL_CLOSE_B", "ST10_MOTOR_V_START_BACK_C", "ST10_MOTOR_V_FULL_OPEN_D", "ST10_MOTOR_RMS_CURRENT_A", "ST10_FINAL_RST"], "table"="ST10_REPORT", "connection reference"=w1869) -> ("error out"=w1866:errorcluster, "connection reference out"=w1867:T13)  [unwired: 5 in]
              }
            }
            n655 = Bundle By Name(cluster=w1792, "OP - 100.Sensor O/P Open V"=w1787, "OP - 100.Start Of Close Sensor V"=w1779, "OP - 100.Sensor O/P Full Close V"=w1778, "OP - 100.Response Time FWD (mSec)"=w1765, "OP - 100.Response Time REV (mSec)"=w1765, "OP - 100.Motor V Start Of Close A"=w1777, "OP - 100.Motor V Full Close B R"=w1776, "OP - 100.Motor V Start Back C"=w1775, "OP - 100.Motor V Full Open D"=w1774, "OP - 100.Motor RMS Current A"=w1773) -> (w1791:T11)
            n656 = call <vilib>:"Simple Error Handler.vi"("type of dialog (OK msg:1)"=w1800, "error in (no error)"=w1801) -> ("error out"=w1799:errorcluster)  [unwired: 3 in, 4 out]
            n657 = call <vilib>:"Clear Errors.vi"("error in (no error)"=w1799) -> ("error out"=w1797:errorcluster)  [unwired: 5 in, 1 out]
            n658 = property on="OP - 100" class="Clust"(error in=w1797) -> (error out=w1794:errorcluster, "Controls[]"=w1796:refnum<vi>[])  [unwired: 1 in, 1 out]
            n659 = for {
              tunnel: w1782 -> [w1811] mode=indexing
              tunnel: [w1810] -> w1781 mode=indexing if=w1808
              i -> [w1809]
              n660 = case shown="\"NG\"" w1811 {
                tunnel: [2 ("CYCLE STATUS OK, NOK, ABORTED") 1 ("CYCLE STATUS OK, NOK, ABORTED") 0 ("CYCLE STATUS OK, NOK, ABORTED")] -> w1810
                frame "NG" {
                }
                frame "OK" {
                }
                frame "-1", Default {
                }
              }
              n661 = Not Equal To 0?(x=w1809) -> (x != 0?=w1808:bool)
            }
            n662 = Index Array(array=w1796, index=3) -> (element=w1784:refnum<vi>)
            n663 = Build Array(w1784) -> (w1783:refnum<vi>[])
            n664 = for {
              tunnel: w1783 -> [w1820] mode=indexing
              shift-right: [w1816] -> w1793
              shift-left: w1794 -> [w1818]
              tunnel: w1781 -> [w1815] mode=indexing
              w1819 = refnum<vi> refnum  # Boolean
              n665 = To More Specific Class(target class=w1819, reference=w1820, error in=w1818) -> (specific class reference=w1821:refnum<vi>, error out=w1817:errorcluster)
              n666 = call "PADMINI_BOOL_COLOR_CHANGE.vi"("error in (no error)"=w1817, "Numeric"=w1815, "Boolean in"=w1821) -> ("error out"=w1816:errorcluster)  [unwired: 8 in]
            }
          }
          frame "EMERGENCY STOP" {
          }
          frame "STOP" {
            n667 = global read "Global 1.vi" "BARCODE RECIPE"() -> (w1880:string)
            n668 = Bundle("BARCODE RECIPE"=w1880) -> (w1879:cluster{"BARCODE RECIPE":string})  [unwired: 1 in]
            n669 = call <vilib>:"DB Tools Update Data.vi"("data"=w1879, "error in (no error)"=w1885, "columns"=string[] ["PREVIOUS_LOADED_RECIPE"], "table"="BARCODE_RECIPE", "connection reference"=w1883) -> ("error out"=w1884:errorcluster, "connection reference out"=w1882:T13)  [unwired: 5 in]
          }
        }
      }
      frame Error {
        # "Return true in any case that should stop the loop."
      }
    }
    n670 = Unbundle By Name(w123) -> ("OP - 90"=→"OP - 90":T8, "OP - 100"=→"OP - 100":T9, "OP - 110"=→"OP - 110":cluster{"BARCODE":string})
    n671 = Unbundle By Name(w123) -> ("OP - 10"=→"OP - 10":T4, "OP - 20"=→"OP - 20":T31, "OP - 30"=→"OP - 30":T3, "OP - 40"=→"OP - 40":T2)
    n672 = Unbundle By Name(w123) -> ("OP - 50"=→"OP - 50":T1, "OP - 60"=→"OP - 60":T10, "OP - 70"=→"OP - 70":T7, "OP - 80"=→"OP - 80":T6)
    n673 = Wait (ms)(milliseconds to wait=u32 100) -> ()  [unwired: 1 out]
  }
  n674 = while {
    shift-right: [w1909] -> w71
    shift-left: w20 -> [w1903]
    shift-right: [w1910] -> w65
    shift-left: w69 -> [w1918]
    stop <- w1908 stop-if-true
    n675 = local read "Shift_change"() -> (w1916:bool)
    n676 = call <vilib>:"Clear Errors.vi"("error in (no error)"=w1903) -> ("error out"=w1894:errorcluster)  [unwired: 5 in, 1 out]
    n677 = call "READ EMERGENCY BIT.vi"("Enum"=enum16{"Read", "Write"}."Read", "error in (no error)"=w1894) -> ("Array Out"=w1906:dbl[])  [unwired: 8 in, 1 out]
    n678 = case shown="True" w1916 {
      tunnel: w1894 -> [w1935 w1948]
      tunnel: [w1936 w1947] -> w1915
      frame False {
        n679 = local read "SHIFT_DATA 2"() -> (w1938:string[])
        n680 = Get Date/Time In Seconds() -> (seconds since 1Jan1904=w1937:timestamp)
        n681 = call "String To Time_4.vi"("error in (no error)"=w1935, "String Array In"=w1938) -> ("error out"=w1934:errorcluster, "Time Stamp Out"=w1933:timestamp[])  [unwired: 8 in]
        "Time Stamp Out 4" <- w1933
        n682 = call "Shift Calculation_4.vi"("error in (no error)"=w1934, "Current Time"=w1937, "Time Stamp Out"=w1933) -> ("error out"=w1932:errorcluster, "Shift"=w1931:i32)  [unwired: 7 in]
        n683 = call <vilib>:"Clear Errors.vi"("error in (no error)"=w1932) -> ()  [unwired: 5 in, 2 out]
        n684 = case shown="4" w1931 {
          tunnel: ["A" "B" "C" "D"] -> w1936
          frame 1, Default {
          }
          frame 2 {
          }
          frame 3 {
          }
          frame 4 {
          }
        }
      }
      frame True {
        n685 = local read "SHIFT_DATA"() -> (w1946:string[])
        n686 = Get Date/Time In Seconds() -> (seconds since 1Jan1904=w1949:timestamp)
        n687 = call "String To Time.vi"("error in (no error)"=w1948, "String Array In"=w1946) -> ("error out"=w1945:errorcluster, "Time Stamp Out"=w1950:timestamp[])  [unwired: 8 in]
        "Time Stamp Out" <- w1950
        n688 = call "Shift Calculation.vi"("error in (no error)"=w1945, "Current Time"=w1949, "Time Stamp Out"=w1950) -> ("error out"=w1944:errorcluster, "Shift"=w1943:i32)  [unwired: 7 in]
        "Shift 4" <- w1943
        n689 = call <vilib>:"Clear Errors.vi"("error in (no error)"=w1944) -> ()  [unwired: 5 in, 2 out]
        n690 = case shown="3" w1943 {
          tunnel: ["A" "B" "C"] -> w1947
          frame 1, Default {
          }
          frame 2 {
          }
          frame 3 {
          }
        }
      }
    }
    "SHIFT" <- w1915
    n691 = Index Array(array=w1906) -> (element=w1905:dbl)  [unwired: 1 in]
    n692 = call "VALUE_CHANGE - ST1_RESULT.vi"("Numeric"=w1905) -> ("Boolean"=w1904:bool)  [unwired: 9 in, 1 out]
    n693 = global write "Global 1.vi" "EMERGENCY STOP"(w1904) -> ()
    n694 = call "Trigger_Loggic.vi"("error in (no error)"=w1894) -> ("error out"=w1899:errorcluster, "Array"=w1919:i32[])  [unwired: 9 in]
    n695 = for {
      tunnel: w1919 -> [w1954] mode=indexing
      shift-right: [w1958] -> w1912
      shift-left: w1918 -> [w1957]
      shift-right: [w1956] -> w1911
      shift-left: w1899 -> [w1955]
      n696 = case shown="19" w1954 {
        tunnel: [w1961 w1966 w1971 w1976 w1981 w1986 w1991 w1996 w2001 w2006 w2011 w2016 w2021 w2026 w2031 w2036 w2041 w2046 w2051 w2056 w2061 w2066 w2071] -> w1958
        tunnel: w1957 -> [w1963 w1968 w1973 w1978 w1983 w1988 w1993 w1998 w2003 w2008 w2013 w2018 w2023 w2028 w2033 w2038 w2043 w2048 w2053 w2058 w2063 w2068 w2073]
        tunnel: [w1960 w1965 w1970 w1975 w1980 w1985 w1990 w1995 w2000 w2005 w2010 w2015 w2020 w2025 w2030 w2035 w2040 w2045 w2050 w2055 w2060 w2065 w2070] -> w1956
        tunnel: w1955 -> [w1962 w1967 w1972 w1977 w1982 w1987 w1992 w1997 w2002 w2007 w2012 w2017 w2022 w2027 w2032 w2037 w2042 w2047 w2052 w2057 w2062 w2067 w2072]
        frame -1, Default {
          # "DEFAULT"
          n697 = Enqueue Element(queue=w1963, element=cluster{"CASE 2":T12} {"CASE 2"=enum."-1"}, error in (no error)=w1962) -> (queue out=w1961:refnum<queue>, error out=w1960:errorcluster)  [unwired: 1 in, 1 out]
        }
        frame 0 {
          # "SCAN BARCODE OP 10"
          n698 = Enqueue Element(queue=w1968, element=cluster{"CASE 2":T12} {"CASE 2"=enum."SCAN1"}, error in (no error)=w1967) -> (queue out=w1966:refnum<queue>, error out=w1965:errorcluster)  [unwired: 1 in, 1 out]
        }
        frame 1 {
          # "DATALOG OF OP 10"
          n699 = Enqueue Element(queue=w1973, element=cluster{"CASE 2":T12} {"CASE 2"=enum."DATALOG1"}, error in (no error)=w1972) -> (queue out=w1971:refnum<queue>, error out=w1970:errorcluster)  [unwired: 1 in, 1 out]
        }
        frame 2 {
          # "SCAN BARCODE OP 20"
          n700 = Enqueue Element(queue=w1978, element=cluster{"CASE 2":T12} {"CASE 2"=enum."SCAN2"}, error in (no error)=w1977) -> (queue out=w1976:refnum<queue>, error out=w1975:errorcluster)  [unwired: 1 in, 1 out]
        }
        frame 3 {
          # "DATALOG OF OP 20"
          n701 = Enqueue Element(queue=w1983, element=cluster{"CASE 2":T12} {"CASE 2"=enum."DATALOG2"}, error in (no error)=w1982) -> (queue out=w1981:refnum<queue>, error out=w1980:errorcluster)  [unwired: 1 in, 1 out]
        }
        frame 4 {
          # "SCAN BARCODE OP 30"
          n702 = Enqueue Element(queue=w1988, element=cluster{"CASE 2":T12} {"CASE 2"=enum."SCAN3"}, error in (no error)=w1987) -> (queue out=w1986:refnum<queue>, error out=w1985:errorcluster)  [unwired: 1 in, 1 out]
        }
        frame 5 {
          # "DATALOG OF OP 30"
          n703 = Enqueue Element(queue=w1993, element=cluster{"CASE 2":T12} {"CASE 2"=enum."DATALOG3"}, error in (no error)=w1992) -> (queue out=w1991:refnum<queue>, error out=w1990:errorcluster)  [unwired: 1 in, 1 out]
        }
        frame 6 {
          # "SCAN BARCODE OP 40"
          n704 = Enqueue Element(queue=w1998, element=cluster{"CASE 2":T12} {"CASE 2"=enum."SCAN4"}, error in (no error)=w1997) -> (queue out=w1996:refnum<queue>, error out=w1995:errorcluster)  [unwired: 1 in, 1 out]
        }
        frame 7 {
          # "DATALOG OF OP 40"
          n705 = Enqueue Element(queue=w2003, element=cluster{"CASE 2":T12} {"CASE 2"=enum."DATALOG4"}, error in (no error)=w2002) -> (queue out=w2001:refnum<queue>, error out=w2000:errorcluster)  [unwired: 1 in, 1 out]
        }
        frame 8 {
          # "SCAN BARCODE OP 50"
          n706 = Enqueue Element(queue=w2008, element=cluster{"CASE":T12} {"CASE"=enum."SCAN5"}, error in (no error)=w2007) -> (queue out=w2006:refnum<queue>, error out=w2005:errorcluster)  [unwired: 1 in, 1 out]
        }
        frame 9 {
          # "DATALOG OF OP 50"
          n707 = Enqueue Element(queue=w2013, element=cluster{"CASE":T12} {"CASE"=enum."DATALOG5"}, error in (no error)=w2012) -> (queue out=w2011:refnum<queue>, error out=w2010:errorcluster)  [unwired: 1 in, 1 out]
        }
        frame 10 {
          # "SCAN BARCODE OP 60"
          n708 = Enqueue Element(queue=w2018, element=cluster{"CASE 2":T12} {"CASE 2"=enum."SCAN6"}, error in (no error)=w2017) -> (queue out=w2016:refnum<queue>, error out=w2015:errorcluster)  [unwired: 1 in, 1 out]
        }
        frame 11 {
          # "DATALOG OF OP 60"
          n709 = Enqueue Element(queue=w2023, element=cluster{"CASE 2":T12} {"CASE 2"=enum."DATALOG6"}, error in (no error)=w2022) -> (queue out=w2021:refnum<queue>, error out=w2020:errorcluster)  [unwired: 1 in, 1 out]
        }
        frame 12 {
          # "SCAN BARCODE OP 70"
          n710 = Enqueue Element(queue=w2028, element=cluster{"CASE 2":T12} {"CASE 2"=enum."SCAN7"}, error in (no error)=w2027) -> (queue out=w2026:refnum<queue>, error out=w2025:errorcluster)  [unwired: 1 in, 1 out]
        }
        frame 13 {
          # "DATALOG OF OP 70"
          n711 = Enqueue Element(queue=w2033, element=cluster{"CASE 2":T12} {"CASE 2"=enum."DATALOG7"}, error in (no error)=w2032) -> (queue out=w2031:refnum<queue>, error out=w2030:errorcluster)  [unwired: 1 in, 1 out]
        }
        frame 14 {
          # "SCAN BARCODE 80"
          n712 = Enqueue Element(queue=w2038, element=cluster{"CASE 2":T12} {"CASE 2"=enum."SCAN8"}, error in (no error)=w2037) -> (queue out=w2036:refnum<queue>, error out=w2035:errorcluster)  [unwired: 1 in, 1 out]
        }
        frame 15 {
          # "DATALOG OF OP 80"
          n713 = Enqueue Element(queue=w2043, element=cluster{"CASE 2":T12} {"CASE 2"=enum."DATALOG8"}, error in (no error)=w2042) -> (queue out=w2041:refnum<queue>, error out=w2040:errorcluster)  [unwired: 1 in, 1 out]
        }
        frame 16 {
          # "SCAN BARCODE OP 90"
          n714 = Enqueue Element(queue=w2048, element=cluster{"CASE 2":T12} {"CASE 2"=enum."SCAN9"}, error in (no error)=w2047) -> (queue out=w2046:refnum<queue>, error out=w2045:errorcluster)  [unwired: 1 in, 1 out]
        }
        frame 17 {
          # "DATALOG OF OP 90"
          n715 = Enqueue Element(queue=w2053, element=cluster{"CASE 2":T12} {"CASE 2"=enum."DATALOG9"}, error in (no error)=w2052) -> (queue out=w2051:refnum<queue>, error out=w2050:errorcluster)  [unwired: 1 in, 1 out]
        }
        frame 18 {
          # "SCAN BARCODE OP 100"
          n716 = Enqueue Element(queue=w2058, element=cluster{"CASE 2":T12} {"CASE 2"=enum."SCAN10"}, error in (no error)=w2057) -> (queue out=w2056:refnum<queue>, error out=w2055:errorcluster)  [unwired: 1 in, 1 out]
        }
        frame 19 {
          # "DATALOG OF OP 100"
          n717 = Enqueue Element(queue=w2063, element=cluster{"CASE 2":T12} {"CASE 2"=enum."DATALOG10"}, error in (no error)=w2062) -> (queue out=w2061:refnum<queue>, error out=w2060:errorcluster)  [unwired: 1 in, 1 out]
        }
        frame 20 {
          # "SCAN BARCODE OP 110"
          n718 = Enqueue Element(queue=w2068, element=cluster{"CASE 2":T12} {"CASE 2"=enum."SCAN11"}, error in (no error)=w2067) -> (queue out=w2066:refnum<queue>, error out=w2065:errorcluster)  [unwired: 1 in, 1 out]
        }
        frame 21 {
          # "DATALOG OF OP 110"
          n719 = Enqueue Element(queue=w2073, element=cluster{"CASE 2":T12} {"CASE 2"=enum."DATALOG11"}, error in (no error)=w2072) -> (queue out=w2071:refnum<queue>, error out=w2070:errorcluster)  [unwired: 1 in, 1 out]
        }
      }
    }
    n720 = Wait (ms)(milliseconds to wait=u32 50) -> ()  [unwired: 1 out]
    n721 = global read "Global 1.vi" "PLC COMM"() -> (→"PLC COM.":bool)
    n722 = global read "Global 1.vi" "PLC 1"() -> (→"OP 10 & 20":bool)
    n723 = global read "Global 1.vi" "PLC 2"() -> (→"OP 30":bool)
    n724 = global read "Global 1.vi" "PLC 3"() -> (→"OP 40":bool)
    n725 = case shown="True" "stop 2" {
      tunnel: w1912 -> [w1922 w1928]
      tunnel: [w1922 w1927] -> w1910
      tunnel: w1911 -> [w1921 w1926]
      tunnel: [w1921 w1925] -> w1909
      tunnel: [FALSE TRUE] -> w1908
      frame False {
      }
      frame True {
        n726 = Flush Queue(queue=w1928, error in (no error)=w1926) -> (queue out=w1930:refnum<queue>, error out=w1929:errorcluster)  [unwired: 1 out]
        n727 = Enqueue Element(queue=w1930, element=cluster{"CASE 2":T12} {"CASE 2"=enum."STOP"}, error in (no error)=w1929) -> (queue out=w1927:refnum<queue>, error out=w1925:errorcluster)  [unwired: 1 in, 1 out]
      }
    }
    "stop" <- w1908
    n728 = global read "Global 1.vi" "PLC 4"() -> (→"OP 50":bool)
    n729 = global read "Global 1.vi" "PLC 5"() -> (→"OP 60":bool)
    n730 = global read "Global 1.vi" "PLC 7"() -> (→"OP 90 -100 - 110":bool)
    n731 = global read "Global 1.vi" "PLC 6"() -> (→"OP 70 & 80":bool)
  }
  n732 = Release Queue(queue=w65, error in (no error)=w71) -> (error out=w48:errorcluster)  [unwired: 1 in, 2 out]
  n733 = call <vilib>:"Clear Errors.vi"("error in (no error)"=w67) -> ("error out"=w52:errorcluster)  [unwired: 5 in, 1 out]
  n734 = call <vilib>:"DB Tools Close Connection.vi"("error in (no error)"=w52, "connection reference"=w66) -> ("error out"=w49:errorcluster)  [unwired: 5 in]
  n735 = Merge Errors(w48, w49) -> (w50:errorcluster)
  n736 = call <vilib>:"Simple Error Handler.vi"("error in (no error)"=w50) -> ("error out"=w45:errorcluster)  [unwired: 4 in, 4 out]
  n737 = call <vilib>:"Clear Errors.vi"("error in (no error)"=w45) -> ("error out"=w51:errorcluster)  [unwired: 5 in, 1 out]
  n738 = flat-sequence {
    tunnel: w51 -> [w2075]
    tunnel: [w2075] -> w53
    frame #0 {
      n739 = global write "Global 1.vi" "REMOVE VI"(TRUE ("remove_VI")) -> ()
    }
  }
  n740 = property class="App"(error in=w53) -> (error out=w55:errorcluster, "App.Kind"=w54:T32)  [unwired: 1 in, 1 out]
  n741 = case shown="\"Run Time System\"" w54 {
    tunnel: [w2076 w2078] -> w56
    tunnel: w55 -> [w2076 w2077]
    frame "Development System", Default {
    }
    frame "Run Time System" {
      n742 = invoke class="VI" method="FP.Close"(error in=w2077) -> (error out=w2078:errorcluster)  [unwired: 2 in, 2 out]
    }
  }
  "error out 2" <- w56
